vi "Q14070-Z060B111.vi"() -> ()   [LabVIEW 2013]
uses:
  <vilib>/Utility/file.llb/Read From Spreadsheet File (string).vi
  <vilib>/express/express arith-compare/Formula/XNode/ExpressFormulaBlockNode.xnode
  PCI8622_32.dll
  <vilib>/printing/EasyPrintingControls.llb/contents.ctl
  <vilib>/Utility/NIReport.llb/NI_ReportGenerationCore.lvlib
  <vilib>/printing/EasyPrintingControls.llb/report_type.ctl
  <vilib>/Utility/NIReport.llb/NI_report.lvclass
  <vilib>/printing/EasyPrinting.llb/Easy Print VI Panel or Documentation (path).vi
panel:
  out "左轴向力数组大小":i32
  in  "电动缸快速":dbl=15.0
  in  "电动缸慢速":dbl=1.0
  out "最大轴向力标准(N)":dbl=200.0 caption="L+Lmax(mm)" format="%#.3f"
  out "循环退出":bool
  in  "?":bool
  in  "密码":string
  in  "?":bool
  in  "?":bool
  in  "截取百分比":dbl=0.05
  in  "半行程":dbl=70.0
  in  "是否取消放行按钮":bool
  out "PLC":bool
  out "齿条传动比":dbl=200.0 caption="L+Lmax(mm)" format="%#.3f"
  out "右平均轴向力(N)":dbl caption="L+Lmax(mm)" format="%#.3f"
  out "左平均轴向力(N)":dbl caption="最大位移偏离Lmax(mm)" format="%#.3f"
  in  "确定按钮":bool
  out "员工ID":string
  in  "出支线工步号":dbl
  out "报警提示":string
  in  "报警工步号":dbl
  out "急停":bool
  out "DeviceHandle":u32
  in  "轴向力设定次数":dbl=5.0
  in  "最小间隙(mm)":dbl=0.0005 format="%#.3f"
  out "本备料状态H":bool
  out "本测试状态H":bool
  out "本自动状态H":bool
  out "夹头松开":bool
  out "测头右位":bool
  out "测头左位":bool
  in  "测头气缸右移":bool
  in  "测头气缸左移":bool
  in  "轴向力已做次数":dbl
  out "轴向力及全行程间隙合格":bool
  out "轴向力启动":bool
  out "间隙启动":bool
  out "夹头夹紧位":bool
  in  "夹头松开":bool
  in  "夹头夹紧":bool
  out "找帽扭矩":dbl=5.0 caption="压力传感器" format="%#.2f"
  out "error out":errorcluster
  out "型号数量":i32
  out "error out 4":errorcluster
  in  "间隙设定调整次数":dbl=5.0
  out "读取产品ID":string
  out "本备料状态":bool
  out "本测试状态":bool
  out "本自动状态":bool
  out "FGCS":string
  out "KSJJ":string
  out "Z060BRFID":string
  out "轴向力Y":dbl[](array[numeric])
  out "轴向力X":dbl[](array[numeric])
  out "间隙X数组":dbl[](array[numeric])
  out "间隙Y数组":dbl[](array[numeric])
  out "error out 3":errorcluster caption="错误输出"
  out "rfid工步号":u32
  out "芯片ID":string="201209190001"
  out "rfid完成":bool
  out "rfid触发":bool
  out "本序已做":bool
  in  "回零完成":bool
  in  "电动缸回零":bool
  in  "单点间隙已调试次数":dbl
  in  "需调整角度(度)":dbl
  in  "转向器中心":dbl
  out "扭矩到达":bool
  out "黄灯":bool
  out "红灯":bool
  out "基准位移":dbl caption="压力传感器" format="%#.4f"
  out "上序不合格":bool
  out "单点间隙合格":bool
  out "上序合格":bool
  out "测头机构电机":u32
  out "复位":bool
  in  "型号选择":u16(ring)=1 items=["J709", "J728", "J706"]
  in  "联线按钮":bool
  in  "工步号":u32
  in  "产品ID":string="201209190001"
  out "间隙位移(mm)":dbl=-4.6787895475327215 caption="压力传感器" format="%#.3f"
  out "齿条推拉力(N)":dbl format="%#.2f"
  out "齿条扭矩(Nm)":dbl format="%#.2f"
  out "通讯状态":bool
  out "员工姓名":string
  out "工步提示":string
  out "ADODB._Connection Out 2":refnum<k7>
  out "旋转齿条电机":u32
  out "电动缸电机":u32
  in  "停止":bool
  in  "参数加载":bool
  in  "选项卡控件":T1(tab)
  in  "180°外全行程间隙标准(mm)":dbl=0.1 format="%#.3f"
  out "扭动曲线":cluster{"Y":dbl[], "Y":dbl[]}[](graph) caption="压球涨堵头1"
  out "中间位置间隙":dbl caption="间隙值L(mm)" format="%#.3f"
  in  "中间位置最大间隙标准(mm)":dbl=0.07 format="%#.3f"
  out "右180°外全行程间隙":dbl caption="正向最大间隙L1(mm)" format="%#.3f"
  out "左180°外全行程间隙":dbl caption="正向最大间隙L1(mm)" format="%#.3f"
  out "右180°内全行程间隙":dbl caption="正向最大间隙L1(mm)" format="%#.3f"
  out "左180°内全行程间隙":dbl caption="正向最大间隙L1(mm)" format="%#.3f"
  in  "180°内全行程间隙标准(mm)":dbl=0.07 format="%#.3f"
  in  "找帽OK":bool
  out "左全行程间隙":dbl caption="正向最大间隙L1(mm)" format="%#.3f"
  out "右全行程间隙":dbl caption="正向最大间隙L1(mm)" format="%#.3f"
  out "总圈数最大值":dbl
  out "总圈数标准":dbl
  out "总行程最大值":dbl
  out "总行程标准(mm)":dbl
  out "力波动标准(N)":dbl=60.0 caption="L+Lmax(mm)" format="%#.3f"
  out "轴向力标准(N)":dbl=100.0 caption="L+Lmax(mm)" format="%#.3f"
  out "右轴向力波动(N)":dbl caption="L+Lmax(mm)" format="%_4g"
  out "右最大轴向力(N)":dbl caption="L+Lmax(mm)" format="%_4g"
  out "左轴向力波动(N)":dbl caption="最大位移偏离Lmax(mm)" format="%_4g"
  out "左最大轴向力(N)":dbl caption="最大位移偏离Lmax(mm)" format="%_4g"
  out "行程跳动曲线":cluster{"Y":dbl[], "Y":dbl[]}[](graph) caption="压球涨堵头1"
  out "平均轴向力标准(N) max":dbl=200.0 caption="L+Lmax(mm)" format="%#.3f"
  out "总行程":dbl format="%_4g"
  out "总圈数":dbl format="%_4g"
  in  "不合格品":bool
  in  "扭矩停止值":dbl=16.0
  in  "齿条右极限":dbl=-70.0 caption="压力传感器" format="%#.2f"
  in  "齿条左极限":dbl=-262.0 caption="压力传感器" format="%#.2f"
  in  "齿条移动速度":dbl=5.0 caption="压力传感器" format="%#.2f"
  in  "旋转齿条轴找帽转速":dbl=5.0 caption="压力传感器" format="%#.2f"
  in  "测量点扭矩":dbl=4.0 caption="压力传感器" format="%#.2f"
  in  "旋转齿条轴测量转速":dbl caption="压力传感器" format="%#.2f"
  in  "测头机构轴后退位":dbl=30.0 caption="压力传感器" format="%#.2f"
  in  "测头机构轴待检位":dbl caption="压力传感器" format="%#.2f"
  in  "测头机构轴检测位":dbl caption="压力传感器" format="%#.2f"
  in  "测头机构轴移动速度":dbl caption="压力传感器" format="%#.2f"
  in  "机械间隙值":dbl=3.5
  in  "阻挡":bool
  in  "放行":bool
  in  "夹头松开":bool
  in  "夹头夹紧":bool
  in  "测头气缸右移":bool
  in  "测头气缸左移":bool
  in  "支线下降":bool
  in  "支线顶升":bool
  in  "出支线":bool
  in  "进支线":bool
  in  "主线下降":bool
  in  "主线顶升":bool
  in  "下阻挡器放行":bool
  in  "上阻挡器放行":bool
  in  "测头机构轴使能":bool
  in  "测头机构轴后退":bool
  in  "测头机构轴前进":bool
  in  "电动缸速度(mm/s)":dbl=10.0 format="%#.3f"
  out "电动缸位置(mm)":dbl format="%#.3f"
  in  "旋转齿条轴速度(°/s)":dbl=10.0 format="%#.3f"
  out "旋转齿条轴位置(°)":dbl format="%#.3f"
  in  "测头机构轴速度(mm/s)":dbl=10.0 format="%#.3f"
  out "测头机构轴位置(mm)":dbl format="%#.3f"
  in  "旋转齿条轴右转":bool
  in  "旋转齿条轴左转":bool
  in  "旋转齿条轴使能":bool
  in  "电动缸后退":bool
  in  "电动缸使能":bool
  in  "电动缸前进":bool
  in  "齿条扭矩比例偏移":dbl=1.0 format="%#.2f"
  in  "齿条扭矩零点偏移":dbl format="%#.2f"
  in  "齿条推拉力比例偏移":dbl=1.0 format="%#.2f"
  in  "齿条推拉力零点偏移":dbl format="%#.2f"
  in  "间隙位移比例偏移":dbl=1.0 format="%#.2f"
  in  "间隙位移零点偏移":dbl format="%#.2f"
  in  "传感器参数保存":bool
  in  "参数修改":bool
  in  "参数查询":bool
  in  "参数浏览表":string[][](table)
  # "芜湖机械转向器装配线"
  # "间隙及轴向力检测"
  # "湖北唯思凌科装备制造有限公司 设计开发 (C)2015"
  # "Q14070机械转向器装配线"
  # "≤"
  # "间隙测量结果"
  # "间隙测量判定值"
  # "≤"
  # "≤"
  # "≤"
  # "轴向力测量结果"
  # "轴向力测量标准"
  # "≥"
  # "≤"
  # "≥"
  # "≤"
  # "≤"
  # "≥"
  # "不得大于20NM"
  # "传感器校验区"
  # "关于传感器校验：\n1、传感器校验需要由具备资质的单位或部门进行校验。\n2、具备权限的用户才能够修改传感器校验参数和试验参数。\n3、修改校验参数方法：先将比例偏移置为1，修改零点偏移，使零点值与校验的传感器一致；然后根据增幅调整比例偏移。"
  # "注意：\n具备权限的用户才能够修改传感器校验参数和试验参数！"
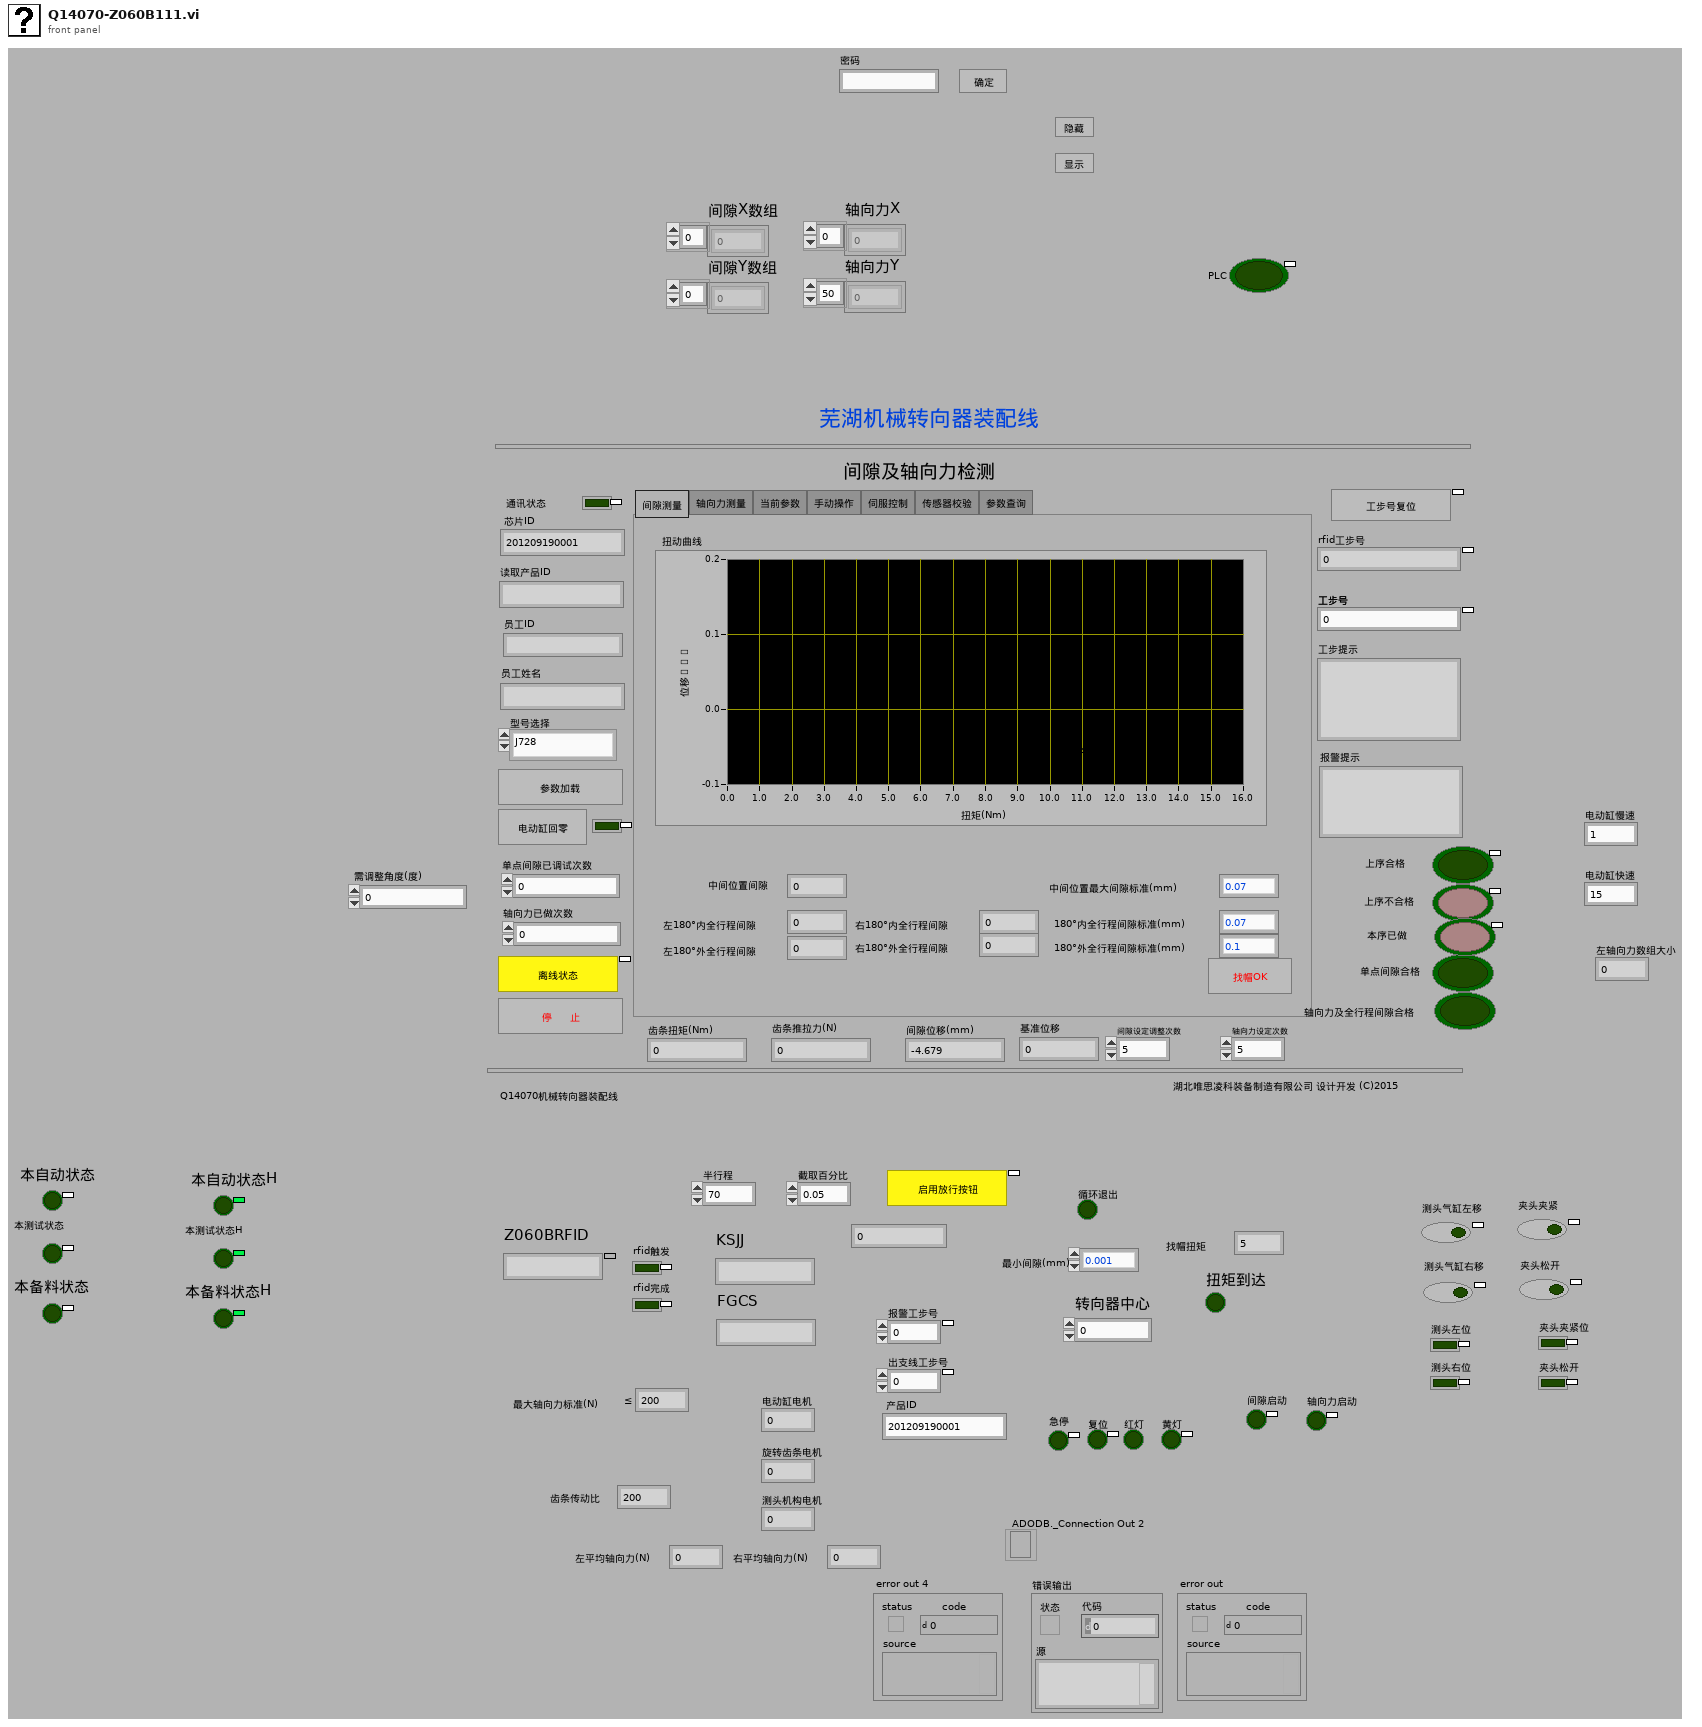
[diagram p1: front panel]
types:
  T1 = enum32{"间隙测量", "轴向力测量", "当前参数", "手动操作", "伺服控制", "传感器校验", "参数查询"}
  T2 = typedef "NI_ReportGenerationCore.lvlib/report_type.ctl" = u16
  T3 = typedef "NI_ReportGenerationCore.lvlib/contents.ctl" = u16
  T4 = typedef "imagedata.ctl" = cluster{"image type":i32, "image depth":i32, "image":u8[], "mask":u8[], "colors":u32[], "Rectangle":cluster{"left":i16, "top":i16, "right":i16, "bottom":i16}}
  T5 = enum8{"Enabled", "Disabled", "Disabled and Grayed Out"}
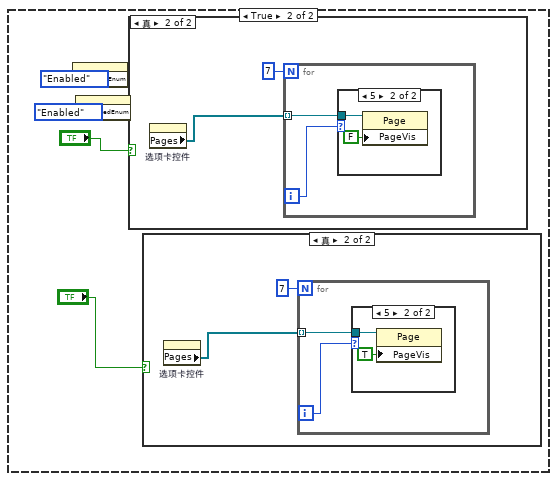
[diagram p2: hidden frame]
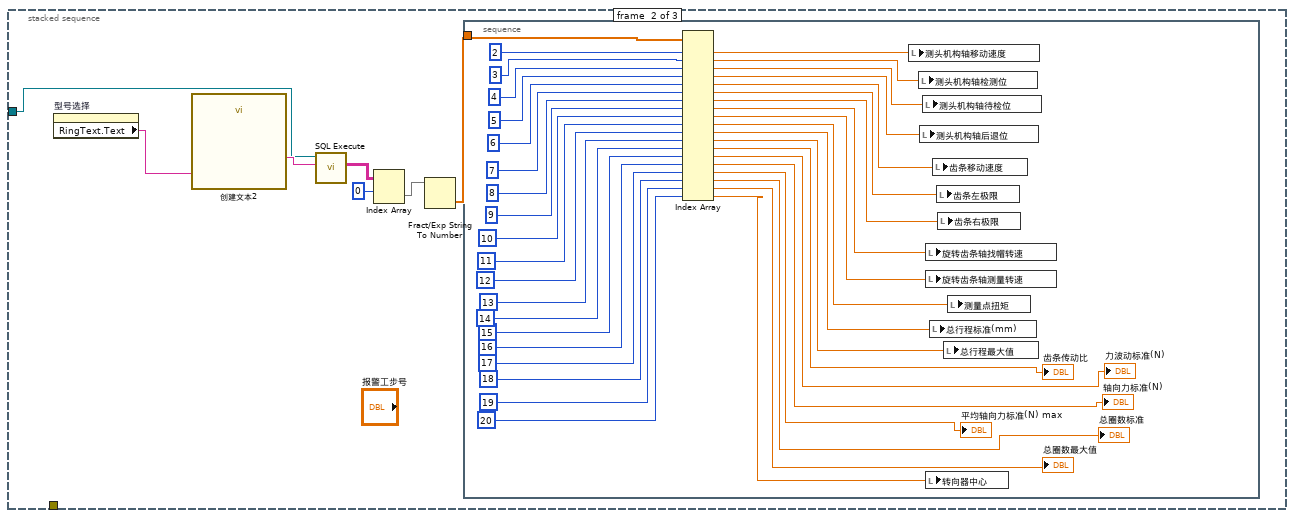
[diagram p9: hidden frame]
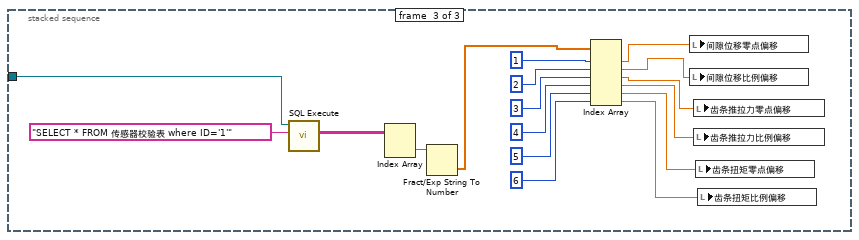
[diagram p10: hidden frame]
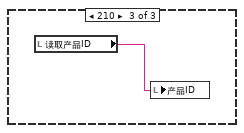
[diagram p12: hidden frame]
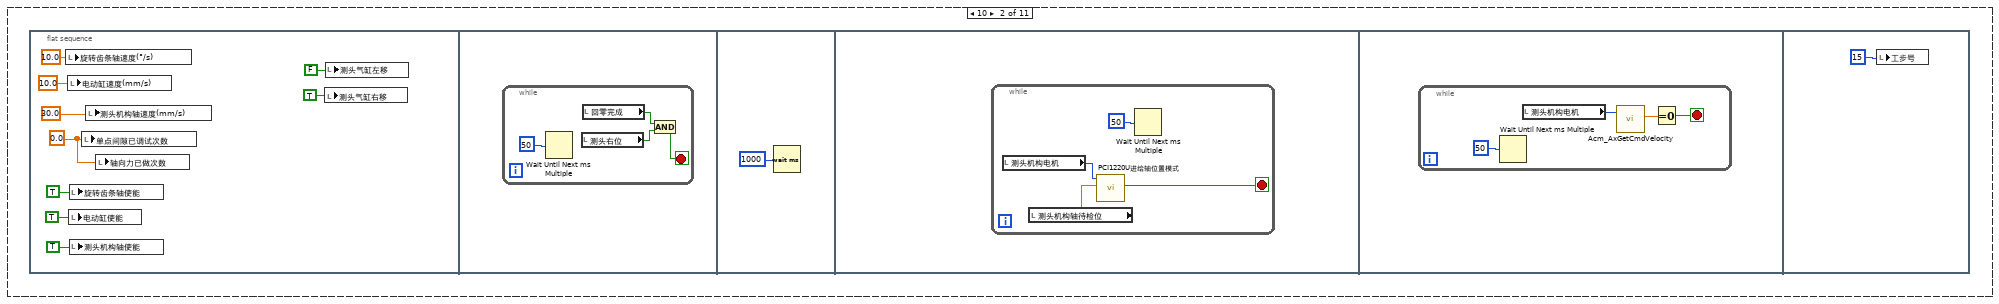
[diagram p14: hidden frame]
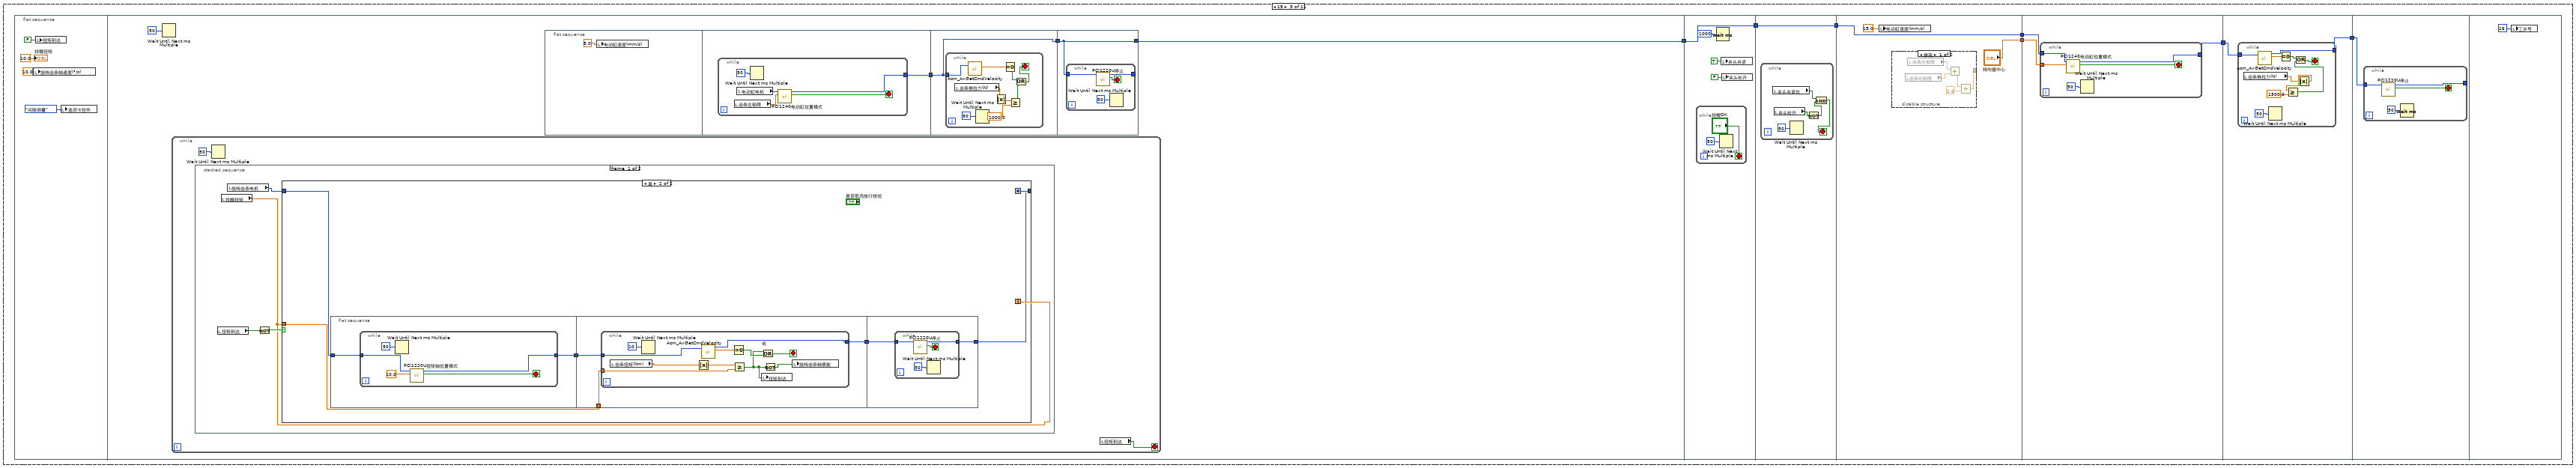
[diagram p15: hidden frame]
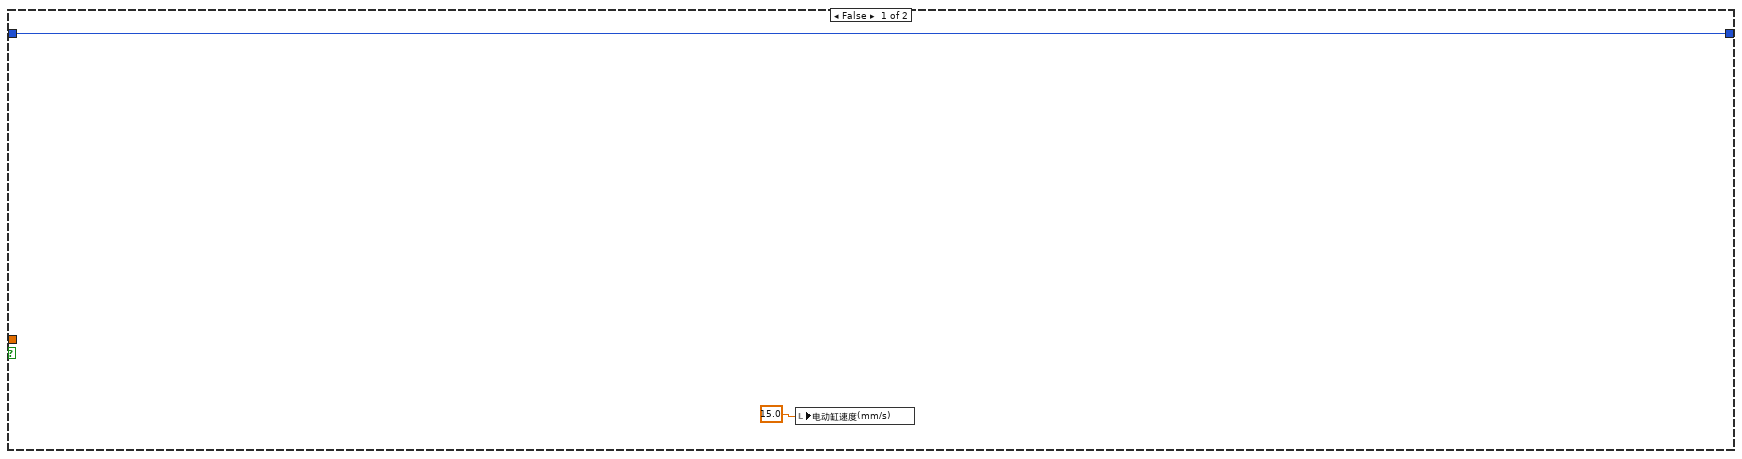
[diagram p16: hidden frame]
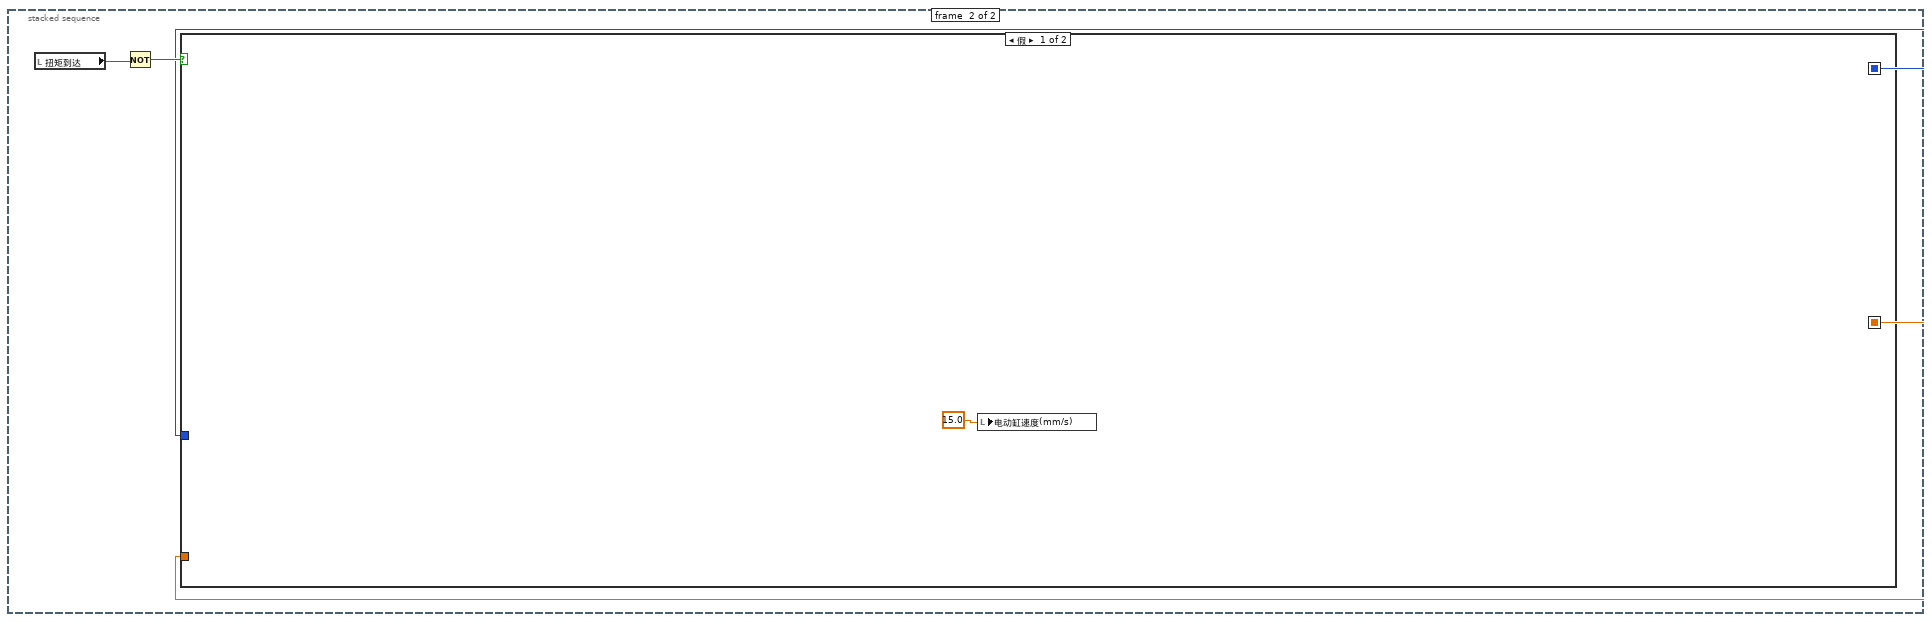
[diagram p17: hidden frame]
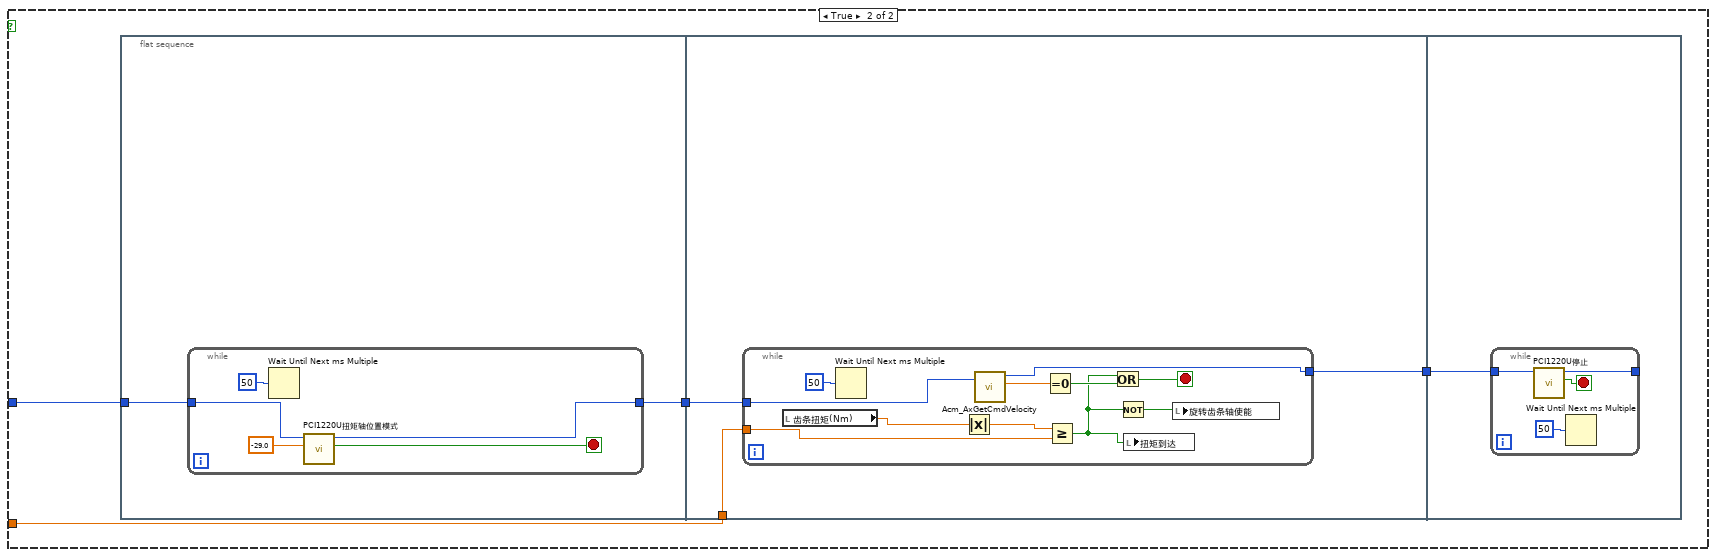
[diagram p18: hidden frame]
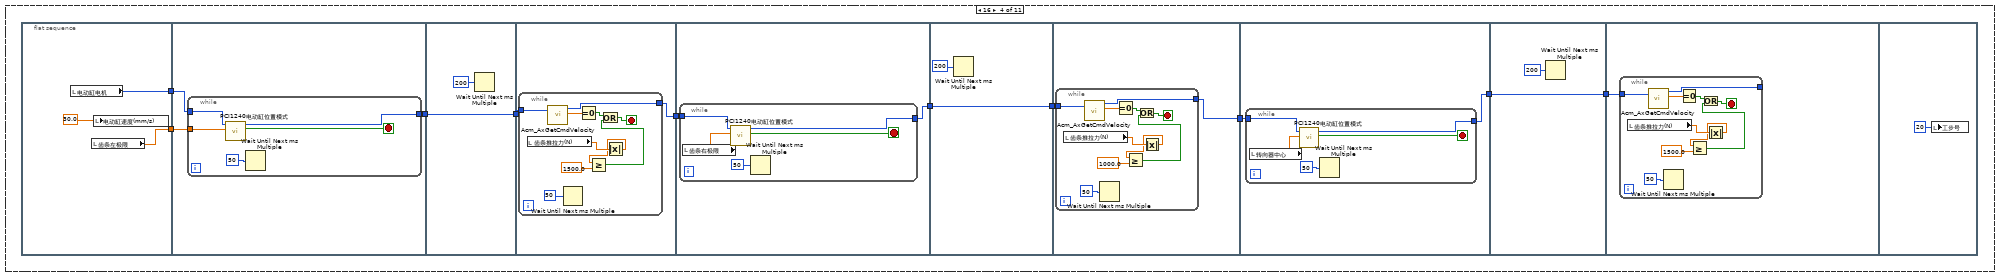
[diagram p20: hidden frame]
diagram:
  n1 = while {
    stop <- w7 stop-if-true
    n2 = local read "工步号"() -> (w5:u32)
    n3 = case shown="40" w5 {
      frame 0, Default {
      }
      frame 10 {
        n4 = flat-sequence {
          frame #0 {
            w8 = 0.0 ("已调试次数")
            n5 = local write "旋转齿条轴速度(°/s)"(10.0 ("旋转齿条轴速度(°/s)")) -> ()
            n6 = local write "电动缸速度(mm/s)"(10.0 ("电动缸速度(mm/s)")) -> ()
            n7 = local write "电动缸使能"(TRUE ("电动缸使能")) -> ()
            n8 = local write "旋转齿条轴使能"(TRUE ("旋转齿条轴使能")) -> ()
            n9 = local write "测头机构轴使能"(TRUE ("调整机构轴使能")) -> ()
            n10 = local write "单点间隙已调试次数"(w8) -> ()
            n11 = local write "测头机构轴速度(mm/s)"(30.0 ("调整机构轴速度(mm/s)")) -> ()
            n12 = local write "轴向力已做次数"(w8) -> ()
            n13 = local write "测头气缸右移"(TRUE ("测头气缸右移")) -> ()
            n14 = local write "测头气缸左移"(FALSE ("测头气缸左移")) -> ()
          }
          frame #1 {
            n15 = while {
              stop <- w17 stop-if-true
              n16 = Wait Until Next ms Multiple(millisecond multiple=u32 50 ("毫秒倍数")) -> ()  [unwired: 1 out]
              n17 = local read "测头右位"() -> (w18:bool)
              n18 = local read "回零完成"() -> (w19:bool)
              n19 = And(x=w19, y=w18) -> (x .and. y?=w17:bool)
            }
          }
          frame #2 {
            n20 = Wait (ms)(milliseconds to wait=u32 1000 ("等待时间（毫秒）")) -> ()  [unwired: 1 out]
          }
          frame #3 {
            n21 = while {
              stop <- w25 stop-if-true
              n22 = local read "测头机构电机"() -> (w23:u32)
              n23 = local read "测头机构轴待检位"() -> (w22:dbl)
              n24 = call "PCI1220U进给轴位置模式.vi"("Distance"=w22, "AxisHandle IN"=w23) -> ("AbsSuccess"=w25:bool)  [unwired: 8 in, 1 out]
              n25 = Wait Until Next ms Multiple(millisecond multiple=u32 50 ("毫秒倍数")) -> ()  [unwired: 1 out]
            }
          }
          frame #4 {
            n26 = while {
              stop <- w28 stop-if-true
              n27 = Wait Until Next ms Multiple(millisecond multiple=u32 50 ("毫秒倍数")) -> ()  [unwired: 1 out]
              n28 = local read "测头机构电机"() -> (w26:u32)
              n29 = call <userlib>:"Acm_AxGetCmdVelocity.vi"("AxisHandle"=w26) -> ("Velocity"=w29:dbl)  [unwired: 1 in, 3 out]
              n30 = Equal To 0?(x=w29) -> (x = 0?=w28:bool)
            }
          }
          frame #5 {
            n31 = local write "工步号"(u32 15 ("工步号")) -> ()
          }
        }
      }
      frame 15 {
        n32 = flat-sequence {
          tunnel: [w43] -> w34
          tunnel: w34 -> [w146]
          tunnel: [w146] -> w32
          tunnel: w32 -> [w150]
          tunnel: [w150] -> w31
          tunnel: [w157] -> w37
          tunnel: ["转向器中心"] -> w36
          tunnel: w31 -> [w157]
          tunnel: w37 -> [w166]
          tunnel: w36 -> [w165]
          tunnel: [w164] -> w35
          tunnel: w35 -> [w173]
          tunnel: [w172] -> w33
          tunnel: w33 -> [w184]
          frame #0 {
            n33 = local write "旋转齿条轴速度(°/s)"(10.0 ("旋转齿条轴速度(°/s)")) -> ()
            n34 = local write "扭矩到达"(FALSE ("扭矩到达")) -> ()
            n35 = local write "选项卡控件"(T1."间隙测量" ("选项卡控件")) -> ()
            "找帽扭矩" <- 10.0 ("找帽扭矩")
          }
          frame #1 {
            n36 = Wait Until Next ms Multiple(millisecond multiple=u32 50 ("毫秒倍数")) -> ()  [unwired: 1 out]
            n37 = while {
              stop <- w46 stop-if-true
              n38 = stacked-sequence {
                seq-local: [w48 _] -> [_ w89]
                seq-local: [w52 _] -> [_ w88]
                frame #0 {
                  n39 = local read "扭矩到达"() -> (w50:bool)
                  n40 = local read "找帽扭矩"() -> (w48:dbl)
                  n41 = local read "旋转齿条电机"() -> (w49:u32)
                  n42 = Not(x=w50) -> (.not. x?=w51:bool)
                  n43 = case shown="真" w51 {
                    tunnel: [w54 w55] -> w52
                    tunnel: w49 -> [w54 w59]
                    tunnel: w48 -> [_ w57]
                    frame False {
                      n44 = local write "电动缸速度(mm/s)"(15.0 ("电动缸速度(mm/s)")) -> ()
                    }
                    frame True {
                      n45 = flat-sequence {
                        tunnel: w59 -> [w61]
                        tunnel: [w60] -> w58
                        tunnel: w58 -> [w69]
                        tunnel: w57 -> [w68]
                        tunnel: [w67] -> w56
                        tunnel: w56 -> [w82]
                        tunnel: [w81] -> w55
                        frame #0 {
                          n46 = while {
                            tunnel: [w65] -> w60
                            tunnel: w61 -> [w62]
                            stop <- w64 stop-if-true
                            n47 = Wait Until Next ms Multiple(millisecond multiple=u32 50 ("毫秒倍数")) -> ()  [unwired: 1 out]
                            n48 = call "PCI1220U扭矩轴位置模式.vi"("Distance"=10.0, "AxisHandle IN"=w62) -> ("AbsSuccess"=w64:bool, "AxisHandle OUT"=w65:u32)  [unwired: 8 in]
                          }
                        }
                        frame #1 {
                          n49 = while {
                            tunnel: w69 -> [w79]
                            tunnel: w68 -> [w74]
                            tunnel: [w73] -> w67
                            stop <- w75 stop-if-true
                            n50 = local read "齿条扭矩(Nm)"() -> (w72:dbl)
                            n51 = Wait Until Next ms Multiple(millisecond multiple=u32 10 ("毫秒倍数")) -> ()  [unwired: 1 out]
                            n52 = Absolute Value(x=w72) -> (abs(x)=w77:dbl)
                            n53 = call <userlib>:"Acm_AxGetCmdVelocity.vi"("AxisHandle"=w79) -> ("Velocity"=w78:dbl, "AxisHandle"=w73:u32)  [unwired: 1 in, 2 out]
                            n54 = Equal To 0?(x=w78) -> (x = 0?=w76:bool)
                            n55 = Greater Or Equal?(x=w77, y=w74) -> (x >= y?=w71:bool)
                            n56 = Or "或"(x=w71, y=w76) -> (x .or. y?=w75:bool)
                            n57 = local write "扭矩到达"(w71) -> ()
                            n58 = Not(x=w71) -> (.not. x?=w70:bool)
                            n59 = local write "旋转齿条轴使能"(w70) -> ()
                          }
                        }
                        frame #2 {
                          n60 = while {
                            tunnel: w82 -> [w86]
                            tunnel: [w83] -> w81
                            stop <- w85 stop-if-true
                            n61 = call "PCI1220U停止.vi"("AxisHandle IN"=w86) -> ("完成"=w85:bool, "AxisHandle OUT"=w83:u32)  [unwired: 9 in]
                            n62 = Wait Until Next ms Multiple(millisecond multiple=u32 50 ("毫秒倍数")) -> ()  [unwired: 1 out]
                          }
                        }
                      }
                    }
                  }
                }
                frame #1 {
                  n63 = local read "扭矩到达"() -> (w87:bool)
                  n64 = Not(x=w87) -> (.not. x?=w90:bool)
                  n65 = case shown="假" w90 {
                    tunnel: w88 -> [_ w95]
                    tunnel: w89 -> [_ w93]
                    frame False {
                      n66 = local write "电动缸速度(mm/s)"(15.0 ("电动缸速度(mm/s)")) -> ()
                    }
                    frame True {
                      n67 = flat-sequence {
                        tunnel: w95 -> [w96]
                        tunnel: [w97] -> w94
                        tunnel: w94 -> [w105]
                        tunnel: w93 -> [w104]
                        tunnel: [w103] -> w92
                        tunnel: w92 -> [w117]
                        frame #0 {
                          n68 = while {
                            tunnel: [w101] -> w97
                            tunnel: w96 -> [w98]
                            stop <- w100 stop-if-true
                            n69 = Wait Until Next ms Multiple(millisecond multiple=u32 50 ("毫秒倍数")) -> ()  [unwired: 1 out]
                            n70 = call "PCI1220U扭矩轴位置模式.vi"("Distance"=-29.0, "AxisHandle IN"=w98) -> ("AbsSuccess"=w100:bool, "AxisHandle OUT"=w101:u32)  [unwired: 8 in]
                          }
                        }
                        frame #1 {
                          n71 = while {
                            tunnel: w105 -> [w115]
                            tunnel: [w110] -> w103
                            tunnel: w104 -> [w109]
                            stop <- w111 stop-if-true
                            n72 = local read "齿条扭矩(Nm)"() -> (w108:dbl)
                            n73 = Wait Until Next ms Multiple(millisecond multiple=u32 50 ("毫秒倍数")) -> ()  [unwired: 1 out]
                            n74 = Absolute Value(x=w108) -> (abs(x)=w113:dbl)
                            n75 = call <userlib>:"Acm_AxGetCmdVelocity.vi"("AxisHandle"=w115) -> ("Velocity"=w114:dbl, "AxisHandle"=w110:u32)  [unwired: 1 in, 2 out]
                            n76 = Equal To 0?(x=w114) -> (x = 0?=w112:bool)
                            n77 = Greater Or Equal?(x=w113, y=w109) -> (x >= y?=w106:bool)
                            n78 = Or(x=w106, y=w112) -> (x .or. y?=w111:bool)
                            n79 = Not(x=w106) -> (.not. x?=w107:bool)
                            n80 = local write "扭矩到达"(w106) -> ()
                            n81 = local write "旋转齿条轴使能"(w107) -> ()
                          }
                        }
                        frame #2 {
                          n82 = while {
                            tunnel: w117 -> [w121]
                            tunnel: [w118] -> _
                            stop <- w120 stop-if-true
                            n83 = call "PCI1220U停止.vi"("AxisHandle IN"=w121) -> ("完成"=w120:bool, "AxisHandle OUT"=w118:u32)  [unwired: 9 in]
                            n84 = Wait Until Next ms Multiple(millisecond multiple=u32 50 ("毫秒倍数")) -> ()  [unwired: 1 out]
                          }
                        }
                      }
                    }
                  }
                }
              }
              n85 = Wait Until Next ms Multiple(millisecond multiple=u32 50 ("毫秒倍数")) -> ()  [unwired: 1 out]
              n86 = local read "扭矩到达"() -> (w46:bool)
            }
            n87 = flat-sequence {
              tunnel: [w123] -> w45
              tunnel: w45 -> [w129]
              tunnel: [w129] -> w42
              tunnel: [w139] -> w43
              tunnel: w42 -> [w139]
              frame #0 {
                n88 = local write "电动缸速度(mm/s)"(5.0 ("电动缸速度(mm/s)")) -> ()
              }
              frame #1 {
                n89 = while {
                  tunnel: [w127] -> w123
                  stop <- w126 stop-if-true
                  n90 = local read "齿条左极限"() -> (w124:dbl)
                  n91 = local read "电动缸电机"() -> (w128:u32)
                  n92 = Wait Until Next ms Multiple(millisecond multiple=u32 50 ("毫秒倍数")) -> ()  [unwired: 1 out]
                  n93 = call "PCI1240电动缸位置模式 .vi"("Distance"=w124, "AxisHandle IN"=w128) -> ("AbsSuccess"=w126:bool, "AxisHandle OUT"=w127:u32)  [unwired: 8 in]
                }
              }
              frame #2 {
                n94 = while {
                  tunnel: w129 -> [w137]
                  stop <- w134 stop-if-true
                  n95 = local read "齿条推拉力(N)"() -> (w133:dbl)
                  n96 = call <userlib>:"Acm_AxGetCmdVelocity.vi"("AxisHandle"=w137) -> ("Velocity"=w138:dbl)  [unwired: 1 in, 3 out]
                  n97 = Wait Until Next ms Multiple(millisecond multiple=u32 50 ("毫秒倍数")) -> ()  [unwired: 1 out]
                  n98 = Absolute Value(x=w133) -> (abs(x)=w130:dbl)
                  n99 = Equal To 0?(x=w138) -> (x = 0?=w135:bool)
                  n100 = Greater Or Equal?(x=w130, y=1000.0) -> (x >= y?=w131:bool)
                  n101 = Or(x=w135, y=w131) -> (x .or. y?=w134:bool)
                }
              }
              frame #3 {
                n102 = while {
                  tunnel: w139 -> [w143]
                  tunnel: [w140] -> _
                  stop <- w142 stop-if-true
                  n103 = call "PCI1220U停止.vi"("AxisHandle IN"=w143) -> ("完成"=w142:bool, "AxisHandle OUT"=w140:u32)  [unwired: 9 in]
                  n104 = Wait Until Next ms Multiple(millisecond multiple=u32 50 ("毫秒倍数")) -> ()  [unwired: 1 out]
                }
              }
            }
          }
          frame #2 {
            n105 = while {
              stop <- "找帽OK" stop-if-true
              n106 = Wait Until Next ms Multiple(millisecond multiple=u32 50 ("毫秒倍数")) -> ()  [unwired: 1 out]
            }
            n107 = Wait (ms)(milliseconds to wait=u32 1000 ("毫秒倍数")) -> ()  [unwired: 1 out]
            n108 = local write "夹头夹紧"(TRUE ("夹头夹紧")) -> ()
            n109 = local write "夹头松开"(FALSE ("夹头松开")) -> ()
          }
          frame #3 {
            n110 = while {
              stop <- w152 stop-if-true
              n111 = local read "夹头夹紧位"() -> (w153:bool)
              n112 = local read "夹头松开"() -> (w155:bool)
              n113 = Wait Until Next ms Multiple(millisecond multiple=u32 50 ("毫秒倍数")) -> ()  [unwired: 1 out]
              n114 = Not(x=w155) -> (.not. x?=w154:bool)
              n115 = And(x=w153, y=w154) -> (x .and. y?=w152:bool)
            }
          }
          frame #4 {
            n116 = local write "电动缸速度(mm/s)"(15.0 ("电动缸轴移动速度")) -> ()
            n117 = disable-structure shown="禁用" {
              disable-tunnel: [w159 _] -> _
              frame Disabled {
                n118 = local read "齿条右极限"() -> (w162:dbl)
                n119 = local read "齿条左极限"() -> (w163:dbl)
                n120 = Add(x=w163, y=w162) -> (x+y=w161:dbl)
                n121 = Divide(x=w161, y=2.0) -> (x/y=w159:dbl)
              }
              frame Enabled {
              }
            }
          }
          frame #5 {
            n122 = while {
              tunnel: w166 -> [w171]
              tunnel: w165 -> [w170]
              tunnel: [w167] -> w164
              stop <- w169 stop-if-true
              n123 = call "PCI1240电动缸位置模式 .vi"("Distance"=w170, "AxisHandle IN"=w171) -> ("AbsSuccess"=w169:bool, "AxisHandle OUT"=w167:u32)  [unwired: 8 in]
              n124 = Wait Until Next ms Multiple(millisecond multiple=u32 50 ("毫秒倍数")) -> ()  [unwired: 1 out]
            }
          }
          frame #6 {
            n125 = while {
              tunnel: w173 -> [w183]
              tunnel: [w174] -> w172
              stop <- w175 stop-if-true
              n126 = local read "齿条推拉力(N)"() -> (w180:dbl)
              n127 = call <userlib>:"Acm_AxGetCmdVelocity.vi"("AxisHandle"=w183) -> ("Velocity"=w182:dbl, "AxisHandle"=w174:u32)  [unwired: 1 in, 2 out]
              n128 = Wait Until Next ms Multiple(millisecond multiple=u32 50 ("毫秒倍数")) -> ()  [unwired: 1 out]
              n129 = Equal To 0?(x=w182) -> (x = 0?=w177:bool)
              n130 = Absolute Value(x=w180) -> (abs(x)=w179:dbl)
              n131 = Greater Or Equal?(x=w179, y=1500.0) -> (x >= y?=w176:bool)
              n132 = Or(x=w177, y=w176) -> (x .or. y?=w175:bool)
            }
          }
          frame #7 {
            n133 = while {
              tunnel: w184 -> [w188]
              tunnel: [w187] -> _
              stop <- w186 stop-if-true
              n134 = call "PCI1220U停止.vi"("AxisHandle IN"=w188) -> ("完成"=w186:bool, "AxisHandle OUT"=w187:u32)  [unwired: 9 in]
              n135 = Wait (ms)(milliseconds to wait=u32 50 ("毫秒倍数")) -> ()  [unwired: 1 out]
            }
          }
          frame #8 {
            n136 = local write "工步号"(u32 16 ("工步号")) -> ()
          }
        }
      }
      frame 16 {
        n137 = flat-sequence {
          tunnel: [w202] -> w199
          tunnel: [w201] -> w198
          tunnel: w199 -> [w205]
          tunnel: w198 -> [w204]
          tunnel: [w203] -> w197
          tunnel: w197 -> [w212]
          tunnel: [w212] -> w196
          tunnel: w196 -> [w214]
          tunnel: [w213] -> w195
          tunnel: w195 -> [w226]
          tunnel: [w225] -> w193
          tunnel: [w232] -> w194
          tunnel: w193 -> [w232]
          tunnel: w194 -> [w235]
          tunnel: [w234] -> w192
          tunnel: w192 -> [w247]
          tunnel: [w246] -> w190
          tunnel: [w253] -> w191
          tunnel: w190 -> [w253]
          tunnel: w191 -> [w255]
          frame #0 {
            n138 = local read "电动缸电机"() -> (w202:u32)
            n139 = local read "齿条左极限"() -> (w201:dbl)
            n140 = local write "电动缸速度(mm/s)"(30.0 ("齿条移动速度")) -> ()
          }
          frame #1 {
            n141 = while {
              tunnel: w205 -> [w210]
              tunnel: w204 -> [w209]
              tunnel: [w206] -> w203
              stop <- w208 stop-if-true
              n142 = call "PCI1240电动缸位置模式 .vi"("Distance"=w209, "AxisHandle IN"=w210) -> ("AbsSuccess"=w208:bool, "AxisHandle OUT"=w206:u32)  [unwired: 8 in]
              n143 = Wait Until Next ms Multiple(millisecond multiple=u32 50 ("毫秒倍数")) -> ()  [unwired: 1 out]
            }
          }
          frame #2 {
            n144 = Wait Until Next ms Multiple(millisecond multiple=u32 200 ("毫秒倍数")) -> ()  [unwired: 1 out]
          }
          frame #3 {
            n145 = while {
              tunnel: w214 -> [w224]
              tunnel: [w215] -> w213
              stop <- w216 stop-if-true
              n146 = local read "齿条推拉力(N)"() -> (w221:dbl)
              n147 = call <userlib>:"Acm_AxGetCmdVelocity.vi"("AxisHandle"=w224) -> ("Velocity"=w223:dbl, "AxisHandle"=w215:u32)  [unwired: 1 in, 2 out]
              n148 = Wait Until Next ms Multiple(millisecond multiple=u32 50 ("毫秒倍数")) -> ()  [unwired: 1 out]
              n149 = Equal To 0?(x=w223) -> (x = 0?=w218:bool)
              n150 = Absolute Value(x=w221) -> (abs(x)=w220:dbl)
              n151 = Greater Or Equal?(x=w220, y=1500.0) -> (x >= y?=w217:bool)
              n152 = Or(x=w218, y=w217) -> (x .or. y?=w216:bool)
            }
          }
          frame #4 {
            n153 = while {
              tunnel: w226 -> [w231]
              tunnel: [w228] -> w225
              stop <- w230 stop-if-true
              n154 = local read "齿条右极限"() -> (w227:dbl)
              n155 = call "PCI1240电动缸位置模式 .vi"("Distance"=w227, "AxisHandle IN"=w231) -> ("AbsSuccess"=w230:bool, "AxisHandle OUT"=w228:u32)  [unwired: 8 in]
              n156 = Wait Until Next ms Multiple(millisecond multiple=u32 50 ("毫秒倍数")) -> ()  [unwired: 1 out]
            }
          }
          frame #5 {
            n157 = Wait Until Next ms Multiple(millisecond multiple=u32 200 ("毫秒倍数")) -> ()  [unwired: 1 out]
          }
          frame #6 {
            n158 = while {
              tunnel: w235 -> [w245]
              tunnel: [w236] -> w234
              stop <- w237 stop-if-true
              n159 = local read "齿条推拉力(N)"() -> (w242:dbl)
              n160 = call <userlib>:"Acm_AxGetCmdVelocity.vi"("AxisHandle"=w245) -> ("Velocity"=w244:dbl, "AxisHandle"=w236:u32)  [unwired: 1 in, 2 out]
              n161 = Wait Until Next ms Multiple(millisecond multiple=u32 50 ("毫秒倍数")) -> ()  [unwired: 1 out]
              n162 = Equal To 0?(x=w244) -> (x = 0?=w239:bool)
              n163 = Absolute Value(x=w242) -> (abs(x)=w241:dbl)
              n164 = Greater Or Equal?(x=w241, y=1000.0) -> (x >= y?=w238:bool)
              n165 = Or(x=w239, y=w238) -> (x .or. y?=w237:bool)
            }
          }
          frame #7 {
            n166 = while {
              tunnel: w247 -> [w252]
              tunnel: [w249] -> w246
              stop <- w251 stop-if-true
              n167 = local read "转向器中心"() -> (w248:dbl)
              n168 = call "PCI1240电动缸位置模式 .vi"("Distance"=w248, "AxisHandle IN"=w252) -> ("AbsSuccess"=w251:bool, "AxisHandle OUT"=w249:u32)  [unwired: 8 in]
              n169 = Wait Until Next ms Multiple(millisecond multiple=u32 50 ("毫秒倍数")) -> ()  [unwired: 1 out]
            }
          }
          frame #8 {
            n170 = Wait Until Next ms Multiple(millisecond multiple=u32 200 ("毫秒倍数")) -> ()  [unwired: 1 out]
          }
          frame #9 {
            n171 = while {
              tunnel: w255 -> [w265]
              tunnel: [w256] -> _
              stop <- w257 stop-if-true
              n172 = local read "齿条推拉力(N)"() -> (w262:dbl)
              n173 = call <userlib>:"Acm_AxGetCmdVelocity.vi"("AxisHandle"=w265) -> ("Velocity"=w264:dbl, "AxisHandle"=w256:u32)  [unwired: 1 in, 2 out]
              n174 = Wait Until Next ms Multiple(millisecond multiple=u32 50 ("毫秒倍数")) -> ()  [unwired: 1 out]
              n175 = Equal To 0?(x=w264) -> (x = 0?=w259:bool)
              n176 = Absolute Value(x=w262) -> (abs(x)=w261:dbl)
              n177 = Greater Or Equal?(x=w261, y=1500.0) -> (x >= y?=w258:bool)
              n178 = Or(x=w259, y=w258) -> (x .or. y?=w257:bool)
            }
          }
          frame #10 {
            n179 = local write "工步号"(u32 20 ("工步号")) -> ()
          }
        }
      }
      frame 20 {
        n180 = flat-sequence {
          tunnel: [w295] -> w276
          tunnel: w276 -> [w301]
          tunnel: [w308] -> w272
          tunnel: w272 -> [w315]
          tunnel: [w315] -> w271
          tunnel: w271 -> [w323]
          tunnel: [w323] -> w270
          tunnel: w270 -> [w324]
          tunnel: [w330] -> w274
          tunnel: [w332] -> w275
          tunnel: w274 -> [w332]
          tunnel: [w334] -> w281
          tunnel: w275 -> [w334]
          tunnel: w281 -> [w341]
          tunnel: [w340] -> w280
          tunnel: [w345] -> w279
          tunnel: [w344] -> w278
          tunnel: w280 -> [w343]
          tunnel: [w343] -> w277
          tunnel: [w372] -> w284
          tunnel: [w369] -> w283
          tunnel: w279 -> [w369]
          tunnel: [w368] -> w282
          tunnel: w278 -> [w368]
          tunnel: w277 -> [w372]
          tunnel: w284 -> [w376]
          tunnel: [w375] -> w273
          tunnel: w283 -> [w373]
          tunnel: w282 -> [w374]
          tunnel: w273 -> [w382]
          tunnel: [w381] -> w268
          tunnel: w268 -> [w389]
          tunnel: [w389] -> w267
          tunnel: w267 -> [w391]
          tunnel: [w390] -> w269
          tunnel: w269 -> [w401]
          frame #0 {
            n181 = local write "选项卡控件"(T1."间隙测量" ("选项卡控件")) -> ()
          }
          frame #1 {
            n182 = while {
              stop <- w286 stop-if-true
              n183 = local read "夹头松开"() -> (w288:bool)
              n184 = local read "夹头夹紧位"() -> (w287:bool)
              n185 = Wait Until Next ms Multiple(millisecond multiple=u32 50 ("毫秒倍数")) -> ()  [unwired: 1 out]
              n186 = Not(x=w288) -> (.not. x?=w289:bool)
              n187 = And(x=w287, y=w289) -> (x .and. y?=w286:bool)
            }
          }
          frame #2 {
            n188 = local read "转向器中心"() -> (w291:dbl)
            n189 = local read "电动缸电机"() -> (w294:u32)
            n190 = Add(x=w291, y=0.0) -> (x+y=w293:dbl)
            n191 = while {
              tunnel: w294 -> [w300]
              tunnel: w293 -> [w299]
              tunnel: [w296] -> w295
              stop <- w298 stop-if-true
              n192 = call "PCI1240电动缸位置模式 .vi"("Distance"=w299, "AxisHandle IN"=w300) -> ("AbsSuccess"=w298:bool, "AxisHandle OUT"=w296:u32)  [unwired: 8 in]
              n193 = Wait Until Next ms Multiple(millisecond multiple=u32 50 ("毫秒倍数")) -> ()  [unwired: 1 out]
            }
          }
          frame #3 {
            n194 = while {
              tunnel: w301 -> [w305]
              stop <- w303 stop-if-true
              n195 = call <userlib>:"Acm_AxGetCmdVelocity.vi"("AxisHandle"=w305) -> ("Velocity"=w304:dbl)  [unwired: 1 in, 3 out]
              n196 = Wait Until Next ms Multiple(millisecond multiple=u32 50 ("毫秒倍数")) -> ()  [unwired: 1 out]
              n197 = Equal To 0?(x=w304) -> (x = 0?=w303:bool)
            }
          }
          frame #4 {
            n198 = local write "测头机构轴速度(mm/s)"(30.0 ("测头机构轴速度(mm/s)")) -> ()
          }
          frame #5 {
            n199 = local read "测头机构电机"() -> (w309:u32)
            n200 = local read "测头机构轴检测位"() -> (w307:dbl)
            n201 = while {
              tunnel: w309 -> [w312]
              tunnel: w307 -> [w311]
              tunnel: [w310] -> w308
              stop <- w314 stop-if-true
              n202 = Wait Until Next ms Multiple(millisecond multiple=u32 50 ("毫秒倍数")) -> ()  [unwired: 1 out]
              n203 = call "PCI1220U进给轴位置模式.vi"("Distance"=w311, "AxisHandle IN"=w312) -> ("AbsSuccess"=w314:bool, "AxisHandle OUT"=w310:u32)  [unwired: 8 in]
            }
          }
          frame #6 {
            n204 = while {
              stop <- w318 stop-if-true
              n205 = local read "测头机构轴检测位"() -> (w320:dbl)
              n206 = local read "测头机构轴位置(mm)"() -> (w317:dbl)
              n207 = Wait Until Next ms Multiple(millisecond multiple=u32 50 ("毫秒倍数")) -> ()  [unwired: 1 out]
              n208 = Subtract(x=w320, y=20.0) -> (x-y=w316:dbl)
              n209 = Greater Or Equal?(x=w317, y=w316) -> (x >= y?=w318:bool)
            }
          }
          frame #7 {
            n210 = local write "测头机构轴速度(mm/s)"(10.0 ("测头机构轴速度(mm/s)")) -> ()
          }
          frame #8 {
            n211 = while {
              tunnel: w324 -> [w328]
              stop <- w326 stop-if-true
              n212 = call <userlib>:"Acm_AxGetCmdVelocity.vi"("AxisHandle"=w328) -> ("Velocity"=w327:dbl)  [unwired: 1 in, 3 out]
              n213 = Wait Until Next ms Multiple(millisecond multiple=u32 50 ("毫秒倍数")) -> ()  [unwired: 1 out]
              n214 = Equal To 0?(x=w327) -> (x = 0?=w326:bool)
            }
          }
          frame #9 {
            n215 = local write "旋转齿条轴使能"(TRUE ("旋转齿条轴使能")) -> ()
          }
          frame #10 {
            n216 = local read "旋转齿条电机"() -> (w330:u32)
            n217 = call "PCI1220U角度置零.vi"("AxisHandle IN"=w330) -> ()  [unwired: 10 in, 1 out]
          }
          frame #11 {
            n218 = local write "旋转齿条轴速度(°/s)"(1.0 ("旋转齿条轴速度(°/s)")) -> ()
            n219 = Wait Until Next ms Multiple(millisecond multiple=u32 2000 ("毫秒倍数")) -> ()  [unwired: 1 out]
          }
          frame #12 {
            n220 = while {
              i -> [w337]
              stop <- w335 stop-if-true
              n221 = local read "间隙位移(mm)"() -> (→"基准位移":dbl)
              n222 = Wait Until Next ms Multiple(millisecond multiple=u32 500 ("毫秒倍数")) -> ()  [unwired: 1 out]
              n223 = Greater Or Equal?(x=w337, y=4) -> (x >= y?=w335:bool)
            }
          }
          frame #13 {
            n224 = call "PCI1220U运行.vi"("方向"=enum32{"Negative", "Positive"}."Negative" ("Direction"), "AxisHandle IN"=w341) -> ("AxisHandle OUT"=w340:u32)  [unwired: 9 in]
          }
          frame #14 {
            w346 = dbl[] []
            n225 = while {
              shift-right: [w357] -> w345
              shift-left: w346 -> [w359]
              shift-right: [w356] -> w344
              shift-left: w346 -> [w358]
              stop <- w349 stop-if-true
              n226 = Wait (ms)(milliseconds to wait=u32 10 ("毫秒倍数")) -> ()  [unwired: 1 out]
              n227 = local read "间隙位移(mm)"() -> (w352:dbl)
              n228 = local read "基准位移"() -> (w350:dbl)
              n229 = local read "齿条扭矩(Nm)"() -> (w353:dbl)
              n230 = Subtract(x=w352, y=w350) -> (x-y=w351:dbl)
              n231 = Absolute Value(x=w353) -> (abs(x)=w348:dbl)
              n232 = Build Array (concatenate) ("创建数组")(w358, w351) -> (w356:dbl[])
              n233 = Build Array (concatenate) ("创建数组")(w359, w348) -> (w357:dbl[])
              n234 = Greater Or Equal?(x=w348, y="扭矩停止值") -> (x >= y?=w349:bool)
              n235 = Bundle ("捆绑")(w357, w356) -> (w354:cluster{dbl[], dbl[]})  [unwired: 1 in]
              n236 = Build Array ("创建数组")(w354) -> (w355:cluster{dbl[], dbl[]}[])
              n237 = local write "扭动曲线"(w355) -> ()
            }
          }
          frame #15 {
            n238 = Absolute Value(x=w369) -> (abs(x)=w370:dbl[])
            n239 = local read "测量点扭矩"() -> (w371:dbl)
            n240 = local read "基准位移"() -> (w365:dbl)
            n241 = call "自定义插值.vi"("压力"=w371, "扭矩数组"=w370, "位移数组"=w368) -> ("扭矩值"=w366:dbl)  [unwired: 8 in]
            n242 = Array Max & Min(array=w368) -> (min value=w367:dbl)  [unwired: 3 out]
            n243 = Absolute Value(x=w367) -> (abs(x)=w364:dbl)
            n244 = Subtract(x=w365, y=w364) -> (x-y=w363:dbl)
            n245 = Add(x=w364, y=w366) -> (x+y=w361:dbl)
            n246 = Absolute Value(x=w361) -> (abs(x)=w362:dbl)
            n247 = local write "中间位置间隙"(w362) -> ()
            n248 = local write "基准位移"(w363) -> ()
          }
          frame #16 {
            n249 = while {
              tunnel: w376 -> [w380]
              tunnel: [w379] -> w375
              stop <- w378 stop-if-true
              n250 = call "PCI1220U停止.vi"("AxisHandle IN"=w380) -> ("完成"=w378:bool, "AxisHandle OUT"=w379:u32)  [unwired: 9 in]
              n251 = Wait (ms)(milliseconds to wait=u32 50 ("毫秒倍数")) -> ()  [unwired: 1 out]
            }
            "间隙Y数组" <- w374
            "间隙X数组" <- w373
          }
          frame #17 {
            n252 = while {
              tunnel: [w387] -> w381
              tunnel: w382 -> [w385]
              stop <- w386 stop-if-true
              n253 = Wait Until Next ms Multiple(millisecond multiple=u32 50 ("毫秒倍数")) -> ()  [unwired: 1 out]
              n254 = call "PCI1220U扭矩轴位置模式.vi"("Distance"=0.0, "AxisHandle IN"=w385) -> ("AbsSuccess"=w386:bool, "AxisHandle OUT"=w387:u32)  [unwired: 8 in]
            }
          }
          frame #18 {
            n255 = Wait (ms)(milliseconds to wait=u32 500 ("等待时间（毫秒）")) -> ()  [unwired: 1 out]
          }
          frame #19 {
            n256 = while {
              tunnel: w391 -> [w399]
              tunnel: [w395] -> w390
              stop <- w396 stop-if-true
              n257 = local read "齿条扭矩(Nm)"() -> (w394:dbl)
              n258 = call <userlib>:"Acm_AxGetCmdVelocity.vi"("AxisHandle"=w399) -> ("Velocity"=w400:dbl, "AxisHandle"=w395:u32)  [unwired: 1 in, 2 out]
              n259 = Greater Or Equal?(x=w394, y=3.0) -> (x >= y?=w392:bool)
              n260 = Equal To 0?(x=w400) -> (x = 0?=w397:bool)
              n261 = Or(x=w397, y=w392) -> (x .or. y?=w396:bool)
              n262 = Wait Until Next ms Multiple(millisecond multiple=u32 50 ("毫秒倍数")) -> ()  [unwired: 1 out]
            }
          }
          frame #20 {
            n263 = while {
              tunnel: w401 -> [w405]
              tunnel: [w404] -> _
              stop <- w403 stop-if-true
              n264 = call "PCI1220U停止.vi"("AxisHandle IN"=w405) -> ("完成"=w403:bool, "AxisHandle OUT"=w404:u32)  [unwired: 9 in]
              n265 = Wait (ms)(milliseconds to wait=u32 50 ("毫秒倍数")) -> ()  [unwired: 1 out]
            }
          }
          frame #21 {
            n266 = local write "旋转齿条轴使能"(FALSE ("旋转齿条轴使能")) -> ()
            n267 = Wait (ms)(milliseconds to wait=u32 500 ("毫秒倍数")) -> ()  [unwired: 1 out]
          }
          frame #22 {
            n268 = local write "工步号"(u32 25 ("工步号")) -> ()
          }
        }
      }
      frame 25 {
        n269 = flat-sequence {
          frame #0 {
            n270 = local read "中间位置最大间隙标准(mm)"() -> (w410:dbl)
            n271 = local read "中间位置间隙"() -> (w411:dbl)
            n272 = local read "最小间隙(mm)"() -> (w409:dbl)
            n273 = In Range and Coerce(upper limit=w410, x=w411, lower limit=w409) -> (In Range?=w414:bool)  [unwired: 1 out]
            n274 = case shown="假" w414 {
              tunnel: [FALSE ("本序合格") TRUE ("本序合格")] -> w413
              tunnel: [w419 0.0 ("需调整角度(度)")] -> w412
              tunnel: w411 -> [w417 _]
              tunnel: w410 -> [w416 _]
              tunnel: w409 -> [w415 _]
              frame False {
                n275 = xnode "公式"("X"=w417, "Xmax"=w416, "Xmin"=w415) -> ("结果"=w419:dbl)  [unwired: 1 in, 1 out]
              }
              frame True {
              }
            }
            n276 = local write "单点间隙合格"(w413) -> ()
            n277 = local write "需调整角度(度)"(w412) -> ()
          }
          frame #1 {
            n278 = local read "单点间隙合格"() -> (w434:bool)
            n279 = case shown="假" w434 {
              frame False {
                n280 = local read "单点间隙已调试次数"() -> (w437:dbl)
                n281 = Less?(x=w437, y="间隙设定调整次数") -> (x < y?=w436:bool)
                n282 = case shown="假" w436 {
                  frame False {
                    n283 = local write "工步号"(u32 45 ("变更工步号")) -> ()
                  }
                  frame True {
                    n284 = local write "工步号"(u32 30 ("变更工步号")) -> ()
                  }
                }
              }
              frame True {
                n285 = local write "工步号"(u32 40 ("变更工步号")) -> ()
              }
            }
          }
        }
      }
      frame 30 {
        # "人工调整"
        n286 = flat-sequence {
          tunnel: [w443] -> w441
          tunnel: w441 -> [w450]
          frame #0 {
            n287 = local write "测头机构轴速度(mm/s)"(30.0 ("测头机构轴速度(mm/s)")) -> ()
          }
          frame #1 {
            n288 = local read "测头机构电机"() -> (w444:u32)
            n289 = while {
              tunnel: w444 -> [w447]
              tunnel: [w446] -> w443
              stop <- w449 stop-if-true
              n290 = local read "测头机构轴待检位"() -> (w445:dbl)
              n291 = call "PCI1220U进给轴位置模式.vi"("Distance"=w445, "AxisHandle IN"=w447) -> ("AbsSuccess"=w449:bool, "AxisHandle OUT"=w446:u32)  [unwired: 8 in]
              n292 = Wait Until Next ms Multiple(millisecond multiple=u32 50 ("毫秒倍数")) -> ()  [unwired: 1 out]
            }
          }
          frame #2 {
            n293 = while {
              tunnel: w450 -> [w454]
              stop <- w452 stop-if-true
              n294 = call <userlib>:"Acm_AxGetCmdVelocity.vi"("AxisHandle"=w454) -> ("Velocity"=w453:dbl)  [unwired: 1 in, 3 out]
              n295 = Wait Until Next ms Multiple(millisecond multiple=u32 50 ("毫秒倍数")) -> ()  [unwired: 1 out]
              n296 = Equal To 0?(x=w453) -> (x = 0?=w452:bool)
            }
          }
          frame #3 {
            n297 = while {
              stop <- w456 stop-if-true
              n298 = local read "测头机构轴位置(mm)"() -> (w458:dbl)
              n299 = Wait Until Next ms Multiple(millisecond multiple=u32 50 ("毫秒倍数")) -> ()  [unwired: 1 out]
              n300 = Less Or Equal?(x=w458, y=35.0) -> (x <= y?=w456:bool)
            }
          }
          frame #4 {
            n301 = local write "测头气缸左移"(TRUE ("测头气缸左移")) -> ()
            n302 = local write "测头气缸右移"(FALSE ("测头气缸右移")) -> ()
          }
          frame #5 {
            n303 = while {
              stop <- w461 stop-if-true
              # "等待启动"
              n304 = local read "间隙启动"() -> (w461:bool)
              n305 = Wait Until Next ms Multiple(millisecond multiple=u32 50 ("毫秒倍数")) -> ()  [unwired: 1 out]
            }
          }
          frame #6 {
            n306 = local read "不合格品"() -> (w463:bool)
            n307 = case shown="假" w463 {
              frame False {
                n308 = flat-sequence {
                  frame #0 {
                    n309 = local read "单点间隙已调试次数"() -> (w466:dbl)
                    n310 = local write "测头气缸左移"(FALSE ("测头气缸左移")) -> ()
                    n311 = local write "测头气缸右移"(TRUE ("测头气缸左移")) -> ()
                    n312 = Add(x=w466, y=1.0 ("已调试次数")) -> (x+y=w468:dbl)
                    n313 = local write "单点间隙已调试次数"(w468) -> ()
                  }
                  frame #1 {
                    n314 = while {
                      stop <- w469 stop-if-true
                      n315 = Wait Until Next ms Multiple(millisecond multiple=u32 50 ("毫秒倍数")) -> ()  [unwired: 1 out]
                      n316 = local read "测头右位"() -> (w469:bool)
                    }
                  }
                  frame #2 {
                    n317 = local write "工步号"(u32 20 ("工步号")) -> ()
                  }
                }
              }
              frame True {
                n318 = local write "工步号"(u32 45 ("工步号")) -> ()
              }
            }
          }
        }
      }
      frame 40 {
        n319 = flat-sequence {
          tunnel: [w594] -> w590
          tunnel: w590 -> [w596]
          tunnel: [w595] -> w589
          tunnel: w589 -> [w604]
          tunnel: [w604] -> w588
          tunnel: w588 -> [w616]
          tunnel: [w616] -> w587
          tunnel: w587 -> [w618]
          tunnel: [w617] -> w586
          tunnel: w586 -> [w626]
          tunnel: [w626] -> w585
          tunnel: w585 -> [w636]
          tunnel: [w636] -> w584
          tunnel: w584 -> [w644]
          tunnel: [w644] -> w583
          tunnel: w583 -> [w646]
          tunnel: [w647] -> w582
          tunnel: [w645] -> w581
          tunnel: w582 -> [w660]
          tunnel: w581 -> [w655]
          tunnel: [w658] -> w580
          tunnel: [w657] -> w579
          tunnel: [w656] -> w578
          tunnel: [w655] -> w577
          tunnel: [w697] -> w576
          tunnel: [w700] -> w575
          tunnel: w580 -> [w700]
          tunnel: [w699] -> w574
          tunnel: w579 -> [w699]
          tunnel: [w698] -> w573
          tunnel: w578 -> [w698]
          tunnel: w577 -> [w697]
          tunnel: w576 -> [w706]
          tunnel: [w702] -> w572
          tunnel: [w705] -> w571
          tunnel: w575 -> [w705]
          tunnel: [w704] -> w570
          tunnel: w574 -> [w704]
          tunnel: [w703] -> w569
          tunnel: w573 -> [w703]
          tunnel: [w701] -> w568
          tunnel: [w721] -> w564
          tunnel: [w720] -> w565
          tunnel: [w719] -> w566
          tunnel: w572 -> [w714]
          tunnel: w571 -> [w718]
          tunnel: w570 -> [w717]
          tunnel: w569 -> [w716]
          tunnel: w568 -> [w715]
          tunnel: [w714] -> w567
          tunnel: [w774] -> w563
          tunnel: [w759] -> w562
          tunnel: [w773] -> w561
          tunnel: [w772] -> w560
          tunnel: [w771] -> w559
          tunnel: [w770] -> w558
          tunnel: [w769] -> w557
          tunnel: w567 -> [w773]
          tunnel: w566 -> [w772]
          tunnel: w565 -> [w759]
          tunnel: w564 -> [w774]
          tunnel: [w760] -> w556
          tunnel: w563 -> [w796]
          tunnel: [w796] -> w555
          tunnel: w562 -> [w795]
          tunnel: [w795] -> w554
          tunnel: w561 -> [w794]
          tunnel: [w783] -> w553
          tunnel: [w782] -> w552
          tunnel: [w793] -> w551
          tunnel: w560 -> [w793]
          tunnel: w559 -> [w790]
          tunnel: w558 -> [w792]
          tunnel: w557 -> [w791]
          tunnel: [w785] -> w550
          tunnel: [w784] -> w549
          tunnel: w556 -> [w781]
          tunnel: w555 -> [w809]
          tunnel: w554 -> [w808]
          tunnel: w553 -> [w804]
          tunnel: w552 -> [w811]
          tunnel: [w811] -> w547
          tunnel: w551 -> [w810]
          tunnel: [w806] -> w546
          tunnel: w550 -> [w813]
          tunnel: [w813] -> w545
          tunnel: w549 -> [w812]
          tunnel: [w812] -> w544
          tunnel: [w807] -> w548
          tunnel: [w805] -> w543
          tunnel: [w804] -> w542
          tunnel: w548 -> [w858]
          tunnel: [w858] -> w541
          tunnel: [w852] -> w540
          tunnel: w547 -> [w857]
          tunnel: [w857] -> w539
          tunnel: w546 -> [w856]
          tunnel: [w856] -> w538
          tunnel: w545 -> [w855]
          tunnel: [w855] -> w537
          tunnel: w544 -> [w854]
          tunnel: [w854] -> w536
          tunnel: [w853] -> w535
          tunnel: w543 -> [w853]
          tunnel: w542 -> [w852]
          tunnel: w541 -> [w865]
          tunnel: [w865] -> w534
          tunnel: w540 -> [w859]
          tunnel: w539 -> [w864]
          tunnel: [w864] -> w533
          tunnel: w538 -> [w863]
          tunnel: [w863] -> w532
          tunnel: w537 -> [w862]
          tunnel: [w862] -> w531
          tunnel: w536 -> [w861]
          tunnel: [w861] -> w530
          tunnel: [w859] -> w529
          tunnel: [w860] -> w528
          tunnel: w535 -> [w860]
          tunnel: [w881] -> w527
          tunnel: [w880] -> w526
          tunnel: w534 -> [w873]
          tunnel: [w872] -> w525
          tunnel: w533 -> [w875]
          tunnel: [w875] -> w524
          tunnel: w532 -> [w876]
          tunnel: [w879] -> w523
          tunnel: w531 -> [w877]
          tunnel: w530 -> [w878]
          tunnel: [w878] -> w522
          tunnel: [w877] -> w521
          tunnel: w529 -> [w872]
          tunnel: w528 -> [w874]
          tunnel: w527 -> [w924]
          tunnel: w526 -> [w930]
          tunnel: [w930] -> w520
          tunnel: w525 -> [w927]
          tunnel: [w927] -> w519
          tunnel: w524 -> [w929]
          tunnel: [w929] -> w518
          tunnel: w523 -> [w928]
          tunnel: [w928] -> w517
          tunnel: [w924] -> w516
          tunnel: [w923] -> w515
          tunnel: [w922] -> w514
          tunnel: w522 -> [w920]
          tunnel: w521 -> [w921]
          tunnel: [w921] -> w513
          tunnel: [w920] -> w512
          tunnel: [w919] -> w511
          tunnel: w520 -> [w943]
          tunnel: [w977] -> w510
          tunnel: w519 -> [w977]
          tunnel: [w976] -> w509
          tunnel: w518 -> [w976]
          tunnel: w517 -> [w975]
          tunnel: [w973] -> w508
          tunnel: w516 -> [w972]
          tunnel: w515 -> [w970]
          tunnel: w514 -> [w969]
          tunnel: [w967] -> w507
          tunnel: [w966] -> w506
          tunnel: [w965] -> w505
          tunnel: [w940] -> w504
          tunnel: [w939] -> w503
          tunnel: w513 -> [w962]
          tunnel: w512 -> [w961]
          tunnel: [w962] -> w502
          tunnel: [w961] -> w501
          tunnel: [w960] -> w500
          tunnel: [w959] -> w499
          tunnel: [w956] -> w498
          tunnel: [w951] -> w497
          tunnel: [w946] -> w496
          tunnel: [w938] -> w495
          tunnel: w511 -> [w937]
          tunnel: w510 -> [w1004]
          tunnel: [w1004] -> w494
          tunnel: w509 -> [_]
          tunnel: [w1001] -> w493
          tunnel: w508 -> [w1003]
          tunnel: [w1000] -> w492
          tunnel: w507 -> [w999]
          tunnel: w506 -> [w998]
          tunnel: w505 -> [w997]
          tunnel: [w996] -> w491
          tunnel: [w995] -> w490
          tunnel: w504 -> [w994]
          tunnel: w503 -> [w993]
          tunnel: w502 -> [w989]
          tunnel: w501 -> [w988]
          tunnel: [w989] -> w489
          tunnel: [w988] -> w488
          tunnel: [w987] -> w487
          tunnel: [w986] -> w486
          tunnel: w500 -> [w986]
          tunnel: [w985] -> w485
          tunnel: w499 -> [w985]
          tunnel: [w984] -> w484
          tunnel: [w983] -> w483
          tunnel: w498 -> [w982]
          tunnel: [w981] -> w482
          tunnel: w497 -> [w981]
          tunnel: [w980] -> w481
          tunnel: w496 -> [w980]
          tunnel: w495 -> [w979]
          tunnel: w494 -> [w1021]
          tunnel: [w1021] -> w480
          tunnel: w493 -> [w1020]
          tunnel: [w1020] -> w479
          tunnel: w492 -> [w1019]
          tunnel: [w1019] -> w478
          tunnel: w491 -> [w1014]
          tunnel: w490 -> [w1013]
          tunnel: w489 -> [w1016]
          tunnel: w488 -> [w1015]
          tunnel: w487 -> [w1012]
          tunnel: w486 -> [w1011]
          tunnel: w485 -> [w1010]
          tunnel: w484 -> [w1009]
          tunnel: w483 -> [w1008]
          tunnel: w482 -> [w1006]
          tunnel: w481 -> [w1005]
          tunnel: w480 -> [w1025]
          tunnel: [w1024] -> w477
          tunnel: w479 -> [w1023]
          tunnel: w478 -> [w1022]
          tunnel: [w1022] -> w476
          tunnel: w477 -> [w1032]
          tunnel: [w1032] -> w475
          tunnel: w476 -> [w1031]
          tunnel: [w1031] -> w474
          tunnel: w475 -> [w1039]
          tunnel: [w1038] -> w473
          tunnel: w474 -> [w1037]
          tunnel: w473 -> [w1045]
          frame #0 {
            n320 = local read "电动缸快速"() -> (w591:dbl)
            n321 = local write "电动缸速度(mm/s)"(w591) -> ()
            n322 = local write "单点间隙已调试次数"(0.0 ("单点间隙已调试次数")) -> ()
            n323 = local read "电动缸电机"() -> (w594:u32)
            n324 = local write "选项卡控件"(T1."轴向力测量" ("选项卡控件")) -> ()
          }
          frame #1 {
            n325 = while {
              tunnel: w596 -> [w603]
              tunnel: [w602] -> w595
              stop <- w597 stop-if-true
              n326 = local read "齿条左极限"() -> (w600:dbl)
              n327 = Wait (ms)(milliseconds to wait=u32 50 ("毫秒倍数")) -> ()  [unwired: 1 out]
              n328 = local read "循环退出"() -> (w599:bool)
              n329 = call "PCI1240电动缸位置模式 .vi"("Distance"=w600, "AxisHandle IN"=w603) -> ("AbsSuccess"=w598:bool, "AxisHandle OUT"=w602:u32)  [unwired: 8 in]
              n330 = Compound Arithmetic op=OR(w598, w599) -> (w597:bool)
            }
          }
          frame #2 {
            n331 = while {
              tunnel: w604 -> [w605]
              stop <- w607 stop-if-true
              n332 = local read "齿条推拉力(N)"() -> (w611:dbl)
              n333 = Wait (ms)(milliseconds to wait=u32 50 ("毫秒倍数")) -> ()  [unwired: 1 out]
              n334 = call <userlib>:"Acm_AxGetCmdVelocity.vi"("AxisHandle"=w605) -> ("Velocity"=w613:dbl)  [unwired: 1 in, 3 out]
              n335 = local read "循环退出"() -> (w606:bool)
              n336 = Less Or Equal?(x=w611, y=-500.0) -> (x <= y?=w608:bool)
              n337 = Equal To 0?(x=w613) -> (x = 0?=w609:bool)
              n338 = Compound Arithmetic op=OR(w609, w608, w606) -> (w607:bool)
            }
          }
          frame #3 {
            n339 = local read "电动缸慢速"() -> (w614:dbl)
            n340 = local write "电动缸速度(mm/s)"(w614) -> ()
            n341 = Wait (ms)(milliseconds to wait=u32 100 ("等待时间（毫秒）")) -> ()  [unwired: 1 out]
          }
          frame #4 {
            n342 = while {
              tunnel: w618 -> [w625]
              tunnel: [w623] -> w617
              stop <- w619 stop-if-true
              n343 = Wait (ms)(milliseconds to wait=u32 50 ("毫秒倍数")) -> ()  [unwired: 1 out]
              n344 = local read "循环退出"() -> (w621:bool)
              n345 = call "PCI1240电动缸位置模式 .vi"("Distance"=10000.0, "AxisHandle IN"=w625) -> ("AbsSuccess"=w620:bool, "AxisHandle OUT"=w623:u32)  [unwired: 8 in]
              n346 = Compound Arithmetic op=OR(w620, w621) -> (w619:bool)
            }
          }
          frame #5 {
            n347 = while {
              tunnel: w626 -> [w627]
              stop <- w629 stop-if-true
              n348 = local read "齿条推拉力(N)"() -> (w633:dbl)
              n349 = Wait (ms)(milliseconds to wait=u32 50 ("毫秒倍数")) -> ()  [unwired: 1 out]
              n350 = call <userlib>:"Acm_AxGetCmdVelocity.vi"("AxisHandle"=w627) -> ("Velocity"=w635:dbl)  [unwired: 1 in, 3 out]
              n351 = local read "循环退出"() -> (w628:bool)
              n352 = Less Or Equal?(x=w633, y=-500.0) -> (x <= y?=w630:bool)
              n353 = Equal To 0?(x=w635) -> (x = 0?=w631:bool)
              n354 = Compound Arithmetic op=OR(w631, w630, w628) -> (w629:bool)
            }
          }
          frame #6 {
            n355 = while {
              tunnel: w636 -> [w641]
              stop <- w637 stop-if-true
              n356 = call "PCI1220U停止.vi"("AxisHandle IN"=w641) -> ("完成"=w638:bool)  [unwired: 9 in, 1 out]
              n357 = local read "循环退出"() -> (w639:bool)
              n358 = Wait (ms)(milliseconds to wait=u32 50 ("毫秒倍数")) -> ()  [unwired: 1 out]
              n359 = Compound Arithmetic op=OR(w638, w639) -> (w637:bool)
            }
          }
          frame #7 {
            n360 = local read "电动缸快速"() -> (w642:dbl)
            n361 = local write "电动缸速度(mm/s)"(w642) -> ()
            n362 = Wait (ms)(milliseconds to wait=u32 100 ("毫秒倍数")) -> ()  [unwired: 1 out]
          }
          frame #8 {
            n363 = while {
              tunnel: w646 -> [w654]
              tunnel: [w652] -> w645
              stop <- w648 stop-if-true
              n364 = local read "齿条右极限"() -> (w651:dbl)
              n365 = Wait (ms)(milliseconds to wait=u32 50 ("毫秒倍数")) -> ()  [unwired: 1 out]
              n366 = local read "循环退出"() -> (w650:bool)
              n367 = call "PCI1240电动缸位置模式 .vi"("Distance"=w651, "AxisHandle IN"=w654) -> ("AbsSuccess"=w649:bool, "AxisHandle OUT"=w652:u32)  [unwired: 8 in]
              n368 = Compound Arithmetic op=OR(w649, w650) -> (w648:bool)
            }
            n369 = local read "转向器中心"() -> (w647:dbl)
          }
          frame #9 {
            w659 = dbl[] []
            n370 = while {
              shift-right: [w678] -> w657
              shift-left: w659 -> [w688]
              shift-right: [w686] -> w658
              shift-left: w659 -> [w687]
              tunnel: w655 -> [w682]
              tunnel: w660 -> [w681]
              shift-right: [w677] -> w656
              shift-left: w659 -> [w679]
              stop <- w671 stop-if-true
              n371 = local read "基准位移"() -> (w683:dbl)
              n372 = local read "间隙位移(mm)"() -> (w668:dbl)
              n373 = local read "电动缸位置(mm)"() -> (w664:dbl)
              n374 = call <userlib>:"Acm_AxGetCmdVelocity.vi"("AxisHandle"=w682) -> ("Velocity"=w676:dbl)  [unwired: 1 in, 3 out]
              n375 = Wait (ms)(milliseconds to wait=u32 50 ("毫秒倍数")) -> ()  [unwired: 1 out]
              n376 = disable-structure shown="禁用" {
                disable-tunnel: w668 -> [w695 _]
                frame Disabled {
                  n377 = Less Or Equal?(x=w695, y=-1.0) -> (x <= y?=w694:bool)
                  n378 = Greater Or Equal?(x=w695, y=4.0) -> (x >= y?=w693:bool)
                  n379 = Or(x=w693, y=w694) -> (x .or. y?=w692:bool)
                  n380 = property on="间隙位移(mm)" class="DigNum (严格)"("Blinking"=w692) -> ()  [unwired: 2 in, 2 out]
                }
                frame Enabled {
                }
              }
              n381 = local read "齿条推拉力(N)"() -> (w674:dbl)
              n382 = Subtract(x=w668, y=w683) -> (x-y=w670:dbl)
              n383 = Subtract(x=w664, y=w681) -> (x-y=w667:dbl)
              n384 = Add(x=w670, y=0.0) -> (x+y=w669:dbl)
              n385 = local read "循环退出"() -> (w663:bool)
              n386 = Negate(x=w669) -> (-x=w661:dbl)
              n387 = Multiply(x=w667, y=1.0) -> (x*y=w665:dbl)
              n388 = Build Array (concatenate) ("创建数组")(w687, w661) -> (w686:dbl[])
              n389 = Build Array (concatenate) ("创建数组")(w688, w665) -> (w678:dbl[])
              n390 = Build Array (concatenate) ("创建数组")(w679, w674) -> (w677:dbl[])
              n391 = Greater Or Equal?(x=w674, y=500.0) -> (x >= y?=w672:bool)
              n392 = Equal To 0?(x=w676) -> (x = 0?=w673:bool)
              n393 = Bundle ("捆绑")(w678, w686) -> (w684:cluster{dbl[], dbl[]})  [unwired: 1 in]
              n394 = Compound Arithmetic op=OR(w673, w672, w663) -> (w671:bool)
              n395 = Bundle ("捆绑")(w678, w677) -> (w680:cluster{dbl[], dbl[]})  [unwired: 1 in]
              n396 = Build Array ("创建数组")(w684, w680) -> (w685:cluster{dbl[], dbl[]}[])
              n397 = local write "行程跳动曲线"(w685) -> ()
            }
          }
          frame #10 {
            n398 = local read "电动缸慢速"() -> (w696:dbl)
            n399 = local write "电动缸速度(mm/s)"(w696) -> ()
          }
          frame #11 {
            n400 = while {
              tunnel: w706 -> [w713]
              tunnel: [w711] -> w702
              stop <- w707 stop-if-true
              n401 = Wait (ms)(milliseconds to wait=u32 50 ("毫秒倍数")) -> ()  [unwired: 1 out]
              n402 = local read "循环退出"() -> (w709:bool)
              n403 = call "PCI1240电动缸位置模式 .vi"("Distance"=-10.0, "AxisHandle IN"=w713) -> ("AbsSuccess"=w708:bool, "AxisHandle OUT"=w711:u32)  [unwired: 8 in]
              n404 = Compound Arithmetic op=OR(w708, w709) -> (w707:bool)
            }
            n405 = local read "转向器中心"() -> (w701:dbl)
          }
          frame #12 {
            n406 = while {
              shift-right: [w739] -> w720
              shift-left: w717 -> [w749]
              shift-right: [w747] -> w721
              shift-left: w718 -> [w748]
              tunnel: w714 -> [w743]
              tunnel: w715 -> [w742]
              shift-right: [w738] -> w719
              shift-left: w716 -> [w740]
              stop <- w732 stop-if-true
              n407 = local read "基准位移"() -> (w744:dbl)
              n408 = local read "间隙位移(mm)"() -> (w729:dbl)
              n409 = local read "电动缸位置(mm)"() -> (w725:dbl)
              n410 = call <userlib>:"Acm_AxGetCmdVelocity.vi"("AxisHandle"=w743) -> ("Velocity"=w737:dbl)  [unwired: 1 in, 3 out]
              n411 = Wait (ms)(milliseconds to wait=u32 50 ("毫秒倍数")) -> ()  [unwired: 1 out]
              n412 = disable-structure shown="禁用" {
                disable-tunnel: w729 -> [w756 _]
                frame Disabled {
                  n413 = Less Or Equal?(x=w756, y=-1.0) -> (x <= y?=w755:bool)
                  n414 = Greater Or Equal?(x=w756, y=4.0) -> (x >= y?=w754:bool)
                  n415 = Or(x=w754, y=w755) -> (x .or. y?=w753:bool)
                  n416 = property on="间隙位移(mm)" class="DigNum (严格)"("Blinking"=w753) -> ()  [unwired: 2 in, 2 out]
                }
                frame Enabled {
                }
              }
              n417 = local read "齿条推拉力(N)"() -> (w735:dbl)
              n418 = Subtract(x=w729, y=w744) -> (x-y=w731:dbl)
              n419 = Subtract(x=w725, y=w742) -> (x-y=w728:dbl)
              n420 = Add(x=w731, y=0.0) -> (x+y=w730:dbl)
              n421 = Negate(x=w730) -> (-x=w722:dbl)
              n422 = Multiply(x=w728, y=1.0) -> (x*y=w726:dbl)
              n423 = local read "循环退出"() -> (w724:bool)
              n424 = Build Array (concatenate) ("创建数组")(w748, w722) -> (w747:dbl[])
              n425 = Build Array (concatenate) ("创建数组")(w749, w726) -> (w739:dbl[])
              n426 = Build Array (concatenate) ("创建数组")(w740, w735) -> (w738:dbl[])
              n427 = Greater Or Equal?(x=w735, y=500.0) -> (x >= y?=w733:bool)
              n428 = Equal To 0?(x=w737) -> (x = 0?=w734:bool)
              n429 = Bundle ("捆绑")(w739, w747) -> (w745:cluster{dbl[], dbl[]})  [unwired: 1 in]
              n430 = Bundle ("捆绑")(w739, w738) -> (w741:cluster{dbl[], dbl[]})  [unwired: 1 in]
              n431 = Compound Arithmetic op=OR(w734, w733, w724) -> (w732:bool)
              n432 = Build Array ("创建数组")(w745, w741) -> (w746:cluster{dbl[], dbl[]}[])
              n433 = local write "行程跳动曲线"(w746) -> ()
            }
          }
          frame #13 {
            n434 = while {
              tunnel: w773 -> [w780]
              tunnel: [w779] -> _
              stop <- w775 stop-if-true
              n435 = call "PCI1220U停止.vi"("AxisHandle IN"=w780) -> ("完成"=w776:bool, "AxisHandle OUT"=w779:u32)  [unwired: 9 in]
              n436 = Wait (ms)(milliseconds to wait=u32 50 ("毫秒倍数")) -> ()  [unwired: 1 out]
              n437 = local read "循环退出"() -> (w777:bool)
              n438 = Compound Arithmetic op=OR(w776, w777) -> (w775:bool)
            }
            n439 = call "功能计算_何 截取位移左.vi"("位移数组"=w759, "拉压力数组"=w772, "半行程"="半行程", "截取百分比"="截取百分比") -> ("峰值扭矩"=w771:dbl, "平均扭矩"=w770:dbl, "扭差"=w769:dbl)  [unwired: 12 in, 1 out]
            "左轴向力波动(N)" <- w769
            "左最大轴向力(N)" <- w771
            n440 = call "间隙计算.vi"("扭矩数组"=w774) -> ("峰值间隙1"=w768:dbl, "峰值间隙2"=w767:dbl)  [unwired: 6 in, 3 out]
            n441 = local read "180°内全行程间隙标准(mm)"() -> (w766:dbl)
            n442 = Array Size(array=w759) -> (size(s)=w758:i32)
            n443 = local read "180°外全行程间隙标准(mm)"() -> (w763:dbl)
            n444 = local write "左平均轴向力(N)"(w770) -> ()
            n445 = local write "左180°外全行程间隙"(w767) -> ()
            n446 = local write "左180°内全行程间隙"(w768) -> ()
            n447 = local write "左轴向力数组大小"(w758) -> ()
            n448 = local read "电动缸快速"() -> (w757:dbl)
            n449 = Greater?(x=w768, y=w766) -> (0:w765:bool)
            n450 = Greater?(x=w767, y=w763) -> (0:w764:bool)
            n451 = local write "电动缸速度(mm/s)"(w757) -> ()
            n452 = property on="左180°内全行程间隙" class="DigNum (严格)"("Blinking"=w765) -> ()  [unwired: 2 in, 2 out]
            n453 = property on="左180°外全行程间隙" class="DigNum (严格)"("Blinking"=w764) -> ()  [unwired: 2 in, 2 out]
            n454 = local read "最大轴向力标准(N)"() -> (w760:dbl)
          }
          frame #14 {
            n455 = while {
              tunnel: w794 -> [w803]
              tunnel: [w800] -> w783
              stop <- w797 stop-if-true
              n456 = Wait (ms)(milliseconds to wait=u32 50 ("毫秒倍数")) -> ()  [unwired: 1 out]
              n457 = local read "齿条左极限"() -> (w801:dbl)
              n458 = local read "循环退出"() -> (w799:bool)
              n459 = call "PCI1240电动缸位置模式 .vi"("Distance"=w801, "AxisHandle IN"=w803) -> ("AbsSuccess"=w798:bool, "AxisHandle OUT"=w800:u32)  [unwired: 8 in]
              n460 = Compound Arithmetic op=OR(w798, w799) -> (w797:bool)
            }
            n461 = local read "轴向力标准(N)"() -> (w788:dbl)
            n462 = local read "平均轴向力标准(N) max"() -> (w787:dbl)
            n463 = local read "力波动标准(N)"() -> (w786:dbl)
            n464 = call "判断.vi"("y 3"=w786, "y 2-2"=w787, "y 2-1"=w788, "y"=w781, "x 3"=w791, "x 2"=w792, "x"=w790) -> ("非x? 3"=w784:bool, "非x? 2"=w789:bool, "非x?"=w785:bool)  [unwired: 2 in]
            n465 = property on="左最大轴向力(N)" class="DigNum (严格)"("Blinking"=w785) -> ()  [unwired: 2 in, 2 out]
            n466 = property on="左平均轴向力(N)" class="DigNum (严格)"("Blinking"=w789) -> ()  [unwired: 2 in, 2 out]
            n467 = property on="左轴向力波动(N)" class="DigNum (严格)"("Blinking"=w784) -> ()  [unwired: 2 in, 2 out]
            n468 = local read "转向器中心"() -> (w782:dbl)
          }
          frame #15 {
            n469 = while {
              shift-right: [w839] -> w805
              shift-left: w808 -> [w848]
              shift-right: [w846] -> w807
              shift-left: w809 -> [w847]
              tunnel: w804 -> [w841]
              tunnel: w811 -> [w840]
              shift-right: [w836] -> w806
              shift-left: w810 -> [w837]
              stop <- w831 stop-if-true
              n470 = local read "电动缸位置(mm)"() -> (w817:dbl)
              n471 = call <userlib>:"Acm_AxGetCmdVelocity.vi"("AxisHandle"=w841) -> ("Velocity"=w829:dbl)  [unwired: 1 in, 3 out]
              n472 = local read "间隙位移(mm)"() -> (w824:dbl)
              n473 = local read "基准位移"() -> (w842:dbl)
              n474 = Wait (ms)(milliseconds to wait=u32 50 ("毫秒倍数")) -> ()  [unwired: 1 out]
              n475 = local read "齿条推拉力(N)"() -> (w835:dbl)
              n476 = Add(x=1.47, y=w817) -> (x+y=w819:dbl)
              n477 = Subtract(x=w824, y=w842) -> (x-y=w843:dbl)
              n478 = Subtract(x=w819, y=w840) -> (x-y=w822:dbl)
              n479 = local read "循环退出"() -> (w816:bool)
              n480 = Add(x=w843, y=0.0) -> (x+y=w830:dbl)
              n481 = Multiply(x=w822, y=1.0) -> (x*y=w820:dbl)
              n482 = Negate(x=w830) -> (-x=w814:dbl)
              n483 = Build Array (concatenate) ("创建数组")(w848, w820) -> (w839:dbl[])
              n484 = Less Or Equal?(x=w835, y=-500.0) -> (x <= y?=w832:bool)
              n485 = Build Array (concatenate) ("创建数组")(w837, w835) -> (w836:dbl[])
              n486 = Equal To 0?(x=w829) -> (x = 0?=w833:bool)
              n487 = Build Array (concatenate) ("创建数组")(w847, w814) -> (w846:dbl[])
              n488 = Bundle ("捆绑")(w839, w836) -> (w838:cluster{dbl[], dbl[]})  [unwired: 1 in]
              n489 = Compound Arithmetic op=OR(w833, w832, w816) -> (w831:bool)
              n490 = Bundle ("捆绑")(w839, w846) -> (w844:cluster{dbl[], dbl[]})  [unwired: 1 in]
              n491 = Build Array ("创建数组")(w844, w838) -> (w845:cluster{dbl[], dbl[]}[])
              n492 = Less Or Equal?(x=w824, y=-1.0) -> (x <= y?=w828:bool)
              n493 = Greater Or Equal?(x=w824, y=4.0) -> (x >= y?=w827:bool)
              n494 = local write "行程跳动曲线"(w845) -> ()
              n495 = Or(x=w827, y=w828) -> (x .or. y?=w823:bool)
              n496 = disable-structure shown="禁用" {
                disable-tunnel: w823 -> [w850 _]
                frame Disabled {
                  n497 = property on="间隙位移(mm)" class="DigNum (严格)"("Blinking"=w850) -> ()  [unwired: 2 in, 2 out]
                }
                frame Enabled {
                }
              }
            }
          }
          frame #16 {
            n498 = local read "电动缸慢速"() -> (w851:dbl)
            n499 = local write "电动缸速度(mm/s)"(w851) -> ()
          }
          frame #17 {
            n500 = while {
              tunnel: w859 -> [w871]
              stop <- w866 stop-if-true
              n501 = Wait (ms)(milliseconds to wait=u32 50 ("毫秒倍数")) -> ()  [unwired: 1 out]
              n502 = local read "循环退出"() -> (w868:bool)
              n503 = call "PCI1240电动缸位置模式 .vi"("Distance"=160.0, "AxisHandle IN"=w871) -> ("AbsSuccess"=w867:bool)  [unwired: 8 in, 1 out]
              n504 = Compound Arithmetic op=OR(w867, w868) -> (w866:bool)
            }
          }
          frame #18 {
            n505 = while {
              shift-right: [w907] -> w880
              shift-left: w874 -> [w916]
              shift-right: [w914] -> w881
              shift-left: w873 -> [w915]
              tunnel: w872 -> [w909]
              tunnel: w875 -> [w908]
              shift-right: [w904] -> w879
              shift-left: w876 -> [w905]
              stop <- w899 stop-if-true
              n506 = local read "电动缸位置(mm)"() -> (w885:dbl)
              n507 = call <userlib>:"Acm_AxGetCmdVelocity.vi"("AxisHandle"=w909) -> ("Velocity"=w897:dbl)  [unwired: 1 in, 3 out]
              n508 = local read "间隙位移(mm)"() -> (w892:dbl)
              n509 = local read "基准位移"() -> (w910:dbl)
              n510 = Wait (ms)(milliseconds to wait=u32 50 ("毫秒倍数")) -> ()  [unwired: 1 out]
              n511 = local read "齿条推拉力(N)"() -> (w903:dbl)
              n512 = Subtract(x=w892, y=w910) -> (x-y=w911:dbl)
              n513 = Add(x=1.45, y=w885) -> (x+y=w887:dbl)
              n514 = Subtract(x=w887, y=w908) -> (x-y=w890:dbl)
              n515 = Add(x=w911, y=0.0) -> (x+y=w898:dbl)
              n516 = local read "循环退出"() -> (w884:bool)
              n517 = Negate(x=w898) -> (-x=w882:dbl)
              n518 = Multiply(x=w890, y=1.0) -> (x*y=w888:dbl)
              n519 = Build Array (concatenate) ("创建数组")(w916, w888) -> (w907:dbl[])
              n520 = Less Or Equal?(x=w903, y=-500.0) -> (x <= y?=w900:bool)
              n521 = Build Array (concatenate) ("创建数组")(w905, w903) -> (w904:dbl[])
              n522 = Equal To 0?(x=w897) -> (x = 0?=w901:bool)
              n523 = Build Array (concatenate) ("创建数组")(w915, w882) -> (w914:dbl[])
              n524 = Bundle ("捆绑")(w907, w904) -> (w906:cluster{dbl[], dbl[]})  [unwired: 1 in]
              n525 = Compound Arithmetic op=OR(w901, w900, w884) -> (w899:bool)
              n526 = Bundle ("捆绑")(w907, w914) -> (w912:cluster{dbl[], dbl[]})  [unwired: 1 in]
              n527 = Build Array ("创建数组")(w912, w906) -> (w913:cluster{dbl[], dbl[]}[])
              n528 = Less Or Equal?(x=w892, y=-1.0) -> (x <= y?=w896:bool)
              n529 = Greater Or Equal?(x=w892, y=4.0) -> (x >= y?=w895:bool)
              n530 = local write "行程跳动曲线"(w913) -> ()
              n531 = Or(x=w895, y=w896) -> (x .or. y?=w891:bool)
              n532 = disable-structure shown="禁用" {
                disable-tunnel: w891 -> [w918 _]
                frame Disabled {
                  n533 = property on="间隙位移(mm)" class="DigNum (严格)"("Blinking"=w918) -> ()  [unwired: 2 in, 2 out]
                }
                frame Enabled {
                }
              }
            }
          }
          frame #19 {
            n534 = while {
              tunnel: w927 -> [w936]
              tunnel: [w935] -> _
              stop <- w931 stop-if-true
              n535 = local read "循环退出"() -> (w933:bool)
              n536 = call "PCI1220U停止.vi"("AxisHandle IN"=w936) -> ("完成"=w932:bool, "AxisHandle OUT"=w935:u32)  [unwired: 9 in]
              n537 = Wait (ms)(milliseconds to wait=u32 50 ("毫秒倍数")) -> ()  [unwired: 1 out]
              n538 = Compound Arithmetic op=OR(w932, w933) -> (w931:bool)
            }
            n539 = Array Max & Min(array=w924) -> (max value=w926:dbl, min value=w925:dbl)  [unwired: 2 out]
            n540 = local read "左轴向力数组大小"() -> (w919:i32)
            n541 = Absolute Value(x=w926) -> (abs(x)=w923:dbl)
            n542 = Absolute Value(x=w925) -> (abs(x)=w922:dbl)
            n543 = local write "左全行程间隙"(w923) -> ()
            n544 = local write "右全行程间隙"(w922) -> ()
          }
          frame #20 {
            n545 = local read "180°内全行程间隙标准(mm)"() -> (w968:dbl)
            n546 = local read "截取百分比"() -> (w941:dbl)
            n547 = local read "齿条传动比"() -> (w945:dbl)
            n548 = local read "半行程"() -> (w942:dbl)
            n549 = Split 1D Array(array=w975, index=w937) -> (second subarray=w974:dbl[])  [unwired: 1 out]
            n550 = Split 1D Array(array=w943, index=w937) -> (second subarray=w944:dbl[])  [unwired: 1 out]
            n551 = Array Max & Min(array=w943) -> (max value=w964:dbl, min value=w963:dbl)  [unwired: 2 out]
            n552 = local read "机械间隙值"() -> (w957:dbl)
            n553 = local read "总圈数标准"() -> (w949:dbl)
            n554 = local read "总圈数最大值"() -> (w950:dbl)
            n555 = Subtract(x=w964, y=w963) -> (x-y=w958:dbl)
            n556 = call "功能计算_何 截取位移右.vi"("位移数组"=w944, "拉压力数组"=w974, "半行程"=w942, "截取百分比"=w941) -> ("峰值扭矩"=w940:dbl, "平均扭矩"=w973:dbl, "扭差"=w939:dbl)  [unwired: 12 in, 1 out]
            "右最大轴向力(N)" <- w940
            "右轴向力波动(N)" <- w939
            n557 = Subtract(x=w958, y=w957) -> (x-y=w955:dbl)
            n558 = Split 1D Array(array=w972, index=w937) -> (second subarray=w971:dbl[])  [unwired: 1 out]
            n559 = Greater?(x=w970, y=w968) -> (0:w960:bool)
            n560 = Greater?(x=w969, y=w968) -> (0:w959:bool)
            n561 = call "间隙计算.vi"("扭矩数组"=w971) -> ("峰值间隙1"=w966:dbl, "峰值间隙2"=w965:dbl)  [unwired: 6 in, 3 out]
            n562 = Divide(x=w955, y=w945) -> (x/y=w948:dbl)
            n563 = In Range and Coerce(upper limit=w950, x=w948, lower limit=w949) -> (In Range?=w947:bool)  [unwired: 1 out]
            n564 = Not(x=w947) -> (.not. x?=w946:bool)
            n565 = property on="总圈数" class="DigNum (严格)"("Blinking"=w946) -> ()  [unwired: 2 in, 2 out]
            n566 = property on="左全行程间隙" class="DigNum (严格)"("Blinking"=w960) -> ()  [unwired: 2 in, 2 out]
            n567 = property on="右全行程间隙" class="DigNum (严格)"("Blinking"=w959) -> ()  [unwired: 2 in, 2 out]
            n568 = local write "右平均轴向力(N)"(w973) -> ()
            n569 = local write "总圈数"(w948) -> ()
            n570 = local read "180°内全行程间隙标准(mm)"() -> (w967:dbl)
            n571 = local read "总行程标准(mm)"() -> (w953:dbl)
            n572 = local read "总行程最大值"() -> (w954:dbl)
            n573 = In Range and Coerce(upper limit=w954, x=w955, lower limit=w953) -> (In Range?=w952:bool)  [unwired: 1 out]
            n574 = local write "右180°外全行程间隙"(w965) -> ()
            n575 = local write "右180°内全行程间隙"(w966) -> ()
            n576 = local read "180°外全行程间隙标准(mm)"() -> (w956:dbl)
            n577 = local read "最大轴向力标准(N)"() -> (w938:dbl)
            n578 = Not(x=w952) -> (.not. x?=w951:bool)
            n579 = local write "总行程"(w955) -> ()
            n580 = property on="总行程" class="DigNum (严格)"("Blinking"=w951) -> ()  [unwired: 2 in, 2 out]
            "轴向力X" <- w943
            "轴向力Y" <- w975
          }
          frame #21 {
            n581 = local read "电动缸快速"() -> (w978:dbl)
            n582 = local read "轴向力标准(N)"() -> (w992:dbl)
            n583 = local read "平均轴向力标准(N) max"() -> (w991:dbl)
            n584 = Greater?(x=w998, y=w999) -> (0:w984:bool)
            n585 = Greater?(x=w997, y=w982) -> (0:w983:bool)
            n586 = local write "电动缸速度(mm/s)"(w978) -> ()
            n587 = local read "转向器中心"() -> (w1000:dbl)
            n588 = local read "力波动标准(N)"() -> (w990:dbl)
            n589 = call "判断.vi"("y 3"=w990, "y 2-2"=w991, "y 2-1"=w992, "y"=w979, "x 3"=w993, "x 2"=w1003, "x"=w994) -> ("非x? 3"=w987:bool, "非x? 2"=w995:bool, "非x?"=w996:bool)  [unwired: 2 in]
            n590 = property on="右180°内全行程间隙" class="DigNum (严格)"("Blinking"=w984) -> ()  [unwired: 2 in, 2 out]
            n591 = property on="右180°外全行程间隙" class="DigNum (严格)"("Blinking"=w983) -> ()  [unwired: 2 in, 2 out]
            n592 = Add(x=w1000, y=-10.0) -> (x+y=w1001:dbl)
          }
          frame #22 {
            n593 = Compound Arithmetic op=OR(w1011, w1010, w1009, w1008) -> (w1007:bool)
            n594 = property on="右最大轴向力(N)" class="DigNum (严格)"("Blinking"=w1014) -> ()  [unwired: 2 in, 2 out]
            n595 = property on="右平均轴向力(N)" class="DigNum (严格)"("Blinking"=w1013) -> ()  [unwired: 2 in, 2 out]
            n596 = property on="右轴向力波动(N)" class="DigNum (严格)"("Blinking"=w1012) -> ()  [unwired: 2 in, 2 out]
            n597 = Compound Arithmetic op=OR(w1005, w1007, w1014, w1012, w1016, w1015, w1006) -> (w1018:bool)
            n598 = Not(x=w1018) -> (.not. x?=w1017:bool)
            n599 = local write "轴向力及全行程间隙合格"(w1017) -> ()
          }
          frame #23 {
            n600 = while {
              tunnel: w1025 -> [w1029]
              tunnel: [w1027] -> w1024
              tunnel: w1023 -> [w1026]
              stop <- w1028 stop-if-true
              n601 = call "PCI1240电动缸位置模式 .vi"("Distance"=w1026, "AxisHandle IN"=w1029) -> ("AbsSuccess"=w1028:bool, "AxisHandle OUT"=w1027:u32)  [unwired: 8 in]
              n602 = Wait (ms)(milliseconds to wait=u32 50 ("毫秒倍数")) -> ()  [unwired: 1 out]
            }
          }
          frame #24 {
            n603 = while {
              tunnel: w1032 -> [w1036]
              stop <- w1034 stop-if-true
              n604 = call <userlib>:"Acm_AxGetCmdVelocity.vi"("AxisHandle"=w1036) -> ("Velocity"=w1035:dbl)  [unwired: 1 in, 3 out]
              n605 = Wait Until Next ms Multiple(millisecond multiple=u32 50 ("毫秒倍数")) -> ()  [unwired: 1 out]
              n606 = Equal To 0?(x=w1035) -> (x = 0?=w1034:bool)
            }
          }
          frame #25 {
            n607 = while {
              tunnel: w1039 -> [w1043]
              tunnel: [w1041] -> w1038
              tunnel: w1037 -> [w1040]
              stop <- w1042 stop-if-true
              n608 = call "PCI1240电动缸位置模式 .vi"("Distance"=w1040, "AxisHandle IN"=w1043) -> ("AbsSuccess"=w1042:bool, "AxisHandle OUT"=w1041:u32)  [unwired: 8 in]
              n609 = Wait (ms)(milliseconds to wait=u32 50 ("毫秒倍数")) -> ()  [unwired: 1 out]
            }
          }
          frame #26 {
            n610 = while {
              tunnel: w1045 -> [w1049]
              stop <- w1047 stop-if-true
              n611 = call <userlib>:"Acm_AxGetCmdVelocity.vi"("AxisHandle"=w1049) -> ("Velocity"=w1048:dbl)  [unwired: 1 in, 3 out]
              n612 = Wait Until Next ms Multiple(millisecond multiple=u32 50 ("毫秒倍数")) -> ()  [unwired: 1 out]
              n613 = Equal To 0?(x=w1048) -> (x = 0?=w1047:bool)
            }
          }
          frame #27 {
            n614 = local read "轴向力已做次数"() -> (w1052:dbl)
            n615 = Add(x=w1052, y=1.0) -> (x+y=w1050:dbl)
            n616 = local write "轴向力已做次数"(w1050) -> ()
          }
          frame #28 {
            n617 = local read "轴向力及全行程间隙合格"() -> (w1053:bool)
            n618 = case shown="假" w1053 {
              frame False {
                n619 = Less?(x="轴向力已做次数", y="轴向力设定次数") -> (x < y?=w1055:bool)
                n620 = case shown="假" w1055 {
                  frame False {
                    n621 = local write "工步号"(u32 45 ("工步号")) -> ()
                  }
                  frame True {
                    n622 = local write "工步号"(u32 30 ("工步号")) -> ()
                  }
                }
              }
              frame True {
                n623 = local write "工步号"(u32 45 ("工步号")) -> ()
              }
            }
          }
        }
      }
      frame 45 {
        # "测头退回"
        n624 = flat-sequence {
          tunnel: [w1063] -> w1060
          tunnel: w1060 -> [w1070]
          frame #0 {
            n625 = local write "测头机构轴速度(mm/s)"(30.0 ("测头机构轴速度(mm/s)")) -> ()
          }
          frame #1 {
            n626 = local read "测头机构轴后退位"() -> (w1062:dbl)
            n627 = local read "测头机构电机"() -> (w1064:u32)
            n628 = while {
              tunnel: w1064 -> [w1068]
              tunnel: w1062 -> [w1067]
              tunnel: [w1066] -> w1063
              stop <- w1069 stop-if-true
              n629 = Wait Until Next ms Multiple(millisecond multiple=u32 50 ("毫秒倍数")) -> ()  [unwired: 1 out]
              n630 = call "PCI1220U进给轴位置模式.vi"("Distance"=w1067, "AxisHandle IN"=w1068) -> ("AbsSuccess"=w1069:bool, "AxisHandle OUT"=w1066:u32)  [unwired: 8 in]
            }
          }
          frame #2 {
            n631 = while {
              tunnel: w1070 -> [w1074]
              stop <- w1072 stop-if-true
              n632 = call <userlib>:"Acm_AxGetCmdVelocity.vi"("AxisHandle"=w1074) -> ("Velocity"=w1073:dbl)  [unwired: 1 in, 3 out]
              n633 = Wait Until Next ms Multiple(millisecond multiple=u32 50 ("毫秒倍数")) -> ()  [unwired: 1 out]
              n634 = Equal To 0?(x=w1073) -> (x = 0?=w1072:bool)
            }
          }
          frame #3 {
            n635 = while {
              stop <- w1076 stop-if-true
              n636 = local read "测头机构轴位置(mm)"() -> (w1078:dbl)
              n637 = Wait Until Next ms Multiple(millisecond multiple=u32 50 ("毫秒倍数")) -> ()  [unwired: 1 out]
              n638 = Less Or Equal?(x=w1078, y=35.0) -> (x <= y?=w1076:bool)
            }
          }
          frame #4 {
            n639 = local write "测头气缸右移"(FALSE ("测头气缸右移")) -> ()
            n640 = local write "测头气缸左移"(TRUE ("测头气缸左移")) -> ()
          }
          frame #5 {
            n641 = Wait Until Next ms Multiple(millisecond multiple=u32 500 ("毫秒倍数")) -> ()  [unwired: 1 out]
          }
          frame #6 {
            n642 = local write "工步号"(u32 50 ("工步号")) -> ()
          }
        }
      }
      frame 50 {
        n643 = flat-sequence {
          tunnel: [w1105] -> w1094
          tunnel: w1094 -> [w1112]
          tunnel: [w1111] -> w1091
          tunnel: w1091 -> [w1123]
          tunnel: [w1129] -> w1088
          tunnel: w1088 -> [w1132]
          tunnel: [w1131] -> w1087
          tunnel: w1087 -> [w1136]
          tunnel: [w1136] -> w1086
          tunnel: w1086 -> [w1138]
          tunnel: [w1137] -> w1084
          tunnel: [w1144] -> w1085
          tunnel: w1084 -> [w1145]
          tunnel: w1085 -> [w1147]
          tunnel: [w1146] -> w1083
          tunnel: [w1153] -> w1093
          tunnel: w1083 -> [w1153]
          tunnel: w1093 -> [w1156]
          tunnel: [w1155] -> w1092
          tunnel: w1092 -> [w1162]
          tunnel: [w1163] -> w1090
          tunnel: w1090 -> [w1170]
          tunnel: [w1169] -> w1089
          tunnel: w1089 -> [w1180]
          frame #0 {
            n644 = local write "旋转齿条轴速度(°/s)"(15.0 ("调整螺塞轴速度(°/s)")) -> ()
            n645 = local write "测头机构轴速度(mm/s)"(15.0 ("调整机构轴速度(mm/s)")) -> ()
            n646 = local write "电动缸速度(mm/s)"(15.0 ("电动缸速度(mm/s)")) -> ()
            n647 = local write "夹头夹紧"(FALSE ("夹头夹紧")) -> ()
            n648 = local write "夹头松开"(TRUE ("夹头松开")) -> ()
          }
          frame #1 {
            n649 = while {
              stop <- w1100 stop-if-true
              n650 = local read "夹头松开"() -> (w1101:bool)
              n651 = local read "夹头夹紧"() -> (w1103:bool)
              n652 = Wait Until Next ms Multiple(millisecond multiple=u32 50 ("毫秒倍数")) -> ()  [unwired: 1 out]
              n653 = Not(x=w1103) -> (.not. x?=w1102:bool)
              n654 = And(x=w1102, y=w1101) -> (x .and. y?=w1100:bool)
            }
          }
          frame #2 {
            n655 = while {
              tunnel: [w1108] -> w1105
              stop <- w1107 stop-if-true
              n656 = local read "电动缸电机"() -> (w1109:u32)
              n657 = Wait Until Next ms Multiple(millisecond multiple=u32 50 ("毫秒倍数")) -> ()  [unwired: 1 out]
              n658 = local read "齿条右极限"() -> (w1106:dbl)
              n659 = call "PCI1240电动缸位置模式 .vi"("Distance"=w1106, "AxisHandle IN"=w1109) -> ("AbsSuccess"=w1107:bool, "AxisHandle OUT"=w1108:u32)  [unwired: 8 in]
            }
          }
          frame #3 {
            n660 = while {
              tunnel: w1112 -> [w1121]
              tunnel: [w1113] -> w1111
              stop <- w1114 stop-if-true
              n661 = local read "齿条推拉力(N)"() -> (w1119:dbl)
              n662 = Wait Until Next ms Multiple(millisecond multiple=u32 50 ("毫秒倍数")) -> ()  [unwired: 1 out]
              n663 = call <userlib>:"Acm_AxGetCmdVelocity.vi"("AxisHandle"=w1121) -> ("Velocity"=w1122:dbl, "AxisHandle"=w1113:u32)  [unwired: 1 in, 2 out]
              n664 = Equal To 0?(x=w1122) -> (x = 0?=w1116:bool)
              n665 = Absolute Value(x=w1119) -> (abs(x)=w1118:dbl)
              n666 = Greater Or Equal?(x=w1118, y=1000.0) -> (x >= y?=w1115:bool)
              n667 = Or(x=w1116, y=w1115) -> (x .or. y?=w1114:bool)
            }
          }
          frame #4 {
            n668 = while {
              tunnel: w1123 -> [w1127]
              tunnel: [w1126] -> _
              stop <- w1125 stop-if-true
              n669 = call "PCI1220U停止.vi"("AxisHandle IN"=w1127) -> ("完成"=w1125:bool, "AxisHandle OUT"=w1126:u32)  [unwired: 9 in]
              n670 = Wait (ms)(milliseconds to wait=u32 50 ("毫秒倍数")) -> ()  [unwired: 1 out]
            }
          }
          frame #5 {
            n671 = local write "旋转齿条轴使能"(TRUE ("旋转齿条轴使能")) -> ()
          }
          frame #6 {
            n672 = local read "旋转齿条电机"() -> (w1129:u32)
            n673 = Wait Until Next ms Multiple(millisecond multiple=u32 500 ("毫秒倍数")) -> ()  [unwired: 1 out]
          }
          frame #7 {
            n674 = call <userlib>:"Acm_AxHome.vi"("DirMode"=u32 0, "HomeMode"=u32 11, "AxisHandle"=w1132) -> ("AxisHandle"=w1131:u32)  [unwired: 1 in, 2 out]
          }
          frame #8 {
            n675 = Wait Until Next ms Multiple(millisecond multiple=u32 100 ("毫秒倍数")) -> ()  [unwired: 1 out]
          }
          frame #9 {
            n676 = while {
              tunnel: w1138 -> [w1141]
              tunnel: [w1140] -> w1137
              stop <- w1139 stop-if-true
              n677 = call <userlib>:"Acm_AxGetCmdVelocity.vi"("AxisHandle"=w1141) -> ("Velocity"=w1143:dbl, "AxisHandle"=w1140:u32)  [unwired: 1 in, 2 out]
              n678 = Wait Until Next ms Multiple(millisecond multiple=u32 50 ("毫秒倍数")) -> ()  [unwired: 1 out]
              n679 = Equal To 0?(x=w1143) -> (x = 0?=w1139:bool)
            }
          }
          frame #10 {
            n680 = call "PCI1220U角度置零.vi"("AxisHandle IN"=w1145) -> ("AxisHandle OUT"=w1144:u32)  [unwired: 10 in]
          }
          frame #11 {
            n681 = while {
              tunnel: w1147 -> [w1149]
              tunnel: [w1148] -> w1146
              stop <- w1152 stop-if-true
              n682 = Wait Until Next ms Multiple(millisecond multiple=u32 50 ("毫秒倍数")) -> ()  [unwired: 1 out]
              n683 = call "PCI1220U扭矩轴位置模式.vi"("Distance"=10.0, "AxisHandle IN"=w1149) -> ("AbsSuccess"=w1152:bool, "AxisHandle OUT"=w1148:u32)  [unwired: 8 in]
            }
          }
          frame #12 {
            n684 = Wait Until Next ms Multiple(millisecond multiple=u32 500 ("毫秒倍数")) -> ()  [unwired: 1 out]
          }
          frame #13 {
            n685 = while {
              tunnel: w1156 -> [w1159]
              tunnel: [w1158] -> w1155
              stop <- w1157 stop-if-true
              n686 = call <userlib>:"Acm_AxGetCmdVelocity.vi"("AxisHandle"=w1159) -> ("Velocity"=w1161:dbl, "AxisHandle"=w1158:u32)  [unwired: 1 in, 2 out]
              n687 = Wait Until Next ms Multiple(millisecond multiple=u32 50 ("毫秒倍数")) -> ()  [unwired: 1 out]
              n688 = Equal To 0?(x=w1161) -> (x = 0?=w1157:bool)
            }
          }
          frame #14 {
            n689 = call "PCI1220U角度置零.vi"("AxisHandle IN"=w1162) -> ()  [unwired: 10 in, 1 out]
          }
          frame #15 {
            n690 = while {
              tunnel: [w1166] -> w1163
              stop <- w1165 stop-if-true
              n691 = local read "电动缸电机"() -> (w1167:u32)
              n692 = Wait Until Next ms Multiple(millisecond multiple=u32 50 ("毫秒倍数")) -> ()  [unwired: 1 out]
              n693 = local read "齿条右极限"() -> (w1164:dbl)
              n694 = call "PCI1240电动缸位置模式 .vi"("Distance"=w1164, "AxisHandle IN"=w1167) -> ("AbsSuccess"=w1165:bool, "AxisHandle OUT"=w1166:u32)  [unwired: 8 in]
            }
          }
          frame #16 {
            n695 = while {
              tunnel: w1170 -> [w1178]
              tunnel: [w1176] -> w1169
              stop <- w1171 stop-if-true
              n696 = local read "齿条推拉力(N)"() -> (w1175:dbl)
              n697 = Wait Until Next ms Multiple(millisecond multiple=u32 50 ("毫秒倍数")) -> ()  [unwired: 1 out]
              n698 = call <userlib>:"Acm_AxGetCmdVelocity.vi"("AxisHandle"=w1178) -> ("Velocity"=w1179:dbl, "AxisHandle"=w1176:u32)  [unwired: 1 in, 2 out]
              n699 = Equal To 0?(x=w1179) -> (x = 0?=w1173:bool)
              n700 = Greater Or Equal?(x=w1175, y=300.0) -> (x >= y?=w1172:bool)
              n701 = Or(x=w1173, y=w1172) -> (x .or. y?=w1171:bool)
            }
          }
          frame #17 {
            n702 = while {
              tunnel: w1180 -> [w1184]
              tunnel: [w1183] -> _
              stop <- w1182 stop-if-true
              n703 = call "PCI1220U停止.vi"("AxisHandle IN"=w1184) -> ("完成"=w1182:bool, "AxisHandle OUT"=w1183:u32)  [unwired: 9 in]
              n704 = Wait (ms)(milliseconds to wait=u32 50 ("毫秒倍数")) -> ()  [unwired: 1 out]
            }
          }
          frame #18 {
            n705 = local write "工步号"(u32 100 ("工步号")) -> ()
          }
        }
      }
      frame 100 {
        n706 = flat-sequence {
          tunnel: [w1219] -> w1209
          tunnel: [w1217] -> w1208
          tunnel: [w1211] -> w1196
          tunnel: [w1210] -> w1193
          tunnel: w1209 -> [w1226]
          tunnel: w1208 -> [w1223]
          tunnel: ["F:\\报表存储\\" ("字符串")] -> w1207
          tunnel: w1196 -> [w1225]
          tunnel: [w1226] -> w1195
          tunnel: [w1225] -> w1194
          tunnel: w1193 -> [w1224]
          tunnel: [w1224] -> w1192
          tunnel: [w1223] -> w1191
          tunnel: w1207 -> [w1238]
          tunnel: [w1245] -> w1206
          tunnel: [w1243] -> w1205
          tunnel: [w1242] -> w1204
          tunnel: [w1241] -> w1203
          tunnel: w1195 -> [w1237]
          tunnel: w1194 -> [w1236]
          tunnel: w1192 -> [w1235]
          tunnel: w1191 -> [w1228]
          tunnel: [w1230] -> w1186
          tunnel: w1206 -> [w1252]
          tunnel: [w1253] -> w1202
          tunnel: w1205 -> [w1253]
          tunnel: w1204 -> [w1251]
          tunnel: w1203 -> [w1250]
          tunnel: [w1249] -> w1201
          tunnel: [w1248] -> w1200
          tunnel: [w1247] -> w1187
          tunnel: w1186 -> [w1247]
          tunnel: [w1260] -> w1199
          tunnel: w1202 -> [w1260]
          tunnel: w1201 -> [w1259]
          tunnel: [w1259] -> w1198
          tunnel: [w1258] -> w1197
          tunnel: w1200 -> [w1258]
          tunnel: [w1256] -> w1188
          tunnel: w1187 -> [w1256]
          tunnel: w1199 -> [w1263]
          tunnel: w1198 -> [w1271]
          tunnel: w1197 -> [w1270]
          tunnel: [w1262] -> w1189
          tunnel: w1188 -> [w1262]
          tunnel: [w1279] -> w1190
          tunnel: w1189 -> [w1279]
          tunnel: w1190 -> [w1281]
          frame #0 {
            n707 = local read "产品ID"() -> (w1218:string)
            n708 = Format Date/Time String(time format string (%c)="%Y%m%d" ("时间格式字符串(%c)")) -> (date/time string=w1212:string)  [unwired: 2 in]
            n709 = String Subset(string=w1212, offset (0)=6 ("偏移量(0)"), length (rest)=2 ("长度（剩余）")) -> (substring=w1210:string)
            n710 = String Subset(string=w1212, offset (0)=4 ("偏移量(0)"), length (rest)=2 ("长度（剩余）")) -> (substring=w1211:string)
            n711 = String Subset(string=w1212, offset (0)=0 ("偏移量(0)"), length (rest)=4 ("长度（剩余）")) -> (substring=w1219:string)
            n712 = call <vilib>:"Trim Whitespace.vi"("string"=w1218) -> ("trimmed string"=w1217:string)  [unwired: 1 in]
          }
          frame #1 {
          }
          frame #2 {
            w1229 = "\\" ("字符串")
            n713 = Concatenate Strings(w1238, w1237, w1229, w1236, w1229, w1235, w1229, w1228, w1229) -> (w1232:string)
            n714 = Concatenate Strings(w1238, w1237, w1229, w1236, w1229, w1235, w1229, w1228, w1229) -> (w1246:string)
            n715 = Concatenate Strings(w1232, w1228, "间隙曲线.JPG" ("字符串")) -> (w1244:string)
            n716 = Concatenate Strings(w1232, "轴向力曲线数组.txt" ("字符串")) -> (w1241:string)
            n717 = Concatenate Strings(w1232, "扭动曲线数组.txt" ("字符串")) -> (w1242:string)
            n718 = Concatenate Strings(w1232, w1228, "轴向力曲线.JPG" ("字符串")) -> (w1234:string)
            n719 = String To Path(string=w1244) -> (path=w1243:path)
            n720 = String To Path(string=w1246) -> (path=w1245:path)
            n721 = String To Path(string=w1234) -> (path=w1230:path)
          }
          frame #3 {
            n722 = call <vilib>:"Check if File or Folder Exists.vi"("path"=w1252) -> ("file or folder exists?"=w1254:bool)  [unwired: 8 in, 2 out]
            n723 = case shown="假" w1254 {
              tunnel: w1252 -> [w1255 _]
              frame False {
                n724 = Create Folder(path (use dialog)=w1255) -> ()  [unwired: 2 in, 3 out]
              }
              frame True {
              }
            }
            n725 = String To Path(string=w1250) -> (path=w1248:path)
            n726 = String To Path(string=w1251) -> (path=w1249:path)
          }
          frame #4 {
            n727 = local write "选项卡控件"(T1."间隙测量" ("选项卡控件")) -> ()
            n728 = Wait Until Next ms Multiple(millisecond multiple=u32 1000 ("毫秒倍数")) -> ()  [unwired: 1 out]
          }
          frame #5 {
            n729 = disable-structure shown="禁用" {
              disable-tunnel: w1263 -> [w1272 _]
              frame Disabled {
                w1276 = T2 2 items=["快速打印", "标准报表", "HTML", "双字节", "Excel"] ("report type (Quick Print)")
                w1275 = T3 1 items=["完整前面板", "前面板可见部分", "图标、说明、前面板和程序框图", "说明信息: 使用前面板", "说明信息: 作为子VI使用", "说明信息: 完整", "说明信息: 自定义"] ("contents (complete front panel)")
                n730 = Current VI's Path() -> (path=w1274:path)
                n731 = call-poly <vilib>:"Easy Print VI Panel or Documentation.vi"("report type (Quick Print)"=w1276, "contents (complete front panel)"=w1275, "VI path"=w1274) -> ("error out"=w1278:errorcluster, "report out"=w1277:refnum<class "NI_report.lvclass">)  [unwired: 1 in, 6 out]
                n732 = call-dynamic "Save Report to File.vi"("report in"=w1277, "report file path"=w1272, "error in (no error)"=w1278) -> ("error out"=→"error out 3":errorcluster)  [unwired: 2 in, 10 out]
              }
              frame Enabled {
              }
            }
            n733 = local read "间隙Y数组"() -> (w1268:dbl[])
            n734 = local read "间隙X数组"() -> (w1269:dbl[])
            n735 = local read "轴向力Y"() -> (w1266:dbl[])
            n736 = local read "轴向力X"() -> (w1267:dbl[])
            n737 = call "导出曲线数组.vi"("file path (dialog if empty)"=w1271, "数组 2"=w1268, "数组"=w1269) -> ()  [unwired: 9 in]
            n738 = call "导出曲线数组.vi"("file path (dialog if empty)"=w1270, "数组 2"=w1266, "数组"=w1267) -> ()  [unwired: 9 in]
            n739 = control-ref of="本VI"() -> (w1265:refnum<vi>)
            n740 = invoke class="VI" method="FP.Get Image"(reference=w1265) -> ("image data"=w1264:T4)  [unwired: 5 in, 5 out]
            n741 = call <vilib>:"Write JPEG File.vi"("image data"=w1264, "path to JPEG file"=w1263) -> ()  [unwired: 8 in, 2 out]
          }
          frame #6 {
            n742 = local write "选项卡控件"(T1."轴向力测量" ("选项卡控件")) -> ()
          }
          frame #7 {
            n743 = control-ref of="本VI"() -> (w1282:refnum<vi>)
            n744 = invoke class="VI" method="FP.Get Image"(reference=w1282) -> ("image data"=w1283:T4)  [unwired: 5 in, 5 out]
            n745 = call <vilib>:"Write JPEG File.vi"("image data"=w1283, "path to JPEG file"=w1281) -> ()  [unwired: 8 in, 2 out]
          }
          frame #8 {
            n746 = local read "联线按钮"() -> (w1284:bool)
            n747 = case shown="真" w1284 {
              frame False {
              }
              frame True {
                n748 = flat-sequence {
                  tunnel: [w1287] -> w1285
                  tunnel: [w1315] -> w1286
                  tunnel: w1285 -> [w1311]
                  tunnel: w1286 -> [w1327]
                  frame #0 {
                    n749 = local read "轴向力及全行程间隙合格"() -> (w1288:bool)
                    n750 = local read "单点间隙合格"() -> (w1289:bool)
                    n751 = And(x=w1289, y=w1288) -> (x .and. y?=w1287:bool)
                  }
                  frame #1 {
                    w1309 = i16 3 ("精度(6)")
                    n752 = local read "右180°内全行程间隙"() -> (w1308:dbl)
                    n753 = local read "右180°外全行程间隙"() -> (w1301:dbl)
                    n754 = local read "左180°外全行程间隙"() -> (w1300:dbl)
                    n755 = local read "左180°内全行程间隙"() -> (w1318:dbl)
                    n756 = local read "右最大轴向力(N)"() -> (w1303:dbl)
                    n757 = local read "左轴向力波动(N)"() -> (w1304:dbl)
                    n758 = local read "左最大轴向力(N)"() -> (w1302:dbl)
                    n759 = local read "员工ID"() -> (w1290:string)
                    n760 = local read "右轴向力波动(N)"() -> (w1305:dbl)
                    n761 = Boolean To (0,1)(Boolean=w1311) -> (0, 1=w1313:i16)
                    n762 = local read "中间位置间隙"() -> (w1320:dbl)
                    n763 = local read "总圈数"() -> (w1307:dbl)
                    n764 = local read "总行程"() -> (w1306:dbl)
                    n765 = local read "FGCS"() -> (w1322:string)
                    n766 = local read "KSJJ"() -> (w1324:string)
                    n767 = local read "产品ID"() -> (w1325:string)
                    n768 = Number To Decimal String(number=w1313, width (-)=i16 1 ("宽度(-)")) -> (decimal integer string=w1310:string)
                    n769 = Format Date/Time String(time format string (%c)="%Y%m%d%H%M" ("时间格式字符串(%c)")) -> (date/time string=w1323:string)  [unwired: 2 in]
                    n770 = Number To Fractional String(number=w1306, precision (6)=w1309) -> (F-format string=w1292:string)  [unwired: 2 in]
                    n771 = Number To Fractional String(number=w1301, precision (6)=w1309) -> (F-format string=w1297:string)  [unwired: 2 in]
                    n772 = Number To Fractional String(number=w1304, precision (6)=w1309) -> (F-format string=w1294:string)  [unwired: 2 in]
                    n773 = Number To Fractional String(number=w1308, precision (6)=w1309) -> (F-format string=w1299:string)  [unwired: 2 in]
                    n774 = Number To Fractional String(number=w1303, precision (6)=w1309) -> (F-format string=w1295:string)  [unwired: 2 in]
                    n775 = Number To Fractional String(number=w1305, precision (6)=w1309) -> (F-format string=w1293:string)  [unwired: 2 in]
                    n776 = Number To Fractional String(number=w1318, precision (6)=w1309) -> (F-format string=w1316:string)  [unwired: 2 in]
                    n777 = Number To Fractional String(number=w1302, precision (6)=w1309) -> (F-format string=w1296:string)  [unwired: 2 in]
                    n778 = Number To Fractional String(number=w1307, precision (6)=w1309) -> (F-format string=w1291:string)  [unwired: 2 in]
                    n779 = Number To Fractional String(number=w1300, precision (6)=w1309) -> (F-format string=w1298:string)  [unwired: 2 in]
                    n780 = Number To Fractional String(number=w1320, precision (6)=i16 3 ("精度(6)")) -> (F-format string=w1317:string)  [unwired: 2 in]
                    n781 = Build Array(w1325, w1290, "1", w1310, w1324, w1323, w1322, "Q14073-11A", w1317, w1316, w1299, w1298, w1297, w1296, w1295, w1294, w1293, w1292, w1291) -> (w1315:string[])
                  }
                  frame #2 {
                    n782 = Wait (ms)(milliseconds to wait=u32 500 ("等待时间（毫秒）")) -> ()  [unwired: 1 out]
                    n783 = call "数据库更新.vi"("设备号"="06", "数据"=w1327) -> ()  [unwired: 13 in, 1 out]
                  }
                  frame #3 {
                  }
                }
              }
            }
          }
          frame #9 {
            n784 = local write "产品ID"("") -> ()
            n785 = local write "工步号"(u32 0 ("工步号")) -> ()
          }
        }
      }
    }
    n786 = Wait (ms)(milliseconds to wait=u32 50 ("毫秒倍数")) -> ()  [unwired: 1 out]
    n787 = local read "停止"() -> (w7:bool)
  }
  n788 = while {
    stop <- w1332 stop-if-true
    n789 = event shown="[1] \"停止\": 值改变" {
      selector: _ -> [_ _ _ _ _ _]
      dyn-events: _ -> [_ _ _ _ _ _]
      timeout: 500 -> [_ _ _ _ _ _]
      event Timeout {
        n790 = event-data() -> ()  [unwired: 3 out]
      }
      event "停止": Value Change {
        n791 = event-data() -> ()  [unwired: 6 out]
        n792 = flat-sequence {
          frame #0 {
            n793 = Wait (ms)(milliseconds to wait=u32 1000 ("毫秒倍数")) -> ()  [unwired: 1 out]
          }
          frame #1 {
            n794 = Quit LabVIEW(quit? (T)=TRUE ("停止？(T)")) -> ()
          }
        }
      }
      event "参数修改": Value Change {
        n795 = event-data() -> ()  [unwired: 6 out]
        n796 = while {
          i -> [w1339]
          stop <- w1338 stop-if-true
          n797 = local read "参数浏览表"() -> (w1341:string[][])
          n798 = local read "型号数量"() -> (w1340:i32)
          n799 = Wait Until Next ms Multiple(millisecond multiple=u32 50 ("毫秒倍数")) -> ()  [unwired: 1 out]
          n800 = Greater Or Equal?(x=w1339, y=w1340) -> (x >= y?=w1338:bool)
          n801 = Index Array(array=w1341, index (col)=w1339) -> (element=w1337:string[])  [unwired: 1 in]
          n802 = stacked-sequence {
            tunnel: w1337 -> [w1377]
            frame #0 {
              n803 = Index Array(array=w1377, index #1=0 ("索引"), index #2=2 ("索引"), index #3=3 ("索引"), index #4=4 ("索引"), index #5=5 ("索引"), index #6=6 ("索引"), index #7=7 ("索引"), index #8=8 ("索引"), index #9=9 ("索引"), index #10=10 ("索引"), index #11=11 ("索引"), index #12=12 ("索引"), index #13=13 ("索引"), index #14=14 ("索引"), index #15=15 ("索引"), index #16=16 ("索引"), index #17=17 ("索引"), index #18=18 ("索引"), index #19=19 ("索引"), index #20=20 ("索引")) -> (element #1=w1344:string, element #2=w1373:string, element #3=w1372:string, element #4=w1371:string, element #5=w1370:string, element #6=w1369:string, element #7=w1368:string, element #8=w1367:string, element #9=w1366:string, element #10=w1365:string, element #11=w1364:string, element #12=w1355:string, element #13=w1354:string, element #14=w1353:string, element #15=w1352:string, element #16=w1351:string, element #17=w1350:string, element #18=w1347:string, element #19=w1346:string, element #20=w1343:string)
              n804 = local read "ADODB._Connection Out 2"() -> (w1362:refnum<k7>)
              n805 = call "创建文本"("测头机构轴移动速度"=w1373, "测头机构轴检测位"=w1372, "测头机构轴待检位"=w1371, "测头机构轴后退位"=w1370, "齿条移动速度"=w1369, "齿条左极限"=w1368, "齿条右极限"=w1367, "旋转齿条轴找帽转速"=w1366, "旋转齿条轴测量转速"=w1365, "测量点扭矩"=w1364, "总行程最小值"=w1355, "总行程最大值"=w1354, "最大轴向力"=w1353, "轴向力波动"=w1352, "平均轴向力最小值"=w1351, "平均轴向力最大值"=w1350, "总圈数最小值"=w1347, "总圈数最大值"=w1346, "中间位置"=w1343, "产品型号"=w1344) -> ("Result"=w1363:string)  [unwired: 6 in, 1 out]
              n806 = call "SQL Execute.vi"("Command Text"=w1363, "ADODB._Connection In"=w1362) -> ("error out"=w1375:errorcluster, "ADODB._Connection Out"=w1376:refnum<k7>)  [unwired: 6 in, 2 out]
              n807 = call "ADO Connection Close.vi"("error in (no error)"=w1375, "ADODB._Connection In"=w1376) -> ("error out"=→"error out":errorcluster)  [unwired: 8 in, 1 out]
            }
          }
        }
      }
      event "参数查询": Value Change {
        n808 = event-data() -> ()  [unwired: 6 out]
        n809 = flat-sequence {
          tunnel: [w1400] -> w1393
          tunnel: [w1399] -> w1392
          tunnel: [w1398] -> w1389
          tunnel: w1393 -> [w1404]
          tunnel: w1392 -> [w1406]
          tunnel: [w1406] -> w1391
          tunnel: [w1405] -> w1390
          tunnel: w1389 -> [w1405]
          tunnel: w1391 -> [_]
          tunnel: w1390 -> [_]
          frame #0 {
            n810 = call-poly <vilib>:"Read From Spreadsheet File.vi"("file path (dialog if empty)"=path "D:/Q14070-Z060人机界面/参数/参数项.txt") -> ("first row"=w1394:string[])  [unwired: 6 in, 4 out]
            n811 = property on="参数浏览表" class="Tbl (严格)"("Row Headers[]"=w1394) -> ()  [unwired: 2 in, 2 out]
          }
          frame #1 {
            n812 = local read "ADODB._Connection Out 2"() -> (w1397:refnum<k7>)
            n813 = call "SQL Execute.vi"("Command Text"="SELECT * FROM 测试参数表;", "ADODB._Connection In"=w1397) -> ("error out"=w1398:errorcluster, "Data"=w1402:string[][], "ADODB._Connection Out"=w1399:refnum<k7>)  [unwired: 6 in, 1 out]
            n814 = Transpose 2D Array "二维数组转置"(2D array=w1402) -> (transposed array=w1400:string[][])
            n815 = Index Array(array=w1400, index (row)=0 ("索引 (行)")) -> (element=w1401:string[])  [unwired: 1 in]
            n816 = property on="参数浏览表" class="Tbl (严格)"("Column Headers[]"=w1401) -> ()  [unwired: 2 in, 2 out]
          }
          frame #2 {
            n817 = local write "参数浏览表"(w1404) -> ()
          }
          frame #3 {
          }
        }
      }
      event "传感器参数保存": Value Change {
        n818 = event-data() -> ()  [unwired: 6 out]
        n819 = flat-sequence {
          frame #0 {
            n820 = local read "齿条推拉力零点偏移"() -> (w1411:dbl)
            n821 = local read "齿条推拉力比例偏移"() -> (w1407:dbl)
            n822 = local read "间隙位移零点偏移"() -> (w1418:dbl)
            n823 = local read "齿条扭矩零点偏移"() -> (w1410:dbl)
            n824 = local read "间隙位移比例偏移"() -> (w1408:dbl)
            n825 = local read "齿条扭矩比例偏移"() -> (w1409:dbl)
            n826 = local read "ADODB._Connection Out 2"() -> (w1426:refnum<k7>)
            n827 = Number To Fractional String(number=w1418, precision (6)=i16 2 ("精度(6)")) -> (F-format string=w1425:string)  [unwired: 2 in]
            n828 = Number To Fractional String(number=w1411, precision (6)=i16 2 ("精度(6)")) -> (F-format string=w1424:string)  [unwired: 2 in]
            n829 = Number To Fractional String(number=w1410, precision (6)=i16 2 ("精度(6)")) -> (F-format string=w1423:string)  [unwired: 2 in]
            n830 = Number To Fractional String(number=w1408, precision (6)=i16 2 ("精度(6)")) -> (F-format string=w1422:string)  [unwired: 2 in]
            n831 = Number To Fractional String(number=w1407, precision (6)=i16 2 ("精度(6)")) -> (F-format string=w1421:string)  [unwired: 2 in]
            n832 = Number To Fractional String(number=w1409, precision (6)=i16 2 ("精度(6)")) -> (F-format string=w1420:string)  [unwired: 2 in]
            n833 = call "创建文本3"("4"=w1422, "6"=w1420, "1"=w1425, "2"=w1424, "3"=w1423, "5"=w1421) -> ("Result"=w1427:string)  [unwired: 8 in, 1 out]
            n834 = call "SQL Execute.vi"("Command Text"=w1427, "ADODB._Connection In"=w1426) -> ("error out"=→"error out 4":errorcluster)  [unwired: 6 in, 3 out]
          }
        }
      }
      event "产品ID": Value Change {
        n835 = event-data() -> ()  [unwired: 7 out]
        n836 = Format Date/Time String(time format string (%c)="%Y%m%d%H%M" ("时间格式字符串(%c)")) -> (date/time string=w1428:string)  [unwired: 2 in]
        n837 = local write "KSJJ"(w1428) -> ()
      }
    }
    n838 = Wait (ms)(milliseconds to wait=u32 50 ("毫秒倍数")) -> ()  [unwired: 1 out]
    n839 = local read "停止"() -> (w1332:bool)
  }
  n840 = while {
    stop <- w1431 stop-if-true
    n841 = stacked-sequence {
      frame #0 {
        n842 = flat-sequence {
          frame #0 {
          }
          frame #1 {
            "PLC" <- "阻挡"
          }
          frame #2 {
            n843 = First Call?() -> (First Call?: T/F=w1433:bool)
            n844 = case shown="真" w1433 {
              frame False {
              }
              frame True {
                n845 = call "员工管理测试程序.vi"() -> ("员工姓名"=w1435:string, "员工ID"=w1434:string)  [unwired: 10 in]
                n846 = local write "员工ID"(w1434) -> ()
                n847 = local write "员工姓名"(w1435) -> ()
              }
            }
          }
          frame #3 {
          }
          frame #4 {
          }
          frame #5 {
          }
          frame #6 {
          }
        }
      }
      frame #1 {
        n848 = flat-sequence {
          frame #0 {
            n849 = property on="型号选择" class="Ring (严格)"() -> ("RingText.Text"=w1439:string)  [unwired: 2 in, 2 out]
            n850 = case shown="\"J728\"" w1439 {
              frame "J709", Default {
                w1440 = FALSE ("可见")
                w1441 = TRUE ("可见")
                n851 = property on="右180°内全行程间隙" class="DigNum (严格)"("Visible"=w1440) -> ()  [unwired: 2 in, 2 out]
                n852 = property on="右180°外全行程间隙" class="DigNum (严格)"("Visible"=w1440) -> ()  [unwired: 2 in, 2 out]
                n853 = property on="左180°外全行程间隙" class="DigNum (严格)"("Visible"=w1440) -> ()  [unwired: 2 in, 2 out]
                n854 = property on="左180°内全行程间隙" class="DigNum (严格)"("Visible"=w1440) -> ()  [unwired: 2 in, 2 out]
                n855 = property on="右全行程间隙" class="DigNum (严格)"("Visible"=w1441) -> ()  [unwired: 2 in, 2 out]
                n856 = property on="左全行程间隙" class="DigNum (严格)"("Visible"=w1441) -> ()  [unwired: 2 in, 2 out]
              }
              frame "J706" {
                w1442 = TRUE ("可见")
                w1443 = FALSE ("可见")
                n857 = property on="右180°内全行程间隙" class="DigNum (严格)"("Visible"=w1442) -> ()  [unwired: 2 in, 2 out]
                n858 = property on="右180°外全行程间隙" class="DigNum (严格)"("Visible"=w1442) -> ()  [unwired: 2 in, 2 out]
                n859 = property on="左180°外全行程间隙" class="DigNum (严格)"("Visible"=w1442) -> ()  [unwired: 2 in, 2 out]
                n860 = property on="左180°内全行程间隙" class="DigNum (严格)"("Visible"=w1442) -> ()  [unwired: 2 in, 2 out]
                n861 = property on="右全行程间隙" class="DigNum (严格)"("Visible"=w1443) -> ()  [unwired: 2 in, 2 out]
                n862 = property on="左全行程间隙" class="DigNum (严格)"("Visible"=w1443) -> ()  [unwired: 2 in, 2 out]
              }
              frame "J728" {
                w1444 = TRUE ("可见")
                w1445 = FALSE ("可见")
                n863 = property on="右180°内全行程间隙" class="DigNum (严格)"("Visible"=w1444) -> ()  [unwired: 2 in, 2 out]
                n864 = property on="右180°外全行程间隙" class="DigNum (严格)"("Visible"=w1444) -> ()  [unwired: 2 in, 2 out]
                n865 = property on="左180°外全行程间隙" class="DigNum (严格)"("Visible"=w1444) -> ()  [unwired: 2 in, 2 out]
                n866 = property on="左180°内全行程间隙" class="DigNum (严格)"("Visible"=w1444) -> ()  [unwired: 2 in, 2 out]
                n867 = property on="右全行程间隙" class="DigNum (严格)"("Visible"=w1445) -> ()  [unwired: 2 in, 2 out]
                n868 = property on="左全行程间隙" class="DigNum (严格)"("Visible"=w1445) -> ()  [unwired: 2 in, 2 out]
              }
            }
          }
          frame #1 {
            (unwired) string[] ["I急停按钮", "I自动旋钮", "I启动按钮", "I备用按钮", "I复位按钮", "I上阻挡器放行", "I下阻挡器放行", "I进支线按钮"] ("I0说明")
            (unwired) string[] ["I出支线按钮", "I主线顶升按钮", "I主线下降按钮", "I支线顶升按钮", "I支线下降按钮", "I气压报警", "未使用", "未使用"] ("I0说明")
            n869 = local read "间隙位移(mm)"() -> (w1448:dbl)
            n870 = Greater Or Equal?(x=w1448, y=4.0) -> (x >= y?=w1446:bool)
            n871 = case shown="真" w1446 {
              frame False {
              }
              frame True {
                n872 = local write "测头机构轴使能"(FALSE ("测头机构轴使能")) -> ()
              }
            }
          }
          frame #2 {
            (unwired) string[] ["I电动缸SRDY", "I电动缸ZSPD", "I电动缸ALRM", "I间隙进给SRDY", "I间隙进给ZSPD", "I间隙进给ALRM", "I间隙旋转SRPD", "I间隙旋转ZSPD"] ("I0说明")
            n873 = local read "测头机构轴位置(mm)"() -> (w1452:dbl)
            n874 = Greater Or Equal?(x=w1452, y=90.0) -> (x >= y?=w1450:bool)
            n875 = case shown="假" w1450 {
              frame False {
                w1453 = T5."Enabled" ("禁用")
                n876 = property on="测头气缸右移" class="Bool"("DisabledEnum"=w1453) -> ()  [unwired: 2 in, 2 out]
                n877 = property on="测头气缸左移" class="Bool"("DisabledEnum"=w1453) -> ()  [unwired: 2 in, 2 out]
                n878 = property on="测头气缸右移" class="Bool (严格)"("DisabledEnum"=w1453) -> ()  [unwired: 2 in, 2 out]
                n879 = property on="测头气缸左移" class="Bool (严格)"("DisabledEnum"=w1453) -> ()  [unwired: 2 in, 2 out]
              }
              frame True {
                w1454 = T5."Disabled" ("禁用")
                w1455 = FALSE ("测头气缸右移")
                n880 = local write "测头气缸右移"(w1455) -> ()
                n881 = local write "测头气缸左移"(w1455) -> ()
                n882 = property on="测头气缸右移" class="Bool"("DisabledEnum"=w1454) -> ()  [unwired: 2 in, 2 out]
                n883 = property on="测头气缸左移" class="Bool"("DisabledEnum"=w1454) -> ()  [unwired: 2 in, 2 out]
                n884 = property on="测头气缸右移" class="Bool (严格)"("DisabledEnum"=w1454) -> ()  [unwired: 2 in, 2 out]
                n885 = property on="测头气缸左移" class="Bool (严格)"("DisabledEnum"=w1454) -> ()  [unwired: 2 in, 2 out]
              }
            }
          }
          frame #3 {
            (unwired) string[] ["I间隙旋转ALRM", "I扭矩旋转SRPD", "I扭矩旋转ZSPD", "I扭矩旋转ALRM", "I拧紧机合格", "I拧紧机不合格", "I拧紧机报警", "未使用"] ("I0说明")
          }
        }
        n886 = local read "急停"() -> (w1438:bool)
        n887 = local read "复位"() -> (w1437:bool)
        n888 = Compound Arithmetic op=OR(invert w1438, w1437) -> (→"循环退出":bool)
      }
      frame #2 {
        n889 = flat-sequence {
          frame #0 {
            (unwired) string[] ["I自制气缸进位", "I自制气缸原位", "I上工位检测", "I本工位检测", "I下工位检测", "I主线顶升上位", "I主线顶升下位", "I支线顶升上位"] ("I0说明")
          }
          frame #1 {
            (unwired) string[] ["I支线顶升下位", "I支线进到位", "I支线退到位", "I位移气缸原位", "I位移气缸进位", "I拧紧机在位", "I电动缸原位", "I电动缸进位"] ("I0说明")
          }
          frame #2 {
            (unwired) string[] ["未使用", "未使用", "未使用", "未使用", "未使用", "未使用", "未使用", "未使用"] ("I0说明")
          }
          frame #3 {
            (unwired) string[] ["未使用", "未使用", "未使用", "未使用", "未使用", "未使用", "未使用", "未使用"] ("I0说明")
          }
        }
        n890 = local read "本测试状态"() -> (w1457:bool)
        n891 = local read "本自动状态"() -> (w1458:bool)
        n892 = local read "本备料状态"() -> (w1456:bool)
        n893 = local write "本测试状态H"(w1457) -> ()
        n894 = local write "本自动状态H"(w1458) -> ()
        n895 = local write "本备料状态H"(w1456) -> ()
      }
      frame #3 {
        n896 = local read "报警工步号"() -> (w1460:dbl)
        n897 = local read "工步号"() -> (w1462:u32)
        n898 = case shown="0, 默认" w1462 {
          tunnel: [w1472 "请取胶瓶" ("工步描述") "请对锁紧螺母加力" ("工步描述") "灵敏度测试中" ("工步描述") "有油刚度测试中" ("工步描述") "安装好锁紧螺母后，按顶升按钮，夹具夹紧" ("工步描述") "请点击启动按钮进行试验" ("工步描述") "探头气缸右移" ("工步描述") "电动缸前进找中" ("工步描述") "探头前进测试开始" ("工步描述") "探头退回" ("工步描述") "轴向力测试中" ("工步描述") "测头后退夹抓松开" ("工步描述") "伺服回零" ("工步描述") "力特性试验完成" ("工步描述") "套好输出轴把手，按启动按钮，做回正力试验" ("工步描述") "回正力试验中" ("工步描述") "试验完成，将把手拉回，取下油管，按顶升按钮" ("工步描述") "拆下锁紧螺母和输入轴万向节，按顶升按钮" ("工步描述")] -> w1461
          frame 0, Default {
            n899 = local read "联线按钮"() -> (w1471:bool)
            n900 = case shown="真" w1471 {
              tunnel: ["等待工件" ("工步描述") "等待扫描条码" ("工步描述")] -> w1472
              frame False {
              }
              frame True {
              }
            }
          }
          frame 1 {
          }
          frame 2 {
          }
          frame 3 {
          }
          frame 4 {
          }
          frame 5 {
          }
          frame 6 {
          }
          frame 10 {
          }
          frame 15 {
          }
          frame 20 {
          }
          frame 30 {
          }
          frame 40 {
          }
          frame 45 {
          }
          frame 50 {
          }
          frame 55 {
          }
          frame 60 {
          }
          frame 70 {
          }
          frame 80 {
          }
          frame 56 {
          }
        }
        "工步提示" <- w1461
        n901 = case shown="3" w1460 {
          tunnel: [_ "操作步骤错请取胶瓶" "操作步骤错误请点标" "测头气缸不在原位" "急停被按下" "气压报警" "电动缸伺服报警" "旋转伺服服报警" "测头伺服服报警"] -> w1459
          frame 0, Default {
          }
          frame 1 {
          }
          frame 3 {
          }
          frame 2 {
          }
          frame 4 {
          }
          frame 5 {
          }
          frame 6 {
          }
          frame 7 {
          }
          frame 8 {
          }
        }
        "报警提示" <- w1459
      }
      frame #4 {
        n902 = local read "急停"() -> (w1494:bool)
        n903 = local read "红灯"() -> (w1493:bool)
        n904 = local read "复位"() -> (w1496:bool)
        n905 = local read "红灯"() -> (w1495:bool)
        n906 = case shown="假" w1494 {
          frame False {
            n907 = local write "红灯"(TRUE ("红灯")) -> ()
          }
          frame True {
            n908 = local write "红灯"(FALSE ("复位")) -> ()
          }
        }
        n909 = case shown="真" w1493 {
          frame False {
          }
          frame True {
            n910 = local write "回零完成"(FALSE ("夹头夹紧控制")) -> ()
          }
        }
        n911 = local read "停止"() -> (w1498:bool)
        n912 = Compound Arithmetic op=OR(w1496, w1498, w1495) -> (w1497:bool)
        n913 = case shown="真" w1497 {
          frame False {
          }
          frame True {
            n914 = local read "测头机构电机"() -> (w1502:u32)
            n915 = local read "旋转齿条电机"() -> (w1503:u32)
            n916 = local read "电动缸电机"() -> (w1504:u32)
            n917 = call "PCI1220U停止.vi"("AxisHandle IN"=w1503) -> ()  [unwired: 9 in, 2 out]
            n918 = call "PCI1220U停止.vi"("AxisHandle IN"=w1504) -> ()  [unwired: 9 in, 2 out]
            n919 = call "PCI1220U停止.vi"("AxisHandle IN"=w1502) -> ()  [unwired: 9 in, 2 out]
          }
        }
      }
      frame #5 {
        n920 = local read "齿条扭矩(Nm)"() -> (w1507:dbl)
        n921 = local read "黄灯"() -> (w1505:bool)
        n922 = local read "旋转齿条轴左转"() -> (w1513:bool)
        n923 = Absolute Value(x=w1507) -> (abs(x)=w1512:dbl)
        n924 = local read "旋转齿条轴右转"() -> (w1508:bool)
        n925 = Not(x=w1513) -> (.not. x?=w1509:bool)
        n926 = Less?(x=w1512, y=20.0) -> (x < y?=w1510:bool)
        n927 = Compound Arithmetic op=AND(w1508, w1509, w1510, w1505) -> (w1506:bool)
        n928 = case shown="真" w1506 {
          frame False {
          }
          frame True {
            n929 = flat-sequence {
              tunnel: [w1517] -> w1515
              tunnel: w1515 -> [w1519]
              tunnel: [w1519] -> w1514
              tunnel: w1514 -> [w1530]
              frame #0 {
                n930 = local read "旋转齿条电机"() -> (w1516:u32)
                n931 = call "PCI1220U运行.vi"("方向"=enum32{"Negative", "Positive"}."Negative" ("Direction"), "AxisHandle IN"=w1516) -> ("AxisHandle OUT"=w1517:u32)  [unwired: 9 in]
              }
              frame #1 {
                n932 = while {
                  stop <- w1523 stop-if-true
                  n933 = Wait (ms)(milliseconds to wait=u32 50 ("毫秒倍数")) -> ()  [unwired: 1 out]
                  n934 = local read "齿条扭矩(Nm)"() -> (w1528:dbl)
                  n935 = local read "旋转齿条轴右转"() -> (w1525:bool)
                  n936 = local read "红灯"() -> (w1520:bool)
                  n937 = local read "复位"() -> (w1521:bool)
                  n938 = Absolute Value(x=w1528) -> (abs(x)=w1527:dbl)
                  n939 = Not(x=w1525) -> (.not. x?=w1522:bool)
                  n940 = Greater?(x=w1527, y=10.0) -> (0:w1524:bool)
                  n941 = Compound Arithmetic op=OR(w1524, w1522, w1521, w1520) -> (w1523:bool)
                }
              }
              frame #2 {
                n942 = call "PCI1220U停止.vi"("AxisHandle IN"=w1530) -> ()  [unwired: 9 in, 2 out]
              }
            }
          }
        }
      }
      frame #6 {
        n943 = local read "齿条扭矩(Nm)"() -> (w1535:dbl)
        n944 = local read "旋转齿条轴右转"() -> (w1539:bool)
        n945 = Absolute Value(x=w1535) -> (abs(x)=w1534:dbl)
        n946 = local read "旋转齿条轴左转"() -> (w1537:bool)
        n947 = local read "黄灯"() -> (w1531:bool)
        n948 = Not(x=w1539) -> (.not. x?=w1536:bool)
        n949 = Less?(x=w1534, y=20.0) -> (x < y?=w1532:bool)
        n950 = Compound Arithmetic op=AND(w1537, w1536, w1532, w1531) -> (w1538:bool)
        n951 = case shown="真" w1538 {
          frame False {
          }
          frame True {
            n952 = flat-sequence {
              tunnel: [w1543] -> w1541
              tunnel: w1541 -> [w1545]
              tunnel: [w1545] -> w1540
              tunnel: w1540 -> [w1556]
              frame #0 {
                n953 = local read "旋转齿条电机"() -> (w1542:u32)
                n954 = call "PCI1220U运行.vi"("方向"=enum32{"Negative", "Positive"}."Positive" ("Direction"), "AxisHandle IN"=w1542) -> ("AxisHandle OUT"=w1543:u32)  [unwired: 9 in]
              }
              frame #1 {
                n955 = while {
                  stop <- w1548 stop-if-true
                  n956 = Wait (ms)(milliseconds to wait=u32 50 ("毫秒倍数")) -> ()  [unwired: 1 out]
                  n957 = local read "齿条扭矩(Nm)"() -> (w1554:dbl)
                  n958 = local read "旋转齿条轴左转"() -> (w1551:bool)
                  n959 = local read "红灯"() -> (w1546:bool)
                  n960 = local read "复位"() -> (w1547:bool)
                  n961 = Absolute Value(x=w1554) -> (abs(x)=w1553:dbl)
                  n962 = Not(x=w1551) -> (.not. x?=w1549:bool)
                  n963 = Greater?(x=w1553, y=10.0) -> (0:w1550:bool)
                  n964 = Compound Arithmetic op=OR(w1547, w1546, w1550, w1549) -> (w1548:bool)
                }
              }
              frame #2 {
                n965 = call "PCI1220U停止.vi"("AxisHandle IN"=w1556) -> ()  [unwired: 9 in, 2 out]
              }
            }
          }
        }
      }
      frame #7 {
        n966 = local read "齿条推拉力(N)"() -> (w1561:dbl)
        n967 = local read "电动缸前进"() -> (w1558:bool)
        n968 = local read "电动缸后退"() -> (w1557:bool)
        n969 = Absolute Value(x=w1561) -> (abs(x)=w1565:dbl)
        n970 = local read "黄灯"() -> (w1559:bool)
        n971 = Not(x=w1557) -> (.not. x?=w1562:bool)
        n972 = Less?(x=w1565, y=1000.0) -> (x < y?=w1563:bool)
        n973 = Compound Arithmetic op=AND(w1558, w1562, w1559, w1563) -> (w1560:bool)
        n974 = case shown="真" w1560 {
          frame False {
          }
          frame True {
            n975 = flat-sequence {
              tunnel: [w1569] -> w1567
              tunnel: w1567 -> [w1571]
              tunnel: [w1571] -> w1566
              tunnel: w1566 -> [w1582]
              frame #0 {
                n976 = local read "电动缸电机"() -> (w1568:u32)
                n977 = call "PCI1220U运行.vi"("方向"=enum32{"Negative", "Positive"}."Positive" ("Direction"), "AxisHandle IN"=w1568) -> ("AxisHandle OUT"=w1569:u32)  [unwired: 9 in]
              }
              frame #1 {
                n978 = while {
                  stop <- w1579 stop-if-true
                  n979 = local read "电动缸前进"() -> (w1576:bool)
                  n980 = local read "齿条推拉力(N)"() -> (w1573:dbl)
                  n981 = Wait (ms)(milliseconds to wait=u32 50 ("毫秒倍数")) -> ()  [unwired: 1 out]
                  n982 = Absolute Value(x=w1573) -> (abs(x)=w1575:dbl)
                  n983 = local read "红灯"() -> (w1577:bool)
                  n984 = local read "复位"() -> (w1578:bool)
                  n985 = Greater?(x=w1575, y=1000.0) -> (0:w1572:bool)
                  n986 = Not(x=w1576) -> (.not. x?=w1580:bool)
                  n987 = Compound Arithmetic op=OR(w1578, w1577, w1580, w1572) -> (w1579:bool)
                }
              }
              frame #2 {
                n988 = call "PCI1220U停止.vi"("AxisHandle IN"=w1582) -> ()  [unwired: 9 in, 2 out]
              }
            }
          }
        }
      }
      frame #8 {
        n989 = local read "电动缸前进"() -> (w1583:bool)
        n990 = local read "齿条推拉力(N)"() -> (w1587:dbl)
        n991 = local read "电动缸后退"() -> (w1584:bool)
        n992 = Absolute Value(x=w1587) -> (abs(x)=w1591:dbl)
        n993 = local read "黄灯"() -> (w1585:bool)
        n994 = Not(x=w1583) -> (.not. x?=w1588:bool)
        n995 = Less?(x=w1591, y=1000.0) -> (x < y?=w1589:bool)
        n996 = Compound Arithmetic op=AND(w1584, w1588, w1585, w1589) -> (w1586:bool)
        n997 = case shown="真" w1586 {
          frame False {
          }
          frame True {
            n998 = flat-sequence {
              tunnel: [w1595] -> w1593
              tunnel: w1593 -> [w1597]
              tunnel: [w1597] -> w1592
              tunnel: w1592 -> [w1608]
              frame #0 {
                n999 = local read "电动缸电机"() -> (w1594:u32)
                n1000 = call "PCI1220U运行.vi"("方向"=enum32{"Negative", "Positive"}."Negative" ("Direction"), "AxisHandle IN"=w1594) -> ("AxisHandle OUT"=w1595:u32)  [unwired: 9 in]
              }
              frame #1 {
                n1001 = while {
                  stop <- w1605 stop-if-true
                  n1002 = local read "电动缸后退"() -> (w1602:bool)
                  n1003 = local read "齿条推拉力(N)"() -> (w1601:dbl)
                  n1004 = Wait (ms)(milliseconds to wait=u32 50 ("毫秒倍数")) -> ()  [unwired: 1 out]
                  n1005 = Absolute Value(x=w1601) -> (abs(x)=w1599:dbl)
                  n1006 = local read "红灯"() -> (w1604:bool)
                  n1007 = local read "复位"() -> (w1603:bool)
                  n1008 = Greater?(x=w1599, y=1000.0) -> (0:w1598:bool)
                  n1009 = Not(x=w1602) -> (.not. x?=w1606:bool)
                  n1010 = Compound Arithmetic op=OR(w1603, w1604, w1606, w1598) -> (w1605:bool)
                }
              }
              frame #2 {
                n1011 = call "PCI1220U停止.vi"("AxisHandle IN"=w1608) -> ()  [unwired: 9 in, 2 out]
              }
            }
          }
        }
      }
      frame #9 {
        n1012 = local read "测头机构轴后退"() -> (w1609:bool)
        n1013 = local read "测头机构轴前进"() -> (w1610:bool)
        n1014 = local read "黄灯"() -> (w1611:bool)
        n1015 = Not(x=w1609) -> (.not. x?=w1613:bool)
        n1016 = Compound Arithmetic op=AND(w1610, w1613, w1611) -> (w1612:bool)
        n1017 = case shown="真" w1612 {
          frame False {
          }
          frame True {
            n1018 = flat-sequence {
              tunnel: [w1617] -> w1615
              tunnel: w1615 -> [w1619]
              tunnel: [w1619] -> w1614
              tunnel: w1614 -> [w1626]
              frame #0 {
                n1019 = local read "测头机构电机"() -> (w1616:u32)
                n1020 = call "PCI1220U运行.vi"("方向"=enum32{"Negative", "Positive"}."Positive" ("Direction"), "AxisHandle IN"=w1616) -> ("AxisHandle OUT"=w1617:u32)  [unwired: 9 in]
              }
              frame #1 {
                n1021 = while {
                  stop <- w1623 stop-if-true
                  n1022 = local read "测头机构轴前进"() -> (w1620:bool)
                  n1023 = Wait (ms)(milliseconds to wait=u32 50 ("毫秒倍数")) -> ()  [unwired: 1 out]
                  n1024 = local read "红灯"() -> (w1621:bool)
                  n1025 = local read "复位"() -> (w1622:bool)
                  n1026 = Not(x=w1620) -> (.not. x?=w1624:bool)
                  n1027 = Compound Arithmetic op=OR(w1622, w1621, w1624) -> (w1623:bool)
                }
              }
              frame #2 {
                n1028 = call "PCI1220U停止.vi"("AxisHandle IN"=w1626) -> ()  [unwired: 9 in, 2 out]
              }
            }
          }
        }
      }
      frame #10 {
        n1029 = local read "测头机构轴前进"() -> (w1627:bool)
        n1030 = local read "测头机构轴后退"() -> (w1628:bool)
        n1031 = local read "黄灯"() -> (w1629:bool)
        n1032 = Not(x=w1627) -> (.not. x?=w1631:bool)
        n1033 = Compound Arithmetic op=AND(w1628, w1631, w1629) -> (w1630:bool)
        n1034 = case shown="真" w1630 {
          frame False {
          }
          frame True {
            n1035 = flat-sequence {
              tunnel: [w1635] -> w1633
              tunnel: w1633 -> [w1637]
              tunnel: [w1637] -> w1632
              tunnel: w1632 -> [w1644]
              frame #0 {
                n1036 = local read "测头机构电机"() -> (w1634:u32)
                n1037 = call "PCI1220U运行.vi"("方向"=enum32{"Negative", "Positive"}."Negative" ("Direction"), "AxisHandle IN"=w1634) -> ("AxisHandle OUT"=w1635:u32)  [unwired: 9 in]
              }
              frame #1 {
                n1038 = while {
                  stop <- w1641 stop-if-true
                  n1039 = local read "测头机构轴后退"() -> (w1638:bool)
                  n1040 = Wait (ms)(milliseconds to wait=u32 50 ("毫秒倍数")) -> ()  [unwired: 1 out]
                  n1041 = local read "红灯"() -> (w1640:bool)
                  n1042 = local read "复位"() -> (w1639:bool)
                  n1043 = Not(x=w1638) -> (.not. x?=w1642:bool)
                  n1044 = Compound Arithmetic op=OR(w1639, w1640, w1642) -> (w1641:bool)
                }
              }
              frame #2 {
                n1045 = call "PCI1220U停止.vi"("AxisHandle IN"=w1644) -> ()  [unwired: 9 in, 2 out]
              }
            }
          }
        }
      }
      frame #11 {
        n1046 = local read "电动缸回零"() -> (w1645:bool)
        n1047 = case shown="真" w1645 {
          frame False {
          }
          frame True {
            n1048 = stacked-sequence {
              frame #0 {
                n1049 = flat-sequence {
                  tunnel: [w1661] -> w1651
                  tunnel: [w1654] -> w1650
                  tunnel: w1651 -> [w1664]
                  tunnel: [w1664] -> w1649
                  tunnel: [w1662] -> w1648
                  tunnel: w1650 -> [w1662]
                  tunnel: w1649 -> [w1666]
                  tunnel: [w1666] -> w1647
                  tunnel: w1648 -> [w1665]
                  tunnel: [w1665] -> w1646
                  tunnel: w1647 -> [w1682]
                  tunnel: w1646 -> [w1681]
                  frame #0 {
                    n1050 = local write "电动缸速度(mm/s)"(15.0 ("电动缸速度(mm/s)")) -> ()
                    n1051 = local write "测头机构轴速度(mm/s)"(10.0 ("电动缸速度(mm/s)")) -> ()
                  }
                  frame #1 {
                    n1052 = local read "测头机构电机"() -> (w1658:u32)
                    n1053 = local read "电动缸电机"() -> (w1655:u32)
                    n1054 = call <userlib>:"Acm_AxHome.vi"("DirMode"=u32 1, "HomeMode"=u32 11, "AxisHandle"=w1655) -> ("AxisHandle"=w1654:u32)  [unwired: 1 in, 2 out]
                    n1055 = call <userlib>:"Acm_AxHome.vi"("DirMode"=u32 0, "HomeMode"=u32 11, "AxisHandle"=w1658) -> ("AxisHandle"=w1661:u32)  [unwired: 1 in, 2 out]
                  }
                  frame #2 {
                    n1056 = Wait Until Next ms Multiple(millisecond multiple=u32 100 ("毫秒倍数")) -> ()  [unwired: 1 out]
                  }
                  frame #3 {
                    n1057 = while {
                      tunnel: w1665 -> [w1673]
                      stop <- w1668 stop-if-true
                      n1058 = call <userlib>:"Acm_AxGetCmdVelocity.vi"("AxisHandle"=w1673) -> ("Velocity"=w1672:dbl)  [unwired: 1 in, 3 out]
                      n1059 = Wait Until Next ms Multiple(millisecond multiple=u32 50 ("毫秒倍数")) -> ()  [unwired: 1 out]
                      n1060 = Equal To 0?(x=w1672) -> (x = 0?=w1667:bool)
                      n1061 = local read "急停"() -> (w1669:bool)
                      n1062 = local read "复位"() -> (w1670:bool)
                      n1063 = Compound Arithmetic op=OR(invert w1669, w1670, w1667) -> (w1668:bool)
                    }
                    n1064 = while {
                      tunnel: w1666 -> [w1680]
                      stop <- w1676 stop-if-true
                      n1065 = call <userlib>:"Acm_AxGetCmdVelocity.vi"("AxisHandle"=w1680) -> ("Velocity"=w1679:dbl)  [unwired: 1 in, 3 out]
                      n1066 = Wait Until Next ms Multiple(millisecond multiple=u32 50 ("毫秒倍数")) -> ()  [unwired: 1 out]
                      n1067 = Equal To 0?(x=w1679) -> (x = 0?=w1677:bool)
                      n1068 = local read "急停"() -> (w1674:bool)
                      n1069 = local read "复位"() -> (w1675:bool)
                      n1070 = Compound Arithmetic op=OR(invert w1674, w1675, w1677) -> (w1676:bool)
                    }
                  }
                  frame #4 {
                    n1071 = call "PCI1220U角度置零.vi"("AxisHandle IN"=w1681) -> ()  [unwired: 10 in, 1 out]
                    n1072 = call "PCI1220U角度置零.vi"("AxisHandle IN"=w1682) -> ()  [unwired: 10 in, 1 out]
                  }
                }
              }
              frame #1 {
                n1073 = flat-sequence {
                  tunnel: [w1694] -> w1689
                  tunnel: w1689 -> [w1696]
                  tunnel: [w1696] -> w1688
                  tunnel: w1688 -> [w1697]
                  tunnel: [w1697] -> w1687
                  tunnel: w1687 -> [w1706]
                  tunnel: [w1705] -> w1684
                  tunnel: w1684 -> [w1708]
                  tunnel: [w1708] -> w1683
                  tunnel: w1683 -> [w1710]
                  tunnel: [w1709] -> w1686
                  tunnel: w1686 -> [w1719]
                  tunnel: [w1719] -> w1685
                  tunnel: w1685 -> [w1727]
                  frame #0 {
                    n1074 = local write "旋转齿条轴速度(°/s)"(5.0 ("电动缸速度(mm/s)")) -> ()
                  }
                  frame #1 {
                    n1075 = local read "旋转齿条电机"() -> (w1691:u32)
                    n1076 = call <userlib>:"Acm_AxHome.vi"("DirMode"=u32 0, "HomeMode"=u32 11, "AxisHandle"=w1691) -> ("AxisHandle"=w1694:u32)  [unwired: 1 in, 2 out]
                  }
                  frame #2 {
                    n1077 = Wait Until Next ms Multiple(millisecond multiple=u32 100 ("毫秒倍数")) -> ()  [unwired: 1 out]
                  }
                  frame #3 {
                    n1078 = while {
                      tunnel: w1697 -> [w1704]
                      stop <- w1698 stop-if-true
                      n1079 = call <userlib>:"Acm_AxGetCmdVelocity.vi"("AxisHandle"=w1704) -> ("Velocity"=w1703:dbl)  [unwired: 1 in, 3 out]
                      n1080 = Wait Until Next ms Multiple(millisecond multiple=u32 50 ("毫秒倍数")) -> ()  [unwired: 1 out]
                      n1081 = Equal To 0?(x=w1703) -> (x = 0?=w1699:bool)
                      n1082 = local read "急停"() -> (w1701:bool)
                      n1083 = local read "复位"() -> (w1700:bool)
                      n1084 = Compound Arithmetic op=OR(invert w1701, w1700, w1699) -> (w1698:bool)
                    }
                  }
                  frame #4 {
                    n1085 = call "PCI1220U角度置零.vi"("AxisHandle IN"=w1706) -> ("AxisHandle OUT"=w1705:u32)  [unwired: 10 in]
                  }
                  frame #5 {
                    n1086 = Wait (ms)(milliseconds to wait=u32 100 ("等待时间（毫秒）")) -> ()  [unwired: 1 out]
                  }
                  frame #6 {
                    n1087 = while {
                      tunnel: [w1717] -> w1709
                      tunnel: w1710 -> [w1715]
                      stop <- w1712 stop-if-true
                      n1088 = call "PCI1220U扭矩轴位置模式.vi"("Distance"=10.0, "AxisHandle IN"=w1715) -> ("AbsSuccess"=w1711:bool, "AxisHandle OUT"=w1717:u32)  [unwired: 8 in]
                      n1089 = Wait Until Next ms Multiple(millisecond multiple=u32 50 ("毫秒倍数")) -> ()  [unwired: 1 out]
                      n1090 = local read "急停"() -> (w1714:bool)
                      n1091 = local read "复位"() -> (w1713:bool)
                      n1092 = Compound Arithmetic op=OR(invert w1714, w1713, w1711) -> (w1712:bool)
                    }
                  }
                  frame #7 {
                    n1093 = while {
                      tunnel: w1719 -> [w1725]
                      stop <- w1720 stop-if-true
                      n1094 = call <userlib>:"Acm_AxGetCmdVelocity.vi"("AxisHandle"=w1725) -> ("Velocity"=w1726:dbl)  [unwired: 1 in, 3 out]
                      n1095 = Wait Until Next ms Multiple(millisecond multiple=u32 50 ("毫秒倍数")) -> ()  [unwired: 1 out]
                      n1096 = Equal To 0?(x=w1726) -> (x = 0?=w1721:bool)
                      n1097 = local read "急停"() -> (w1723:bool)
                      n1098 = local read "复位"() -> (w1722:bool)
                      n1099 = Compound Arithmetic op=OR(w1721, invert w1723, w1722) -> (w1720:bool)
                    }
                  }
                  frame #8 {
                    n1100 = call "PCI1220U角度置零.vi"("AxisHandle IN"=w1727) -> ()  [unwired: 10 in, 1 out]
                  }
                }
              }
              frame #2 {
                n1101 = flat-sequence {
                  frame #0 {
                    n1102 = while {
                      stop <- w1728 stop-if-true
                      n1103 = local read "电动缸回零"() -> (w1735:bool)
                      n1104 = local write "回零完成"(TRUE ("回零完成")) -> ()
                      n1105 = local write "电动缸回零"(FALSE ("电动缸回零")) -> ()
                      n1106 = Wait Until Next ms Multiple(millisecond multiple=u32 50 ("毫秒倍数")) -> ()  [unwired: 1 out]
                      n1107 = Not(x=w1735) -> (.not. x?=w1729:bool)
                      n1108 = local read "急停"() -> (w1730:bool)
                      n1109 = local read "复位"() -> (w1731:bool)
                      n1110 = Compound Arithmetic op=OR(w1729, invert w1730, w1731) -> (w1728:bool)
                    }
                  }
                }
              }
            }
          }
        }
      }
    }
    n1111 = Wait (ms)(milliseconds to wait=u32 50 ("毫秒倍数")) -> ()  [unwired: 1 out]
    n1112 = local read "停止"() -> (w1431:bool)
  }
  n1113 = while {
    stop <- FALSE stop-if-true
    n1114 = Equal?(x="密码", y="jizhuan") -> (x = y?=w1739:bool)
    n1115 = Compound Arithmetic op=AND(w1739, "?") -> (w1737:bool)
    n1116 = case shown="假" w1737 {
      frame False {
        n1117 = property class="Bool (严格)"("DisabledEnum"=T5."Disabled and Grayed Out" ("禁用")) -> ()  [unwired: 2 in, 2 out]
        n1118 = property class="Bool (严格)"("DisabledEnum"=T5."Disabled and Grayed Out" ("禁用")) -> ()  [unwired: 2 in, 2 out]
      }
      frame True {
        n1119 = property class="Bool (严格)"("DisabledEnum"=T5."Enabled" ("禁用")) -> ()  [unwired: 2 in, 2 out]
        n1120 = property class="Bool (严格)"("DisabledEnum"=T5."Enabled" ("禁用")) -> ()  [unwired: 2 in, 2 out]
        n1121 = case shown="真" "?" {
          frame False {
          }
          frame True {
            n1122 = property on="选项卡控件" class="TabCtl (严格)"() -> ("Pages"=w1748:refnum<vi>[])  [unwired: 2 in, 2 out]
            n1123 = for {
              N: 7 -> [_]
              tunnel: w1748 -> [w1750] mode=indexing
              i -> [w1751]
              n1124 = case shown="5" w1751 {
                tunnel: w1750 -> [_ w1753]
                frame 0, Default {
                }
                frame 5 {
                  n1125 = property class="Page"(reference=w1753, "PageVis"=FALSE ("选项卡可见")) -> ()  [unwired: 1 in, 2 out]
                }
              }
            }
          }
        }
        n1126 = case shown="真" "?" {
          frame False {
          }
          frame True {
            n1127 = property on="选项卡控件" class="TabCtl (严格)"() -> ("Pages"=w1754:refnum<vi>[])  [unwired: 2 in, 2 out]
            n1128 = for {
              N: 7 -> [_]
              tunnel: w1754 -> [w1756] mode=indexing
              i -> [w1757]
              n1129 = case shown="5" w1757 {
                tunnel: w1756 -> [_ w1759]
                frame 0, Default {
                }
                frame 5 {
                  n1130 = property class="Page"(reference=w1759, "PageVis"=TRUE ("选项卡可见")) -> ()  [unwired: 1 in, 2 out]
                }
              }
            }
          }
        }
      }
    }
  }
  n1131 = flat-sequence {
    tunnel: [w1763] -> w2
    tunnel: [w1761] -> w1
    tunnel: w2 -> [w1773]
    tunnel: w1 -> [w1772]
    frame #0 {
      n1132 = First Call?() -> (First Call?: T/F=w1760:bool)
      n1133 = case shown="真" w1760 {
        frame False {
        }
        frame True {
          n1134 = while {
            i -> [w1768]
            stop <- w1766 stop-if-true
            w1771 = TRUE ("电动缸使能")
            n1135 = local write "回零完成"(FALSE ("回零完成")) -> ()
            n1136 = local write "测头机构轴使能"(w1771) -> ()
            n1137 = local write "旋转齿条轴使能"(w1771) -> ()
            n1138 = local write "电动缸使能"(w1771) -> ()
            n1139 = Wait Until Next ms Multiple(millisecond multiple=u32 50 ("毫秒倍数")) -> ()  [unwired: 1 out]
            n1140 = Greater Or Equal?(x=w1768, y=30) -> (x >= y?=w1766:bool)
          }
        }
      }
      n1141 = call "ADO Connection Create.vi"() -> ("error out"=w1764:errorcluster, "ADODB._Connection Out"=w1765:refnum<k7>)  [unwired: 10 in]
      n1142 = call "ADO Connection Open.vi"("error in (no error)"=w1764, "ConnectionString"="Provider=Microsoft.Jet.OLEDB.4.0;Data Source=D:\\Q14070-Z060人机界面\\参数\\参数Z060.mdb;Persist Security Info=False;Jet OLEDB:Database Password=1234;", "ADODB._Connection In"=w1765) -> ("error out"=w1761:errorcluster, "ADODB._Connection Out"=w1763:refnum<k7>)  [unwired: 7 in]
    }
    frame #1 {
      n1143 = while {
        tunnel: w1773 -> [w1775]
        tunnel: w1772 -> [w1774]
        stop <- w1779 stop-if-true
        n1144 = Wait (ms)(milliseconds to wait=u32 50 ("等待时间（毫秒）")) -> ()  [unwired: 1 out]
        n1145 = First Call?() -> (First Call?: T/F=w1778:bool)
        n1146 = Or(x=w1778, y="参数加载") -> (x .or. y?=w1777:bool)
        n1147 = case shown="真" w1777 {
          tunnel: w1775 -> [_ w1782]
          tunnel: w1774 -> [_ w1781]
          frame False {
          }
          frame True {
            n1148 = stacked-sequence {
              tunnel: w1782 -> [w1788 w1799 w1857]
              tunnel: w1781 -> [w1783 _ _]
              frame #0 {
                n1149 = call "SQL Execute.vi"("error in (no error)"=w1783, "Command Text"="SELECT * FROM 测试参数表", "ADODB._Connection In"=w1788) -> ("Data"=w1786:string[][])  [unwired: 5 in, 3 out]
                n1150 = Index Array(array=w1786, index (col)=0 ("索引 (行)")) -> (element=w1790:string[])  [unwired: 1 in]
                n1151 = Array Size(array=w1790) -> (size(s)=w1785:i32)
                "型号数量" <- w1785
                n1152 = while {
                  shift-right: [w1797] -> w1789
                  shift-left: i32[] [] -> [w1796]
                  tunnel: w1785 -> [w1794]
                  i -> [w1795]
                  stop <- w1793 stop-if-true
                  n1153 = Greater Or Equal?(x=w1795, y=w1794) -> (x >= y?=w1793:bool)
                  n1154 = Build Array (concatenate)(w1796, w1795) -> (w1797:i32[])
                }
                n1155 = Build Cluster Array "索引与捆绑簇数组"(w1790, w1789) -> (w1784:cluster{"String":string, i32}[])
                n1156 = property on="型号选择" class="Ring (严格)"("StringsAndValues[]"=w1784) -> ()  [unwired: 2 in, 2 out]
              }
              frame #1 {
                n1157 = property on="型号选择" class="Ring (严格)"() -> ("RingText.Text"=w1800:string)  [unwired: 2 in, 2 out]
                n1158 = call "创建文本2"("型号选择"=w1800) -> ("Result"=w1804:string)  [unwired: 13 in, 1 out]
                n1159 = call "SQL Execute.vi"("Command Text"=w1804, "ADODB._Connection In"=w1799) -> ("Data"=w1803:string[][])  [unwired: 6 in, 3 out]
                n1160 = Index Array(array=w1803, index (row)=0 ("索引 (行)")) -> (element=w1801:string[])  [unwired: 1 in]
                n1161 = Fract/Exp String To Number ("分数/指数字符串至数值转换")(string=w1801) -> (number=w1798:dbl[])  [unwired: 3 in, 1 out]
                n1162 = stacked-sequence {
                  tunnel: w1798 -> [w1833]
                  frame #0 {
                    n1163 = Index Array ("索引数组")(array=w1833, index #1=2 ("索引"), index #2=3 ("索引"), index #3=4 ("索引"), index #4=5 ("索引"), index #5=6 ("索引"), index #6=7 ("索引"), index #7=8 ("索引"), index #8=9 ("索引"), index #9=10 ("索引"), index #10=11 ("索引"), index #11=12 ("索引"), index #12=13 ("索引"), index #13=14 ("索引"), index #14=15 ("索引"), index #15=16 ("索引"), index #16=17 ("索引"), index #17=18 ("索引"), index #18=19 ("索引"), index #19=20 ("索引")) -> (element #1=w1832:dbl, element #2=w1831:dbl, element #3=w1830:dbl, element #4=w1829:dbl, element #5=w1828:dbl, element #6=w1827:dbl, element #7=w1826:dbl, element #8=w1825:dbl, element #9=w1824:dbl, element #10=w1823:dbl, element #11=w1816:dbl, element #12=w1815:dbl, element #13=→"齿条传动比":dbl, element #14=→"力波动标准(N)":dbl, element #15=→"轴向力标准(N)":dbl, element #16=→"平均轴向力标准(N) max":dbl, element #17=→"总圈数标准":dbl, element #18=→"总圈数最大值":dbl, element #19=w1811:dbl)
                    n1164 = local write "测头机构轴移动速度"(w1832) -> ()
                    n1165 = local write "测头机构轴检测位"(w1831) -> ()
                    n1166 = local write "测头机构轴后退位"(w1829) -> ()
                    n1167 = local write "测头机构轴待检位"(w1830) -> ()
                    n1168 = local write "旋转齿条轴找帽转速"(w1825) -> ()
                    n1169 = local write "旋转齿条轴测量转速"(w1824) -> ()
                    n1170 = local write "转向器中心"(w1811) -> ()
                    n1171 = local write "总行程标准(mm)"(w1816) -> ()
                    n1172 = local write "齿条移动速度"(w1828) -> ()
                    n1173 = local write "齿条左极限"(w1827) -> ()
                    n1174 = local write "齿条右极限"(w1826) -> ()
                    n1175 = local write "总行程最大值"(w1815) -> ()
                    n1176 = local write "测量点扭矩"(w1823) -> ()
                  }
                }
              }
              frame #2 {
                n1177 = call "SQL Execute.vi"("Command Text"="SELECT * FROM 传感器校验表 where ID='1'", "ADODB._Connection In"=w1857) -> ("Data"=w1859:string[][])  [unwired: 6 in, 3 out]
                n1178 = Index Array(array=w1859) -> (element=w1860:string[])  [unwired: 2 in]
                n1179 = Fract/Exp String To Number ("分数/指数字符串至数值转换")(string=w1860) -> (number=w1850:dbl[])  [unwired: 3 in, 1 out]
                n1180 = Index Array(array=w1850, index #1=1 ("索引"), index #2=2 ("索引"), index #3=3 ("索引"), index #4=4 ("索引"), index #5=5 ("索引"), index #6=6 ("索引")) -> (element #1=w1849:dbl, element #2=w1848:dbl, element #3=w1847:dbl, element #4=w1846:dbl, element #5=w1845:dbl, element #6=w1844:dbl)
                n1181 = local write "间隙位移零点偏移"(w1849) -> ()
                n1182 = local write "间隙位移比例偏移"(w1848) -> ()
                n1183 = local write "齿条推拉力零点偏移"(w1847) -> ()
                n1184 = local write "齿条推拉力比例偏移"(w1846) -> ()
                n1185 = local write "齿条扭矩零点偏移"(w1845) -> ()
                n1186 = local write "齿条扭矩比例偏移"(w1844) -> ()
              }
            }
          }
        }
        n1187 = local read "停止"() -> (w1779:bool)
        "ADODB._Connection Out 2" <- w1775
      }
    }
  }
  n1188 = while {
    stop <- w1862 stop-if-true
    n1189 = local read "rfid工步号"() -> (w1861:u32)
    n1190 = case shown="10" w1861 {
      frame 0, Default {
      }
      frame 10 {
        n1191 = flat-sequence {
          tunnel: [w1872] -> w1866
          tunnel: w1866 -> [w1874]
          tunnel: [w1873] -> w1865
          tunnel: w1865 -> [w1876]
          tunnel: [w1876] -> w1864
          tunnel: w1864 -> [w1879]
          frame #0 {
            n1192 = while {
              stop <- w1867 stop-if-true
              n1193 = local read "rfid触发"() -> (w1867:bool)
              n1194 = Wait Until Next ms Multiple(millisecond multiple=u32 50 ("毫秒倍数")) -> ()  [unwired: 1 out]
            }
          }
          frame #1 {
            n1195 = local write "芯片ID"("" ("随行板ID")) -> ()
            n1196 = local write "rfid完成"(FALSE ("RFID完成")) -> ()
            n1197 = local write "rfid触发"(FALSE ("RFID读取触发")) -> ()
          }
          frame #2 {
            n1198 = local read "Z060BRFID"() -> (w1872:string)
            n1199 = local write "芯片ID"(w1872) -> ()
          }
          frame #3 {
            n1200 = call "查询产品ID.vi"("芯片编码"=w1874) -> ("产品ID"=w1873:string)  [unwired: 8 in, 2 out]
            "读取产品ID" <- w1873
          }
          frame #4 {
            n1201 = Wait (ms)(milliseconds to wait=u32 500 ("等待时间（毫秒）")) -> ()  [unwired: 1 out]
          }
          frame #5 {
            n1202 = call "查询上序合格.vi"("产品ID"=w1879) -> ("本序已做"=w1877:bool, "上序合格"=w1878:bool)  [unwired: 8 in, 1 out]
            n1203 = Not(x=w1878) -> (.not. x?=w1880:bool)
            n1204 = local write "上序合格"(w1878) -> ()
            n1205 = local write "本序已做"(w1877) -> ()
            n1206 = local write "上序不合格"(w1880) -> ()
          }
          frame #6 {
            n1207 = local write "rfid完成"(TRUE ("RFID读取完成")) -> ()
            n1208 = Wait Until Next ms Multiple(millisecond multiple=u32 500 ("毫秒倍数")) -> ()  [unwired: 1 out]
          }
          frame #7 {
            "rfid工步号" <- 15.0 ("工步号")
          }
        }
      }
      frame 210 {
        n1209 = local read "读取产品ID"() -> (w1884:string)
        n1210 = local write "产品ID"(w1884) -> ()
      }
    }
    n1211 = Wait Until Next ms Multiple(millisecond multiple=u32 50 ("毫秒倍数")) -> ()  [unwired: 1 out]
    n1212 = local read "停止"() -> (w1862:bool)
  }
  n1213 = flat-sequence {
    tunnel: [w1885] -> w4
    tunnel: w4 -> [w1891]
    tunnel: [w1890] -> w3
    tunnel: w3 -> [w1961]
    frame #0 {
      n1214 = call "PCI1240U初始化.vi"() -> ("旋转电机"=→"旋转齿条电机":u32, "电动缸电机"=→"电动缸电机":u32, "DeviceHandle"=→"DeviceHandle":u32, "进给电机"=→"测头机构电机":u32)  [unwired: 6 in, 2 out]
      n1215 = call "PCI8622配置.vi"() -> ("DeviceID"=w1885:i32)  [unwired: 11 in]
    }
    frame #1 {
      n1216 = while {
        tunnel: w1891 -> [w1893]
        tunnel: [w1892] -> w1890
        stop <- "停止" stop-if-true
        n1217 = stacked-sequence {
          tunnel: w1893 -> [_ _ w1937]
          tunnel: [_ _ w1937] -> w1892
          frame #0 {
            n1218 = local read "测头机构电机"() -> (w1902:u32)
            n1219 = Boolean To (0,1)(Boolean="测头机构轴使能") -> (0, 1=w1900:i16)
            n1220 = call <userlib>:"Acm_AxSetSvOn.vi"("OnOff"=w1900, "AxisHandle"=w1902) -> ("AxisHandle"=w1899:u32)  [unwired: 1 in, 2 out]
            n1221 = call "PCI1220U进给轴速度设置.vi"("Change Velocity"="测头机构轴速度(mm/s)", "AxisHandle IN"=w1899) -> ("AxisHandle OUT"=w1897:u32)  [unwired: 9 in]
            n1222 = call "PCI1220U进给轴读取位置.vi"("AxisHandle IN"=w1897) -> ("位置"=→"测头机构轴位置(mm)":dbl)  [unwired: 9 in, 1 out]
          }
          frame #1 {
            n1223 = local read "电动缸电机"() -> (w1912:u32)
            n1224 = local read "旋转齿条电机"() -> (w1911:u32)
            n1225 = Boolean To (0,1)(Boolean="电动缸使能") -> (0, 1=w1916:i16)
            n1226 = Boolean To (0,1)(Boolean="旋转齿条轴使能") -> (0, 1=w1910:i16)
            n1227 = call <userlib>:"Acm_AxSetSvOn.vi"("OnOff"=w1910, "AxisHandle"=w1911) -> ("AxisHandle"=w1913:u32)  [unwired: 1 in, 2 out]
            n1228 = call <userlib>:"Acm_AxSetSvOn.vi"("OnOff"=w1916, "AxisHandle"=w1912) -> ("AxisHandle"=w1915:u32)  [unwired: 1 in, 2 out]
            n1229 = call "PCI1220U扭矩轴速度设置.vi"("Change Velocity"="旋转齿条轴速度(°/s)", "AxisHandle IN"=w1913) -> ("AxisHandle OUT"=w1914:u32)  [unwired: 9 in]
            n1230 = call "PCI1240电动缸速度设置.vi"("Change Velocity"="电动缸速度(mm/s)", "AxisHandle IN"=w1915) -> ("AxisHandle OUT"=w1903:u32)  [unwired: 9 in]
            n1231 = call "PCI1220U扭矩轴读取位置.vi"("AxisHandle IN"=w1914) -> ("位置"=→"旋转齿条轴位置(°)":dbl)  [unwired: 9 in, 1 out]
            n1232 = call "PCI1240电动缸读取位置.vi"("AxisHandle IN"=w1903) -> ("位置"=→"电动缸位置(mm)":dbl)  [unwired: 9 in, 1 out]
          }
          frame #2 {
            w1953 = 0  # nRetSizeWords
            w1954 = 2048  # nReadSizeWords
            # "hDevice"
            n1233 = Initialize Array(u16 0, 2048 ("dimension size")) -> (w1944:u16[])
            n1234 = dll-call lib="PCI8622_32.dll" fn="PCI8622_ReadDeviceProAD_Npt" label="ReadDeviceProAD_Npt"("hDevice"=w1937, "ADBuffer[]"=w1944, "nReadSizeWords"=w1954, "nRetSizeWords"=w1953) -> ("ADBuffer[]"=w1947:u16[])  [unwired: 7 in, 2 out]
            n1235 = Divide(x=w1947, y=65536.01) -> (x/y=w1948:dbl[])
            n1236 = Multiply(x=w1948, y=20) -> (x*y=w1951:dbl[])
            n1237 = Subtract(x=w1951, y=10) -> (x-y=w1943:dbl[])
            n1238 = Decimate 1D Array ("抽取一维数组")(w1943) -> (w1931:dbl[], w1932:dbl[], w1930:dbl[])  [unwired: 5 out]
            n1239 = Add Array Elements(numeric array=w1930) -> (sum=w1941:dbl)
            n1240 = Array Size(array=w1930) -> (size(s)=w1942:i32)
            n1241 = Divide(x=w1941, y=w1942) -> (x/y=w1923:dbl)
            n1242 = Divide(x=w1923, y=5.86) -> (x/y=w1920:dbl)
            n1243 = Multiply(x=4.0, y=w1920) -> (x*y=w1918:dbl)
            n1244 = Add Array Elements(numeric array=w1931) -> (sum=w1940:dbl)
            n1245 = Array Size(array=w1931) -> (size(s)=w1939:i32)
            n1246 = Add Array Elements(numeric array=w1932) -> (sum=w1936:dbl)
            n1247 = Array Size(array=w1932) -> (size(s)=w1938:i32)
            n1248 = Divide(x=w1940, y=w1939) -> (x/y=w1929:dbl)
            n1249 = Divide(x=w1936, y=w1938) -> (x/y=w1926:dbl)
            n1250 = Multiply(x=w1929, y=2.0) -> (x*y=w1924:dbl)
            n1251 = Multiply(x=w1926, y=200.0) -> (x*y=w1925:dbl)
            n1252 = Subtract(x=w1918, y=0.675) -> (x-y=w1921:dbl)
            n1253 = local read "间隙位移比例偏移"() -> (w1958:dbl)
            n1254 = local read "间隙位移零点偏移"() -> (w1957:dbl)
            n1255 = local read "齿条扭矩零点偏移"() -> (w1959:dbl)
            n1256 = local read "齿条扭矩比例偏移"() -> (w1960:dbl)
            n1257 = local read "齿条推拉力比例偏移"() -> (w1956:dbl)
            n1258 = local read "齿条推拉力零点偏移"() -> (w1955:dbl)
            n1259 = call "传感器校订.vi"("零点"=w1959, "比例"=w1960, "传感器"=w1924) -> ("示值"=→"齿条扭矩(Nm)":dbl)  [unwired: 8 in]
            n1260 = call "传感器校订.vi"("零点"=w1957, "比例"=w1958, "传感器"=w1921) -> ("示值"=→"间隙位移(mm)":dbl)  [unwired: 8 in]
            n1261 = call "传感器校订.vi"("零点"=w1955, "比例"=w1956, "传感器"=w1925) -> ("示值"=→"齿条推拉力(N)":dbl)  [unwired: 8 in]
          }
        }
        n1262 = Wait Until Next ms Multiple(millisecond multiple=u32 50 ("毫秒倍数")) -> ()  [unwired: 1 out]
      }
    }
    frame #2 {
      n1263 = dll-call lib="PCI8622_32.dll" fn="PCI8622_StopDeviceProAD" label="StopDeviceProAD"("hDevice"=w1961) -> ("hDevice"=w1962:i32)  [unwired: 4 in, 2 out]
      n1264 = dll-call lib="PCI8622_32.dll" fn="PCI8622_ReleaseDeviceProAD" label="ReleaseDeviceProAD"("hDevice"=w1962) -> ()  [unwired: 5 in, 2 out]
      n1265 = dll-call lib="PCI8622_32.dll" fn="PCI8622_ReleaseDevice" label="ReleaseDevice"("hDevice"=w1961) -> ()  [unwired: 5 in, 2 out]
    }
  }
